vi "TC-4.59.22-backup.vi"() -> ()   [LabVIEW 2019]
uses:
  1. Sources/Lib/Lib.llb/CS mode.ctl
  1. Sources/Lib/Lib.llb/R.ctl
  1. Sources/Lib/Lib.llb/T.ctl
  1. Sources/Lib/Lib.llb/Calibrations.ctl
  1. Sources/Lib/Lib.llb/CS.lvclass
  1. Sources/Lib/Lib.llb/PID Settings.ctl
  1. Sources/Lib/Lib.llb/AVS_exc_n_ranges.ctl
  1. Sources/Lib/Lib.llb/AVS_excitation.ctl
  1. Sources/Lib/Lib.llb/AVS47_range.ctl
  1. Sources/Lib/Lib.llb/Ch descriptions.ctl
  1. Sources/Lib/Lib.llb/Cursor Controls.ctl
  1. Sources/Lib/Lib.llb/DataArray.ctl
  1. Sources/Lib/Lib.llb/Unit.ctl
  1. Sources/Lib/Lib.llb/Control 6.ctl
  1. Sources/Lib/Lib.llb/Control 4.ctl
  1. Sources/Lib/Lib.llb/Control 8.ctl
  1. Sources/Lib/Lib.llb/VI FPO Ref.ctl
  1. Sources/Lib/support/Class ID ENUM.ctl
  <userlib>/_OpenG.lib/lvdata/lvdata.llb/Type Descriptor Enumeration__ogtk.ctl
  <userlib>/_OpenG.lib/lvdata/lvdata.llb/Refnum Subtype Enum__ogtk.ctl
  <userlib>/_OpenG.lib/lvdata/lvdata.llb/Waveform Subtype Enum__ogtk.ctl
  1. Sources/Lib/Lib.llb/LV Data cluster.ctl
  1. Sources/Lib/Lib.llb/Action.ctl
  1. Sources/Lib/Lib.llb/TCS.lvclass
  C:/Users/patrick/Documents/GitHub/Leiden-FP-and-TC/src/TC/1. Sources/Lib/Lib.llb/CS.lvclass
  1. Sources/Lib/Lib.llb/QCS.lvclass
  1. Sources/Lib/Lib.llb/CS Emulation.lvclass
  1. Sources/Lib/Lib.llb/PCS.lvclass
  1. Sources/Lib/Lib.llb/Byte Params.ctl
  1. Sources/Lib/Lib.llb/MView.lvlib
  shared/FP-TC-Shared/FP-TC-Shared.lvclass
panel:
  out "R Array":dbl[](array[numeric])
  out "_SetControl":T1
  out "ControlNames":string[](array[string])
  out "VIRef":T2 {"Array DataType" format="%.0x"; "WaveForm Type" format="%.0x"; "RefNum Type" format="%.0x"; "DataType" format="%.0x"}
  out "VI called?":bool=TRUE
  out "Error code":u8
  out "_zBridgeSetNr":u8 caption="zBridge set nr."
  out "_zBridgeDll":path=path "C:/Users/Sasha/Dropbox/Labview/LC Software/ImpSoft-V5.2.2-multithreaded/ImpBridgeLabview/ImpBridgeDll.dll"
  in  "_String":string="^ Click the Run button to start the program "
  in  "Top Toolbar":enum32{"Page 1", "Page 2"}(tab)
  in  "Load config":bool
  in  "Start":bool
  in  "Load Data":bool
  in  "Pause":bool
  in  "Stop":bool
  in  "Copy to Clipboard":bool
  in  "Save config":bool
  in  "Clear all plots":bool
  in  "ColorBox":enum32{"Page 1", "Page 2"}(tab)
  in  "Colors":picture
  out "Color":u32(colorbox)
  in  "Graph-open popup":bool
  out "_CalibFilesPath":path=path "C:/avs-47/aaaa"
  out "_LogFilesPath":path
  out "_AVS_VISA":refnum<visa-resource-name>="COM3"
  out "VI Version":string="TC" caption="V"
  in  "Minimize UI 2":bool
  in  "Minimize UI 1":bool
  in  "Main Panel":enum32{"AVS"}(tab)
  in  "Graph Controls Bar":enum32{"Page 1"}(tab)
  in  "Mode Buttons":T7
  in  "Erase all":bool
  in  "Plot-Save All":bool
  in  "Plot-save-screen":bool
  in  "Channels Panel":T8(tab)=enum."All"
  out "T0":dbl=nan caption="T" format="%#.2p"
  out "R0":dbl caption="R" format="%.3p"
  out "R-Plot 0":cluster{dbl[], dbl[]}(graph) caption="R-Plot"
  out "T1":dbl=nan caption="T" format="%#.2p"
  out "R1":dbl caption="R" format="%.3p"
  out "R-Plot 1":cluster{dbl[], dbl[]}(graph) caption="R-Plot"
  out "T2":dbl=nan caption="T" format="%#.2p"
  out "R2":dbl caption="R" format="%.3p"
  out "R-Plot 2":cluster{dbl[], dbl[]}(graph) caption="R-Plot"
  out "T3":dbl=nan caption="T" format="%#.2p"
  out "R3":dbl caption="R" format="%.3p"
  out "R-Plot 3":cluster{dbl[], dbl[]}(graph) caption="R-Plot"
  out "T4":dbl=nan caption="T" format="%#.2p"
  out "R4":dbl caption="R" format="%.3p"
  out "R-Plot 4":cluster{dbl[], dbl[]}(graph) caption="R-Plot"
  out "T5":dbl=nan caption="T" format="%#.2p"
  out "R5":dbl caption="R" format="%.3p"
  out "R-Plot 5":cluster{dbl[], dbl[]}(graph) caption="R-Plot"
  out "T6":dbl=nan caption="T" format="%#.2p"
  out "R6":dbl caption="R" format="%.3p"
  out "R-Plot 6":cluster{dbl[], dbl[]}(graph) caption="R-Plot"
  out "T7":dbl=nan caption="T" format="%#.2p"
  out "R7":dbl caption="R" format="%.3p"
  out "R-Plot 7":cluster{dbl[], dbl[]}(graph) caption="R-Plot"
  out "T8":dbl=nan caption="T" format="%#.2p"
  out "R8":dbl caption="R" format="%.3p"
  out "R-Plot 8":cluster{dbl[], dbl[]}(graph) caption="R-Plot"
  out "T9":dbl=nan caption="T" format="%#.2p"
  out "R9":dbl caption="R" format="%.3p"
  out "R-Plot 9":cluster{dbl[], dbl[]}(graph) caption="R-Plot"
  out "T Cluster":T9 {"T9" format="%.2p"; "T8" format="%.2p"; "T7" format="%.2p"; "T6" format="%.2p"; "T5" format="%.2p"; "T4" format="%.2p"; "T3" format="%.2p"; "T2" format="%.2p"; "T1" format="%.2p"; "T0" format="%.2p"}
  in  "Sensor Names":T10={"AVS Name 0"="C_still", "AVS Name 1"="3K", "AVS Name 2"="Still", "AVS Name 3"="50mK", "AVS Name 4"="MC", "AVS Name 5"="MC", "AVS Name 6"="MC", "AVS Name 7"="", "AVS Name 8"="", "AVS Name 9"=""}
  in  "Edit Calibrations":T11
  in  "Sensor Calibrations":T12 {"Sensor 10" items=["magnet", "No Calibration", "PT100", "PT1000", "RuO2 10k", "RuO2 1k5", "RuO2 2k", "switch", "Emulation R", "PT 1000", "RuO2-10K-NEW", "RuO2-10K", "RuO2-1k5", "TT-1338", "TT-1340", "TT-1342", "TT-1346", "TT-1349", "TT-1392", "CMN-187", "testCMN", "No Calibration"]; "Sensor 9" items=["magnet", "No Calibration", "PT100", "PT1000", "RuO2 10k", "RuO2 1k5", "RuO2 2k", "switch", "Emulation R", "PT 1000", "RuO2-10K-NEW", "RuO2-10K", "RuO2-1k5", "TT-1338", "TT-1340", "TT-1342", "TT-1346", "TT-1349", "TT-1392", "CMN-187", "testCMN", "No Calibration"]; "Sensor 8" items=["magnet", "No Calibration", "PT100", "PT1000", "RuO2 10k", "RuO2 1k5", "RuO2 2k", "switch", "Emulation R", "PT 1000", "RuO2-10K-NEW", "RuO2-10K", "RuO2-1k5", "TT-1338", "TT-1340", "TT-1342", "TT-1346", "TT-1349", "TT-1392", "CMN-187", "testCMN", "No Calibration"]; "Sensor 7" items=["magnet", "No Calibration", "PT100", "PT1000", "RuO2 10k", "RuO2 1k5", "RuO2 2k", "switch", "Emulation R", "PT 1000", "RuO2-10K-NEW", "RuO2-10K", "RuO2-1k5", "TT-1338", "TT-1340", "TT-1342", "TT-1346", "TT-1349", "TT-1392", "CMN-187", "testCMN", "No Calibration"]; "Sensor 6" items=["magnet", "No Calibration", "PT100", "PT1000", "RuO2 10k", "RuO2 1k5", "RuO2 2k", "switch", "Emulation R", "PT 1000", "RuO2-10K-NEW", "RuO2-10K", "RuO2-1k5", "TT-1338", "TT-1340", "TT-1342", "TT-1346", "TT-1349", "TT-1392", "CMN-187", "testCMN", "No Calibration"]; "Sensor 5" items=["magnet", "No Calibration", "PT100", "PT1000", "RuO2 10k", "RuO2 1k5", "RuO2 2k", "switch", "Emulation R", "PT 1000", "RuO2-10K-NEW", "RuO2-10K", "RuO2-1k5", "TT-1338", "TT-1340", "TT-1342", "TT-1346", "TT-1349", "TT-1392", "CMN-187", "testCMN", "No Calibration"]; "Sensor 4" items=["magnet", "No Calibration", "PT100", "PT1000", "RuO2 10k", "RuO2 1k5", "RuO2 2k", "switch", "Emulation R", "PT 1000", "RuO2-10K-NEW", "RuO2-10K", "RuO2-1k5", "TT-1338", "TT-1340", "TT-1342", "TT-1346", "TT-1349", "TT-1392", "CMN-187", "testCMN", "No Calibration"]; "Sensor 3" items=["magnet", "No Calibration", "PT100", "PT1000", "RuO2 10k", "RuO2 1k5", "RuO2 2k", "switch", "Emulation R", "PT 1000", "RuO2-10K-NEW", "RuO2-10K", "RuO2-1k5", "TT-1338", "TT-1340", "TT-1342", "TT-1346", "TT-1349", "TT-1392", "CMN-187", "testCMN", "No Calibration"]; "Sensor 2" items=["magnet", "No Calibration", "PT100", "PT1000", "RuO2 10k", "RuO2 1k5", "RuO2 2k", "switch", "Emulation R", "PT 1000", "RuO2-10K-NEW", "RuO2-10K", "RuO2-1k5", "TT-1338", "TT-1340", "TT-1342", "TT-1346", "TT-1349", "TT-1392", "CMN-187", "testCMN", "No Calibration"]; "Sensor 1" items=["magnet", "No Calibration", "PT100", "PT1000", "RuO2 10k", "RuO2 1k5", "RuO2 2k", "switch", "Emulation R", "PT 1000", "RuO2-10K-NEW", "RuO2-10K", "RuO2-1k5", "TT-1338", "TT-1340", "TT-1342", "TT-1346", "TT-1349", "TT-1392", "CMN-187", "testCMN", "No Calibration"]}
  out "Units":T13
  out "R Cluster":T14={"R0"=0.0, "R1"=0.0, "R2"=-0.0, "R3"=0.0, "R4"=0.0, "R5"=0.0, "R6"=0.0, "R7"=0.0, "R8"=0.0, "R9"=0.0} {"R9" format="%.3p"; "R8" format="%.3p"; "R7" format="%.3p"; "R6" format="%.3p"; "R5" format="%.3p"; "R4" format="%.3p"; "R3" format="%.3p"; "R2" format="%.3p"; "R1" format="%.3p"; "R0" format="%.3p"}
  in  "AVS Scan Parameters":enum32{"Page 1", "Page 2"}(tab)
  in  "AVS Exc&Ranges":T15={"Excitation 0"=4, "Excitation 1"=4, "Excitation 2"=3, "Excitation 3"=3, "Excitation 4"=3, "Excitation 5"=3, "Excitation 6"=3, "Excitation 7"=3, "Range 0"=5, "Range 1"=5, "Range 2"=5, "Range 3"=5, "Range 4"=5, "Range 5"=5, "Range 6"=5, "Range 7"=5} {"Range 7" items=["n.a."=-1, "open"=0, "2 Ohm"=1, "20 Ohm"=2, "200 Ohm"=3, "2k Ohm"=4, "20k Ohm"=5, "200k Ohm"=6, "2M Ohm"=7]; "Range 6" items=["n.a."=-1, "open"=0, "2 Ohm"=1, "20 Ohm"=2, "200 Ohm"=3, "2k Ohm"=4, "20k Ohm"=5, "200k Ohm"=6, "2M Ohm"=7]; "Range 5" items=["n.a."=-1, "open"=0, "2 Ohm"=1, "20 Ohm"=2, "200 Ohm"=3, "2k Ohm"=4, "20k Ohm"=5, "200k Ohm"=6, "2M Ohm"=7]; "Range 4" items=["n.a."=-1, "open"=0, "2 Ohm"=1, "20 Ohm"=2, "200 Ohm"=3, "2k Ohm"=4, "20k Ohm"=5, "200k Ohm"=6, "2M Ohm"=7]; "Range 3" items=["n.a."=-1, "open"=0, "2 Ohm"=1, "20 Ohm"=2, "200 Ohm"=3, "2k Ohm"=4, "20k Ohm"=5, "200k Ohm"=6, "2M Ohm"=7]; "Range 2" items=["n.a."=-1, "open"=0, "2 Ohm"=1, "20 Ohm"=2, "200 Ohm"=3, "2k Ohm"=4, "20k Ohm"=5, "200k Ohm"=6, "2M Ohm"=7]; "Range 1" items=["n.a."=-1, "open"=0, "2 Ohm"=1, "20 Ohm"=2, "200 Ohm"=3, "2k Ohm"=4, "20k Ohm"=5, "200k Ohm"=6, "2M Ohm"=7]; "Range 0" items=["n.a."=-1, "open"=0, "2 Ohm"=1, "20 Ohm"=2, "200 Ohm"=3, "2k Ohm"=4, "20k Ohm"=5, "200k Ohm"=6, "2M Ohm"=7]; "Excitation 7" items=["none", "3 µV", "10 µV", "30 µV", "100 µV", "300 µV", "1 mV", "3 mV"]; "Excitation 6" items=["none", "3 µV", "10 µV", "30 µV", "100 µV", "300 µV", "1 mV", "3 mV"]; "Excitation 5" items=["none", "3 µV", "10 µV", "30 µV", "100 µV", "300 µV", "1 mV", "3 mV"]; "Excitation 4" items=["none", "3 µV", "10 µV", "30 µV", "100 µV", "300 µV", "1 mV", "3 mV"]; "Excitation 3" items=["none", "3 µV", "10 µV", "30 µV", "100 µV", "300 µV", "1 mV", "3 mV"]; "Excitation 2" items=["none", "3 µV", "10 µV", "30 µV", "100 µV", "300 µV", "1 mV", "3 mV"]; "Excitation 1" items=["none", "3 µV", "10 µV", "30 µV", "100 µV", "300 µV", "1 mV", "3 mV"]; "Excitation 0" items=["none", "3 µV", "10 µV", "30 µV", "100 µV", "300 µV", "1 mV", "3 mV"]}
  out "zBridge.Scan Phase":T18
  out "zBridge params":T19
  out "uPlots":T20
  out "zBridge.Active Channels":T21={"active Channel 0"=TRUE, "active Channel 1"=TRUE, "active Channel 2"=TRUE, "active Channel 3"=FALSE, "active Channel 4"=FALSE, "active Channel 5"=FALSE, "active Channel 6"=FALSE, "active Channel 7"=FALSE, "active Channel 8"=FALSE, "active Channel 9"=FALSE}
  out "Waveform Chart":T22(graph)
  in  "_CS_Address":u32
  in  "Edit calibration":bool
  in  "Convert R-T":bool
  out "T7":dbl caption="T=" format="%#.2p"
  in  "QuickR":dbl caption="R=" format="%_6g"
  in  "_QuickConvertCal":u16(ring) items=["magnet", "No Calibration", "PT100", "PT1000", "RuO2 10k", "RuO2 1k5", "RuO2 2k", "switch", "Emulation R", "PT 1000", "RuO2-10K-NEW", "RuO2-10K", "RuO2-1k5", "TT-1338", "TT-1340", "TT-1342", "TT-1346", "TT-1349", "TT-1392", "CMN-187", "testCMN", "No Calibration"]
  out "_CSMode1List[i]":T23[](array[typedef]) caption="I_list[i]" min=-1.0
  out "CS.Automode Current":T23[](array[typedef]) min=-1.0
  in  "Lower Panel":enum32{"Page 1", "Page 2"}(tab)
  in  "Data History/RT Settings":enum32{"History", "Settings"}(tab)=enum."Settings"
  out "AVS names small":T10={"AVS Name 0"="3K", "AVS Name 1"="Still", "AVS Name 2"="50 mK", "AVS Name 3"="MC", "AVS Name 4"="MC", "AVS Name 5"="", "AVS Name 6"="", "AVS Name 7"="", "AVS Name 8"="", "AVS Name 9"=""}
  out "zBridge.Active channel":T24
  out "Small T Cluster":T25 caption="T" {"T0" format="%#.2p"; "T1" format="%#.2p"; "T2" format="%#.2p"; "T3" format="%#.2p"; "T4" format="%#.2p"; "T5" format="%#.2p"; "T6" format="%#.2p"; "T7" format="%#.2p"; "T8" format="%#.2p"; "T9" format="%#.2p"}
  out "Small R Cluster":T26 caption="R" {"R0" format="%#_5p"; "R1" format="%#_5p"; "R2" format="%#_5p"; "R3" format="%#_5p"; "R4" format="%#_5p"; "R5" format="%#_5p"; "R6" format="%#_5p"; "R7" format="%#_5p"; "R8" format="%#_5p"; "R9" format="%#_5p"}
  out "Time":dbl format="%<%X\n%x>T"
  in  "Runtime Settings":T27={"Read AVS channels from"=0, "Last Channel"=7, "Delay Between Scans"=0, "Stabilisation Delay"=5.0, "Averages"=2, "Data Memory"=25000, "Filter Graphs"=FALSE, "Y_min"=0.0, "Y_max"=2000000.0, "Plot type"=enum."T vs Time", "Allow neg R"=TRUE, "Miniplot Time"=30.0} {"Miniplot Time" min=0.0; "Delay Between Scans" format="%.0f s"; "Averages" min=1 max=1000; "Stabilisation Delay" min=0.5; "Last Channel" min=0 max=7 step=1; "Read AVS channels from" min=0 max=7 step=1; "Y_max" format="%#_6f"; "Y_min" min=0.0 format="%#_6f"; "Data Memory" min=3 max=50000}
  out "CS.Current Value":dbl[](array[numeric])
  in  "Data Array":T28=[{"R"=[], "T"=[], "Time"=[]}, {"R"=[0.0, 2.0], "T"=[], "Time"=[]}]
  out "T Array":dbl[](array[numeric])
  in  "_ScanData":dbl[](array[numeric])
  out "_I3SetPnt":dbl
  out "_CurrentsChanged":bool
  in  "_AVSRanges":T29={"Excitationl 0"=5, "Excitation 1"=5, "Excitation 2"=5, "Excitation 3"=5, "Excitation 4"=5, "Excitation 5"=5, "Excitation 6"=5, "Excitation 7"=5} caption="Ranges" {"Excitation 7" items=["n.a."=-1, "open"=0, "2 Ohm"=1, "20 Ohm"=2, "200 Ohm"=3, "2k Ohm"=4, "20k Ohm"=5, "200k Ohm"=6, "2M Ohm"=7]; "Excitation 6" items=["n.a."=-1, "open"=0, "2 Ohm"=1, "20 Ohm"=2, "200 Ohm"=3, "2k Ohm"=4, "20k Ohm"=5, "200k Ohm"=6, "2M Ohm"=7]; "Excitation 5" items=["n.a."=-1, "open"=0, "2 Ohm"=1, "20 Ohm"=2, "200 Ohm"=3, "2k Ohm"=4, "20k Ohm"=5, "200k Ohm"=6, "2M Ohm"=7]; "Excitation 4" items=["n.a."=-1, "open"=0, "2 Ohm"=1, "20 Ohm"=2, "200 Ohm"=3, "2k Ohm"=4, "20k Ohm"=5, "200k Ohm"=6, "2M Ohm"=7]; "Excitation 3" items=["n.a."=-1, "open"=0, "2 Ohm"=1, "20 Ohm"=2, "200 Ohm"=3, "2k Ohm"=4, "20k Ohm"=5, "200k Ohm"=6, "2M Ohm"=7]; "Excitation 2" items=["n.a."=-1, "open"=0, "2 Ohm"=1, "20 Ohm"=2, "200 Ohm"=3, "2k Ohm"=4, "20k Ohm"=5, "200k Ohm"=6, "2M Ohm"=7]; "Excitation 1" items=["n.a."=-1, "open"=0, "2 Ohm"=1, "20 Ohm"=2, "200 Ohm"=3, "2k Ohm"=4, "20k Ohm"=5, "200k Ohm"=6, "2M Ohm"=7]; "Excitationl 0" items=["n.a."=-1, "open"=0, "2 Ohm"=1, "20 Ohm"=2, "200 Ohm"=3, "2k Ohm"=4, "20k Ohm"=5, "200k Ohm"=6, "2M Ohm"=7]}
  out "_CSClassRef":refnum<class "CS.lvclass">
  in  "CS Indicators Panel":enum32{"Page 1", "Page 2"}(tab)
  out "CS.Automode 0":bool
  out "CS.Automode 1":bool
  out "QCS. I0 Mapping":T30(ring) caption="Output to"
  in  "uA 0":u32
  in  "CS Cannel Names":T31={"CS Name 0"="N.C.", "CS Name 1"="3K", "CS Name 2"="Still", "CS Name 3"="MC"}
  out "I0":T32={"uA"="000", "ON"=FALSE, "Gated"=FALSE, "current flows"=FALSE, "Error"=FALSE} caption="Ch0 -"
  in  "uA 3":u32
  in  "uA 2":u32
  in  "uA 1":u32
  out "CS.Automode 3":bool
  out "CS.Automode 2":bool
  out "I3":T32={"uA"="000", "ON"=FALSE, "Gated"=FALSE, "current flows"=FALSE, "Error"=FALSE} caption="Chn 3"
  out "I2":T32={"uA"="000", "ON"=FALSE, "Gated"=FALSE, "current flows"=FALSE, "Error"=FALSE} caption="Chn 2"
  out "I1":T32={"uA"="000", "ON"=FALSE, "Gated"=FALSE, "current flows"=FALSE, "Error"=FALSE} caption="Chn 1"
  out "_ExtVIReference":refnum<vi>
  out "Small I":cluster{"I1":dbl, "I2":dbl, "I3":dbl, "I4":dbl} caption="I" {"I1" format="%#.2f"; "I2" format="%#.2p"; "I3" format="%#.2p"; "I4" format="%#.2p"}
  out "CS.Actual Current":dbl[](array[numeric])
  in  "Save Data 2":bool
  in  "Show PID graph?":bool
  in  "Set Color":bool
  out "_ZBridgeUnit":string caption="Unit"
  out "_zBridgeParText":string caption="zBridge params/Error"
  out "_CurCalibrations":T33
  out "_LMBDown":bool
  in  "Side Panel":T34(tab)
  in  "Reload Calibrations":bool
  in  "zBridge settings":bool
  out "CS.ID":string
  out "CS status":errorcluster
  out "General Error":errorcluster caption="General status"
  in  "Bridge settings":T35={"Bridge Type"=enum."AVS47A (GPIB interface)", "AVS RS232 Port"="COM5", "AVS GPIB Address"="GPIB0::20::INSTR", "Calibrations Folder"=path "C:/LC Data/Calibrations"}
  in  "CS Settings":T36={"TCS RS232 Port"="COM1", "TCS_Imax"=5, "CS type"=enum."TCS", "CS.QCS Device Nr"=0}
  in  "Data Logging Settings":T37={"Log Files Folder"=path "C:/LC Data/Data", "Log Files Name"="LogAVS", "Automode Files Name"="calibration", "Filenames Suffix"="_%Y-%m-%d-%H-%M-%S", "Delimeter"="\t", "New File Interval"=7, "New File Interval Units"=enum."Days", "Date Format"="%Y-%m-%d %H:%M:%S", "External VI Path"=path "", "Query Description"=FALSE, "Run Description"="\n"}
  out "Bridge status":errorcluster
  in  "CS.QCS I0 Output":T38(ring) caption="Set Channel 0 output to"
  in  "CS.Mode":T39 caption="CS mode"
  out "_TimeOld":dbl format="%#_16g"
  in  "CS Modes Panel":T40(tab)=enum."Automatic 1"
  in  "CS.I3":T41={"Toggle ON/OFF"=FALSE, "Toggle Gated"=FALSE, "I"=0, "Range"=enum."x1 uA"} caption="Chn 3" {"I" max=100000 step=1}
  in  "CS.I2":T41={"Toggle ON/OFF"=FALSE, "Toggle Gated"=FALSE, "I"=0, "Range"=enum."x1 uA"} caption="Chn 2" {"I" max=100000 step=1}
  in  "CS.I1":T41={"Toggle ON/OFF"=FALSE, "Toggle Gated"=FALSE, "I"=0, "Range"=enum."x1 uA"} caption="Chn 1" {"I" max=100000 step=1}
  in  "CS.I0":T41={"Toggle ON/OFF"=FALSE, "Toggle Gated"=FALSE, "I"=0, "Range"=enum."x1 uA"} caption="Chn 0" {"I" max=100000 step=1}
  in  "CS.Mode1.PID Settings":T42={"FB on 2"=enum."3", "Proportional Gain"=3.0, "Integral Gain"=3.0, "Derivative Gain"=1.0, "Deadband"=0.1, "Feed Fwd Gain [uA/mK]"=0.0, "Integral Gain Bandwidth"=10.0, "Integral Gain Background"=1.0, "Current limit, [uA]"=1.0} {"Integral Gain Background" format="%#.6g"; "Integral Gain Bandwidth" format="%#.6g"; "Feed Fwd Gain [uA/mK]" format="%#.5g"; "Deadband" format="%#.5g"; "Derivative Gain" format="%#.6g"; "Integral Gain" format="%#.6g"; "Proportional Gain" format="%#.6g"; "Current limit, [uA]" format="%#.5g"}
  in  "CS.Mode1.Start":bool
  in  "CS.Mode1.List":T23[][](array[typedef]) min=-1.0
  out "CS.Mode1.PID Column":T43[](array[typedef])
  out "CS.Mode1.Row":T44[](array[typedef])=[TRUE, FALSE, FALSE, FALSE, FALSE, FALSE, FALSE, FALSE, FALSE, FALSE]
  out "CS.Mode1.PID Stabilized?":bool caption="SP reached?"
  out "CS.Mode1.PID Error":dbl=10.0 caption="Error" format="%#_6f"
  out "CS.Mode1.Slope":dbl caption="Slope" format="%#_3g %"
  out "CS.Mode1.Timer":dbl caption="Timer" format="%<%H:%M:%S>t"
  out "CS.Mode1.List:Count":i32=10 caption="/"
  out "CS.Mode1.List:Index":i32=10 caption="Point #"
  in  "CS.Mode1.Next":bool
  in  "CS.Mode1.Reset PID":bool
  in  "CS.Mode1.Auto Advance":bool=TRUE caption="Enable automatic sweeping/list iteration"
  in  "CS.Mode1.Settings":T45={"Bridge Channel"=0, "N averages"=10, "Delay Time"=10.0, "T stability"=0.3, "FB on"=enum."Temperature"} {"Delay Time" min=0.0 format="%#_g min"; "Bridge Channel" min=-1 max=9 step=1}
  in  "CS.Mode1.Call VI?":bool caption="Call Ext. VI"
  out "CS.Mode1.VI State":T46(ring) caption="- state"
  in  "CS.Mode1.Trigger all TC":bool caption="Trigger other running TC instances"
  in  "CS.Mode1.List:Prev":bool
  in  "CS.Mode1.List:Next":bool
  in  "CS.Mode1.List:To First":bool
  in  "CS.Mode1.List:Save":bool
  in  "CS.Mode1.List:Load":bool
  in  "CS.Mode1.Write To Log":bool
  in  "CS.Mode1.PID":cluster{"Enabled":bool}
  in  "CS.Mode1.List:Clear":bool
  in  "CS.Mode2.Settings":T47={"FB on"=enum."Temperature", "Bridge Channel"=0, "Hysteresis"=10} {"Hysteresis" max=100 format="%.0f %%"; "Bridge Channel" min=-1 max=9 step=1}
  in  "CS.Mode2.Start":bool
  in  "CS.Mode2.Add Row":bool
  in  "CS.Mode2.New Row":dbl[](array[numeric])=[0.0, 0.0, 0.0, 0.0, 0.0, 0.0] caption="New range" min=-1.0
  in  "CS.Mode2.List":dbl[][](array[numeric])=[[0.0, 0.0, 0.0, 0.0, 0.0, inf]] min=-1.0
  out "CS.Mode2.Row":T44[](array[typedef])=[TRUE, FALSE, FALSE, FALSE, FALSE, FALSE, FALSE, FALSE, FALSE, FALSE]
  in  "T Sweep":T48={"Start value"=200.0, "End value"=250.0, "Step"=10.0, "Current"=0.0, "I_next"=FALSE, "I_prev"=FALSE, "Interrrupt Sweep"=FALSE, "Start"=FALSE, "Boolean"=TRUE} {"Step" min=0.0; "End value" min=0.0; "Start value" min=0.0}
  # "Quick convert R->T:"
  # "Ohm"
  # "mK"
  # "Ch#"
  # "Miniplot"
  # "Channel parameters"
  # "Impedance"
  # "Unit"
  # "Type of sensor"
  # "T [mK]"
  # "Description"
  # "0"
  # "1"
  # "2"
  # "3"
  # "4"
  # "5"
  # "6"
  # "7"
  # "8"
  # "9"
  # "0"
  # "1"
  # "2"
  # "3"
  # "4"
  # "5"
  # "7"
  # "8"
  # "9"
  # "6"
  # "auto"
  # "auto"
  # "auto"
  # "auto"
  # "gated"
  # "gated"
  # "gated"
  # "gated"
  # "Status"
  # "Current source mode"
  # "Current source manual control"
  # "Current source automatic mode #1"
  # "Currents List"
  # "Settings"
  # "I0"
  # "I1"
  # "I2"
  # "I3"
  # "Status"
  # "On temperature stabilized"
  # "Current source automatic mode #2"
  # "Currents List"
  # "Settings"
  # "T0"
  # "T1"
  # "I0"
  # "I1"
  # "I2"
  # "I3"
  # "T0"
  # "T1"
  # "I0"
  # "I1"
  # "I2"
  # "I3"
  # "Ch3"
types:
  T1 = typedef "MView.lvlib/LV Data cluster.ctl" = cluster{"Name":string, "Scalar":string, "Array":string[][]}
  T2 = typedef "MView.lvlib/VI FPO Ref.ctl" = cluster{"Control Ref ID":refnum<vi>[], "Full Name":string[], "ClassID":T3[], "Short Name":string[], "DataType":T4[], "RefNum Type":T5[], "WaveForm Type":T6[], "Parent":i32[], "Array DataType":T4[], "Owning VI":refnum<vi>[], "Active?":bool[]}
  T3 = typedef "Class ID ENUM.ctl" = enum16{"<Null>", "1", "2", "Generic", "Decoration", "Text", "Control", "ColorBox", "Boolean", "RefNum", "Variant", "Path", "ListBox", "Table", "Array", "Picture", "ActiveXContainer", "Numeric", "Digital", "NamedNumeric", "ColorRamp", "Slide", "GraphOrChart", "WaveformChart", "WaveformGraph", "IntensityChart", "IntensityGraph", "String", "IOName", "ComboBox", "Cluster", "Panel", "Knob", "NumWithScale", "Ring", "Enum", "GObject", "Plot", "Cursor", "NumericText", "Scale", "ColorScale", "GraphScale", "ColorGraphScale", "TypedRefNum", "OldKnobScale", "MCListbox", "MeasureData", "BVTag", "DAQName", "VISAName", "IVIName", "SlideScale", "TabControl", "Page", "TabArrayTabControl", "ConPane", "57", "58", "59", "60", "61", "62", "63", "64", "SubPanel", "TreeControl", "67", "68", "69", "70", "71", "72", "73", "74", "75", "SplitterBar"}
  T4 = typedef "Type Descriptor Enumeration__ogtk.ctl" = enum8{"<Null>", "I8", "I16", "I32", "I64", "U8", "U16", "U32", "U64", "SGL", "DBL", "EXT", "CSG", "CDB", "CXT", "0x0F", "0x10", "0x11", "0x12", "0x13", "0x14", "Enum U8", "Enum U16", "Enum U32", "Enum U64", "SGL PQ", "DBL PQ", "EXT PQ", "CSG PQ", "CDB PQ", "CXT PQ", "0x1F", "0x20", "Boolean", "0x22", "0x23", "0x24", "0x25", "0x26", "0x27", "0x28", "0x29", "0x2A", "0x2B", "0x2C", "0x2D", "0x2E", "0x2F", "String", "0x31", "Path", "Pict", "0x34", "0x35", "0x36", "DAQ", "0x38", "0x39", "0x3A", "0x3B", "0x3C", "0x3D", "0x3E", "0x3F", "Array", "0x41", "0x42", "0x43", "0x44", "0x45", "0x46", "0x47", "0x48", "0x49", "0x4A", "0x4B", "0x4C", "0x4D", "0x4E", "0x4F", "Cluster", "0x51", "0x52", "Variant", "Waveform", "0x55", "0x56", "0x57", "0x58", "0x59", "0x5A", "0x5B", "0x5C", "0x5D", "0x5E", "Fixed Point", "0x60", "0x61", "0x62", "0x63", "0x64", "0x65", "0x66", "0x67", "0x68", "0x69", "0x6A", "0x6B", "0x6C", "0x6D", "0x6E", "0x6F", "Refnum", "0x71", "0x72", "Set Collection", "Map Collection"}
  T5 = typedef "Refnum Subtype Enum__ogtk.ctl" = enum8{"Generic", "Datalog File Refnum", "Byte Stream File Refnum", "Device Refnum", "Occurence Refnum", "TCP Connection Refnum", "VISA Refnum (Obsolete)", "Automation Renum", "VI Server Refnum", "Menu Refnum", "IVI Refnum (Obsolete)", "IMAQ Session", "0x0C", "Datasocket Refnum", "VISA Resource", "IVI Logical Name", "UDP Connection Refnum", "Notifier Refnum", "Queue Refnum", "IrDA Refnum", "Hardware Plugin Refnum", "Hardware Plugin Tag Refnum", "DAQmx Refnum", "Event Registration Refnum", ".NET Refnum", "User Event Refnum", "0x1A", "Event Callback", "0x1C", "0x1D", "LabVIEW Class Instance", "Bluetooth", "Data Value References", "RT FIFO", "TDM Streaming"}
  T6 = typedef "Waveform Subtype Enum__ogtk.ctl" = enum8{"<Not a Waveform Type>", "0x01", "Analog 16-bit signed", "Analog Double-Precision", "0x04", "Analog Single Precision", "Timestamp", "Digital Data", "Digital Waveform", "Dynamic Data", "Analog Extended-Precision", "Analog 8-bit unsigned", "Analog 16-bit unsigned", "Analog 32-bit unsigned", "Analog 8-bit signed", "Analog 32-bit signed", "Analog Complex Single-Precision", "Analog Complex Double-Precision", "Analog Complex Extended Precision", "Analog 64-bit signed", "Analog 64-bit unsigned"}
  T7 = typedef "Cursor Controls.ctl" = enum32{"No Selection", "Cursor mode", "Erase point", "Erase range"}
  T8 = enum32{"0", "1", "2", "3", "4", "5", "6", "7", "8", "9", "All", "PID loop"}
  T9 = typedef "T.ctl" = cluster{"T0":dbl, "T1":dbl, "T2":dbl, "T3":dbl, "T4":dbl, "T5":dbl, "T6":dbl, "T7":dbl, "T8":dbl, "T9":dbl}
  T10 = typedef "Ch descriptions.ctl" = cluster{"AVS Name 0":string, "AVS Name 1":string, "AVS Name 2":string, "AVS Name 3":string, "AVS Name 4":string, "AVS Name 5":string, "AVS Name 6":string, "AVS Name 7":string, "AVS Name 8":string, "AVS Name 9":string}
  T11 = cluster{"Boolean":bool, "Boolean 2":bool, "Boolean 3":bool, "Boolean 4":bool, "Boolean 5":bool, "Boolean 6":bool, "Boolean 7":bool, "Boolean 8":bool, "Boolean 9":bool, "Boolean 10":bool}
  T12 = typedef "Calibrations.ctl" = cluster{"Sensor 1":u16, "Sensor 2":u16, "Sensor 3":u16, "Sensor 4":u16, "Sensor 5":u16, "Sensor 6":u16, "Sensor 7":u16, "Sensor 8":u16, "Sensor 9":u16, "Sensor 10":u16}
  T13 = typedef "Unit.ctl" = cluster{"Value 0":string, "Value 1":string, "Value 2":string, "Value 3":string, "Value 4":string, "Value 5":string, "Value 6":string, "Value 7":string, "Value 8":string, "Value 9":string}
  T14 = typedef "R.ctl" = cluster{"R0":dbl, "R1":dbl, "R2":dbl, "R3":dbl, "R4":dbl, "R5":dbl, "R6":dbl, "R7":dbl, "R8":dbl, "R9":dbl}
  T15 = typedef "AVS_exc_n_ranges.ctl" = cluster{"Excitation 0":T16, "Excitation 1":T16, "Excitation 2":T16, "Excitation 3":T16, "Excitation 4":T16, "Excitation 5":T16, "Excitation 6":T16, "Excitation 7":T16, "Range 0":T17, "Range 1":T17, "Range 2":T17, "Range 3":T17, "Range 4":T17, "Range 5":T17, "Range 6":T17, "Range 7":T17}
  T16 = typedef "AVS_excitation.ctl" = i16
  T17 = typedef "AVS47_range.ctl" = i16
  T18 = cluster{"Value 0":dbl, "Value 1":dbl, "Value 2":dbl, "Value 3":dbl, "Value 4":dbl, "Value 5":dbl, "Value 6":dbl, "Value 7":dbl, "Value 8":dbl, "Value 9":dbl}
  T19 = cluster{"AVS Name 0":string, "AVS Name 1":string, "AVS Name 2":string, "AVS Name 3":string, "AVS Name 4":string, "AVS Name 5":string, "AVS Name 6":string, "AVS Name 7":string, "AVS Name 8":string, "AVS Name 9":string}
  T20 = cluster{"uPlot 0":cluster{dbl[], dbl[]}, "uPlot 1":cluster{dbl[], dbl[]}, "uPlot 2":cluster{dbl[], dbl[]}, "uPlot 3":cluster{dbl[], dbl[]}, "uPlot 4":cluster{dbl[], dbl[]}, "uPlot 5":cluster{dbl[], dbl[]}, "uPlot 6":cluster{dbl[], dbl[]}, "uPlot 7":cluster{dbl[], dbl[]}, "uPlot 8":cluster{dbl[], dbl[]}, "uPlot 9":cluster{dbl[], dbl[]}}
  T21 = cluster{"active Channel 0":bool, "active Channel 1":bool, "active Channel 2":bool, "active Channel 3":bool, "active Channel 4":bool, "active Channel 5":bool, "active Channel 6":bool, "active Channel 7":bool, "active Channel 8":bool, "active Channel 9":bool}
  T22 = cluster{"Ip":dbl, "Ii":dbl, "Id":dbl, "Iff":dbl, "I_tot":dbl}
  T23 = typedef "Control 4.ctl" = dbl
  T24 = cluster{"Boolean 5":bool, "Boolean 5":bool, "Boolean 5":bool, "Boolean 5":bool, "Boolean 5":bool, "Boolean 5":bool, "Boolean 5":bool, "Boolean 5":bool, "Boolean 5":bool, "Boolean 5":bool}
  T25 = cluster{"T0":dbl, "T1":dbl, "T2":dbl, "T3":dbl, "T4":dbl, "T5":dbl, "T6":dbl, "T7":dbl, "T8":dbl, "T9":dbl}
  T26 = cluster{"R0":dbl, "R1":dbl, "R2":dbl, "R3":dbl, "R4":dbl, "R5":dbl, "R6":dbl, "R7":dbl, "R8":dbl, "R9":dbl}
  T27 = cluster{"Read AVS channels from":i8, "Last Channel":i8, "Delay Between Scans":u32, "Stabilisation Delay":dbl, "Averages":u16, "Data Memory":u16, "Filter Graphs":bool, "Y_min":dbl, "Y_max":dbl, "Plot type":enum16{"R vs Time", "T vs Time"}, "Allow neg R":bool, "Miniplot Time":dbl}
  T28 = typedef "DataArray.ctl" = cluster{"R":dbl[], "T":dbl[], "Time":dbl[]}[]
  T29 = cluster{"Excitationl 0":i16, "Excitation 1":i16, "Excitation 2":i16, "Excitation 3":i16, "Excitation 4":i16, "Excitation 5":i16, "Excitation 6":i16, "Excitation 7":i16}
  T30 = enum16{"Chn 0", "Aux 0", "Aux 1", "Aux 2", "Aux 3"}
  T31 = cluster{"CS Name 0":string, "CS Name 1":string, "CS Name 2":string, "CS Name 3":string}
  T32 = cluster{"uA":string, "ON":bool, "Gated":bool, "current flows":bool, "Error":bool}
  T33 = cluster{"[0]":string, "[1]":string, "[2]":string, "[3]":string, "[4]":string, "[5]":string, "[6]":string, "[7]":string, "[8]":string, "[9]":string}
  T34 = enum32{"Devices Settings", "Current source control"}
  T35 = cluster{"Bridge Type":enum16{"AVS47A (GPIB interface)", "AVS47B (RS232 interface)", "AVS48SI (RS232 interface)", "AVS Emulation", "Impedance Bridge", "Disabled"}, "AVS RS232 Port":refnum<visa-resource-name>, "AVS GPIB Address":refnum<visa-resource-name>, "Calibrations Folder":path}
  T36 = cluster{"TCS RS232 Port":refnum<visa-resource-name>, "TCS_Imax":i32, "CS type":enum16{"TCS", "QCS v1", "PCS (n.a.)", "CS Emulation", "Disabled"}, "CS.QCS Device Nr":u16}
  T37 = cluster{"Log Files Folder":path, "Log Files Name":string, "Automode Files Name":string, "Filenames Suffix":string, "Delimeter":string, "New File Interval":u32, "New File Interval Units":enum16{"Minutes", "Hours", "Days"}, "Date Format":string, "External VI Path":path, "Query Description":bool, "Run Description":string}
  T38 = enum16{"Channel 0", "Aux 0", "Aux 1", "Aux 2", "Aux 3"}
  T39 = typedef "CS mode.ctl" = enum16{"Manual", "Mode 1", "Mode2"}
  T40 = enum32{"Manual", "Automatic 1", "Automatic 2", "Automatic 3"}
  T41 = cluster{"Toggle ON/OFF":bool, "Toggle Gated":bool, "I":u32, "Range":enum8{"Auto", "x1 uA", "x10 uA", "x100 uA", "x1 mA"}}
  T42 = typedef "PID Settings.ctl" = cluster{"FB on 2":enum16{"0", "1", "2", "3"}, "Proportional Gain":dbl, "Integral Gain":dbl, "Derivative Gain":dbl, "Deadband":dbl, "Feed Fwd Gain [uA/mK]":dbl, "Integral Gain Bandwidth":dbl, "Integral Gain Background":dbl, "Current limit, [uA]":dbl}
  T43 = typedef "Control 8.ctl" = bool
  T44 = typedef "Control 6.ctl" = bool
  T45 = cluster{"Bridge Channel":i32, "N averages":i32, "Delay Time":dbl, "T stability":dbl, "FB on":enum16{"Resistance", "Temperature"}}
  T46 = enum32{"Bad", "Idle", "Run top level", "Running"}
  T47 = cluster{"FB on":enum16{"Resistance", "Temperature"}, "Bridge Channel":i32, "Hysteresis":u8}
  T48 = cluster{"Start value":dbl, "End value":dbl, "Step":dbl, "Current":dbl, "I_next":bool, "I_prev":bool, "Interrrupt Sweep":bool, "Start":bool, "Boolean":bool}
  T49 = cluster{"UpdateChannelInfo":refnum<user-event>, "UpdateValuesAVS":refnum<user-event>, "UpdateCalibrations":refnum<user-event>, "UpdateLogFilePath":refnum<user-event>, "TempStabilized":refnum<user-event>, "Reset PID loop":refnum<user-event>, "UpdateValuesZBridge":refnum<user-event>, "CS Automode":refnum<user-event>, "CallExtVI":refnum<user-event>, "Data Array":refnum<user-event>}
  T50 = cluster{"Config folder":path, "Config File":path, "Calibrations Folder":path, "zBridge dll":path, "Variables Library":path}
  T51 = enum32{"Page Enabled", "Page Disabled", "Page Disabled & Grayed"}
  T52 = cluster{"error":bool, "code":i32, "source":string}
  T53 = typedef "Action.ctl" = enum16{"Init", "Write", "Read"}
  T54 = enum32{"No Selection", "Cursor mode", "Erase point", "Erase range"}
  T55 = enum16{"AVS47A (GPIB interface)", "AVS47B (RS232 interface)", "AVS48", "AVS Emulation", "Impedance Bridge", "Disabled"}
  T56 = enum16{"TCS", "QCS v1", "PCS (n.a.)", "CS Emulation", "Disabled"}
  T57 = enum8{"Auto", "x1 uA", "x10 uA", "x100 uA", "x1 mA"}
  T58 = cluster{"Cluster":cluster{"Time":dbl[], "T":dbl[]}, "Cluster":cluster{"Time":dbl[], "T":dbl[]}, "Cluster":cluster{"Time":dbl[], "T":dbl[]}, "Cluster":cluster{"Time":dbl[], "T":dbl[]}, "Cluster":cluster{"Time":dbl[], "T":dbl[]}, "Cluster":cluster{"Time":dbl[], "T":dbl[]}, "Cluster":cluster{"Time":dbl[], "T":dbl[]}, "Cluster":cluster{"Time":dbl[], "T":dbl[]}, "Cluster":cluster{"Time":dbl[], "T":dbl[]}, "Cluster":cluster{"Time":dbl[], "T":dbl[]}}
  T59 = enum32{"invalid app kind", "Development System", "Run Time System", "Student Edition", "Embedded LabVIEW", "Evaluation", "Custom"}
  T60 = enum16{"AVS47A (GPIB interface)", "AVS47B (RS232 interface)", "AVS48SI (RS232 interface)", "AVS Emulation", "Impedance Bridge", "Disabled"}
  T61 = cluster{"[0]":dbl, "[1]":dbl, "[2]":dbl, "[3]":dbl, "[4]":dbl, "[5]":dbl, "[6]":dbl, "[7]":dbl, "[8]":dbl, "[9]":dbl}
  T62 = cluster{"Temperature[0]":dbl, "Temperature[1]":dbl, "Temperature[2]":dbl, "Temperature[3]":dbl, "Temperature[4]":dbl, "Temperature[5]":dbl, "Temperature[6]":dbl, "Temperature[7]":dbl, "Temperature[8]":dbl, "Temperature[9]":dbl}
  T63 = cluster{"Current Time (double)":dbl, "R":dbl[], "T":dbl[]}
  T64 = typedef "File Info Record__ogtk.ctl" = cluster{"type":string, "creator":string, "permissions":i32, "data size":i32, "res size":i32, "creation date":u32, "modification date":u32, "bFolder":bool, "bInvisible":bool, "location":cluster{"vertical":i16, "horizontal":i16}, "owner":string, "group":string}
  T65 = cluster{"Units[0]":string, "Units[1]":string, "Units[2]":string, "Units[3]":string, "Units[4]":string, "Units[5]":string, "Units[6]":string, "Units[7]":string, "Units[8]":string, "Units[9]":string}
  T66 = cluster{"zBridge params[0]":string, "zBridge params[1]":string, "zBridge params[2]":string, "zBridge params[3]":string, "zBridge params[4]":string, "zBridge params[5]":string, "zBridge params[6]":string, "zBridge params[7]":string, "zBridge params[8]":string, "zBridge params[9]":string}
  T67 = cluster{"date/time string":string, "Value":dbl[], "Value":dbl[], "Value":dbl[]}
  T68 = typedef "imagedata.ctl" = cluster{"image type":i32, "image depth":i32, "image":u8[], "mask":u8[], "colors":u32[], "Rectangle":cluster{"left":i16, "top":i16, "right":i16, "bottom":i16}}
  T69 = typedef "LVPoint32TypeDef.ctl" = cluster{"Horizontal":i32, "Vertical":i32}
  T70 = cluster{"Shift":bool, "Ctrl":bool, "Alt":bool, "Cmd":bool, "Opt":bool}
  T71 = cluster{"Output Array":dbl[], "array w/ subset deleted":dbl[], "array w/ subset deleted":dbl[]}
  T72 = typedef "LVRectTypeDef.ctl" = cluster{"Left":i16, "Top":i16, "Right":i16, "Bottom":i16}
  T73 = typedef "Exc_n_Ranges.ctl" = cluster{"Excitationl 0":i16, "Excitation 1":i16, "Excitation 2":i16, "Excitation 3":i16, "Excitation 4":i16, "Excitation 5":i16, "Excitation 6":i16, "Excitation 7":i16, "Range 0":i16, "Range 1":i16, "Range 2":i16, "Range 3":i16, "Range 4":i16, "Range 5":i16, "Range 6":i16, "Range 7":i16}
  T74 = enum32{"HKEY_CLASSES_ROOT", "HKEY_CURRENT_USER", "HKEY_LOCAL_MACHINE", "HKEY_USERS", "HKEY_PERFORMANCE_DATA", "HKEY_CURRENT_CONFIG", "HKEY_DYN_DATA"}
  T75 = typedef "Byte Params.ctl" = enum8{"Active", "Channel Type", "Channel No", "Reference No", "RLC select", "Save Data", "L Inverted", "Menu Active"}
  T76 = typedef "LVPositionTypeDef.ctl" = cluster{"Left":i32, "Top":i32}
  T77 = cluster{"Range 0":i16, "Range 1":i16, "Range 2":i16, "Range 3":i16, "Range 4":i16, "Range 7":i16, "Range 5":i16, "Range 6":i16}
  T78 = cluster{"Range 0":i16, "Range 1":i16, "Range 2":i16, "Range 3":i16, "Range 4":i16, "Range 5":i16, "Range 6":i16, "Range 7":i16}
  T79 = cluster{"RANGE 0":u16, "RANGE 1":u16, "RANGE 2":u16, "RANGE 3":u16, "RANGE 4":u16, "RANGE 5":u16, "RANGE 6":u16, "RANGE 7":u16}
  T80 = typedef "LCR Channel parameters.ctl" = cluster{"Set_number":u8, "Set_char":u16, "Ch_number":u8, "Ch_type":u8, "Freq":dbl, "T_int":dbl, "I_exc":dbl, "V_exc":dbl, "SNR":dbl, "Vnoise":dbl, "P_diss":dbl}
  T81 = typedef "CS Data.ctl" = cluster{"Range":u8, "Current":dbl, "Current (string)":string, "On?":bool, "G?":bool, "I?":bool, "Err?":bool}
  T82 = typedef "TCS indicator.ctl" = cluster{"uA":string, " ON":bool, "Gated":bool, "current flows":bool, "Error":bool}
  T83 = cluster{"Toggle ON/OFF":bool, "Toggle Gated":bool}
  T84 = cluster{"Current":u32, "Range":enum16{"Auto", "x1 uA", "x10 uA", "x100 uA", "x1 mA"}}
  T85 = typedef "TCS manual control.ctl" = cluster{"Toggle ON/OFF":bool, "Toggle Gated":bool, "Current":u32, "Range":enum8{"Auto", "x1 uA", "x10 uA", "x100 uA", "x1 mA"}}
  T86 = cluster{"Status[0]":i32, "Status[1]":i32, "Status[2]":i32, "Status[3]":i32, "Status[4]":i32, "Status[5]":i32, "Status[6]":i32, "Status[7]":i32, "Status[8]":i32, "Status[9]":i32}
  T87 = cluster{"Active":bool, "Active":bool, "Active":bool, "Active":bool, "Active":bool, "Active":bool, "Active":bool, "Active":bool, "Active":bool, "Active":bool}
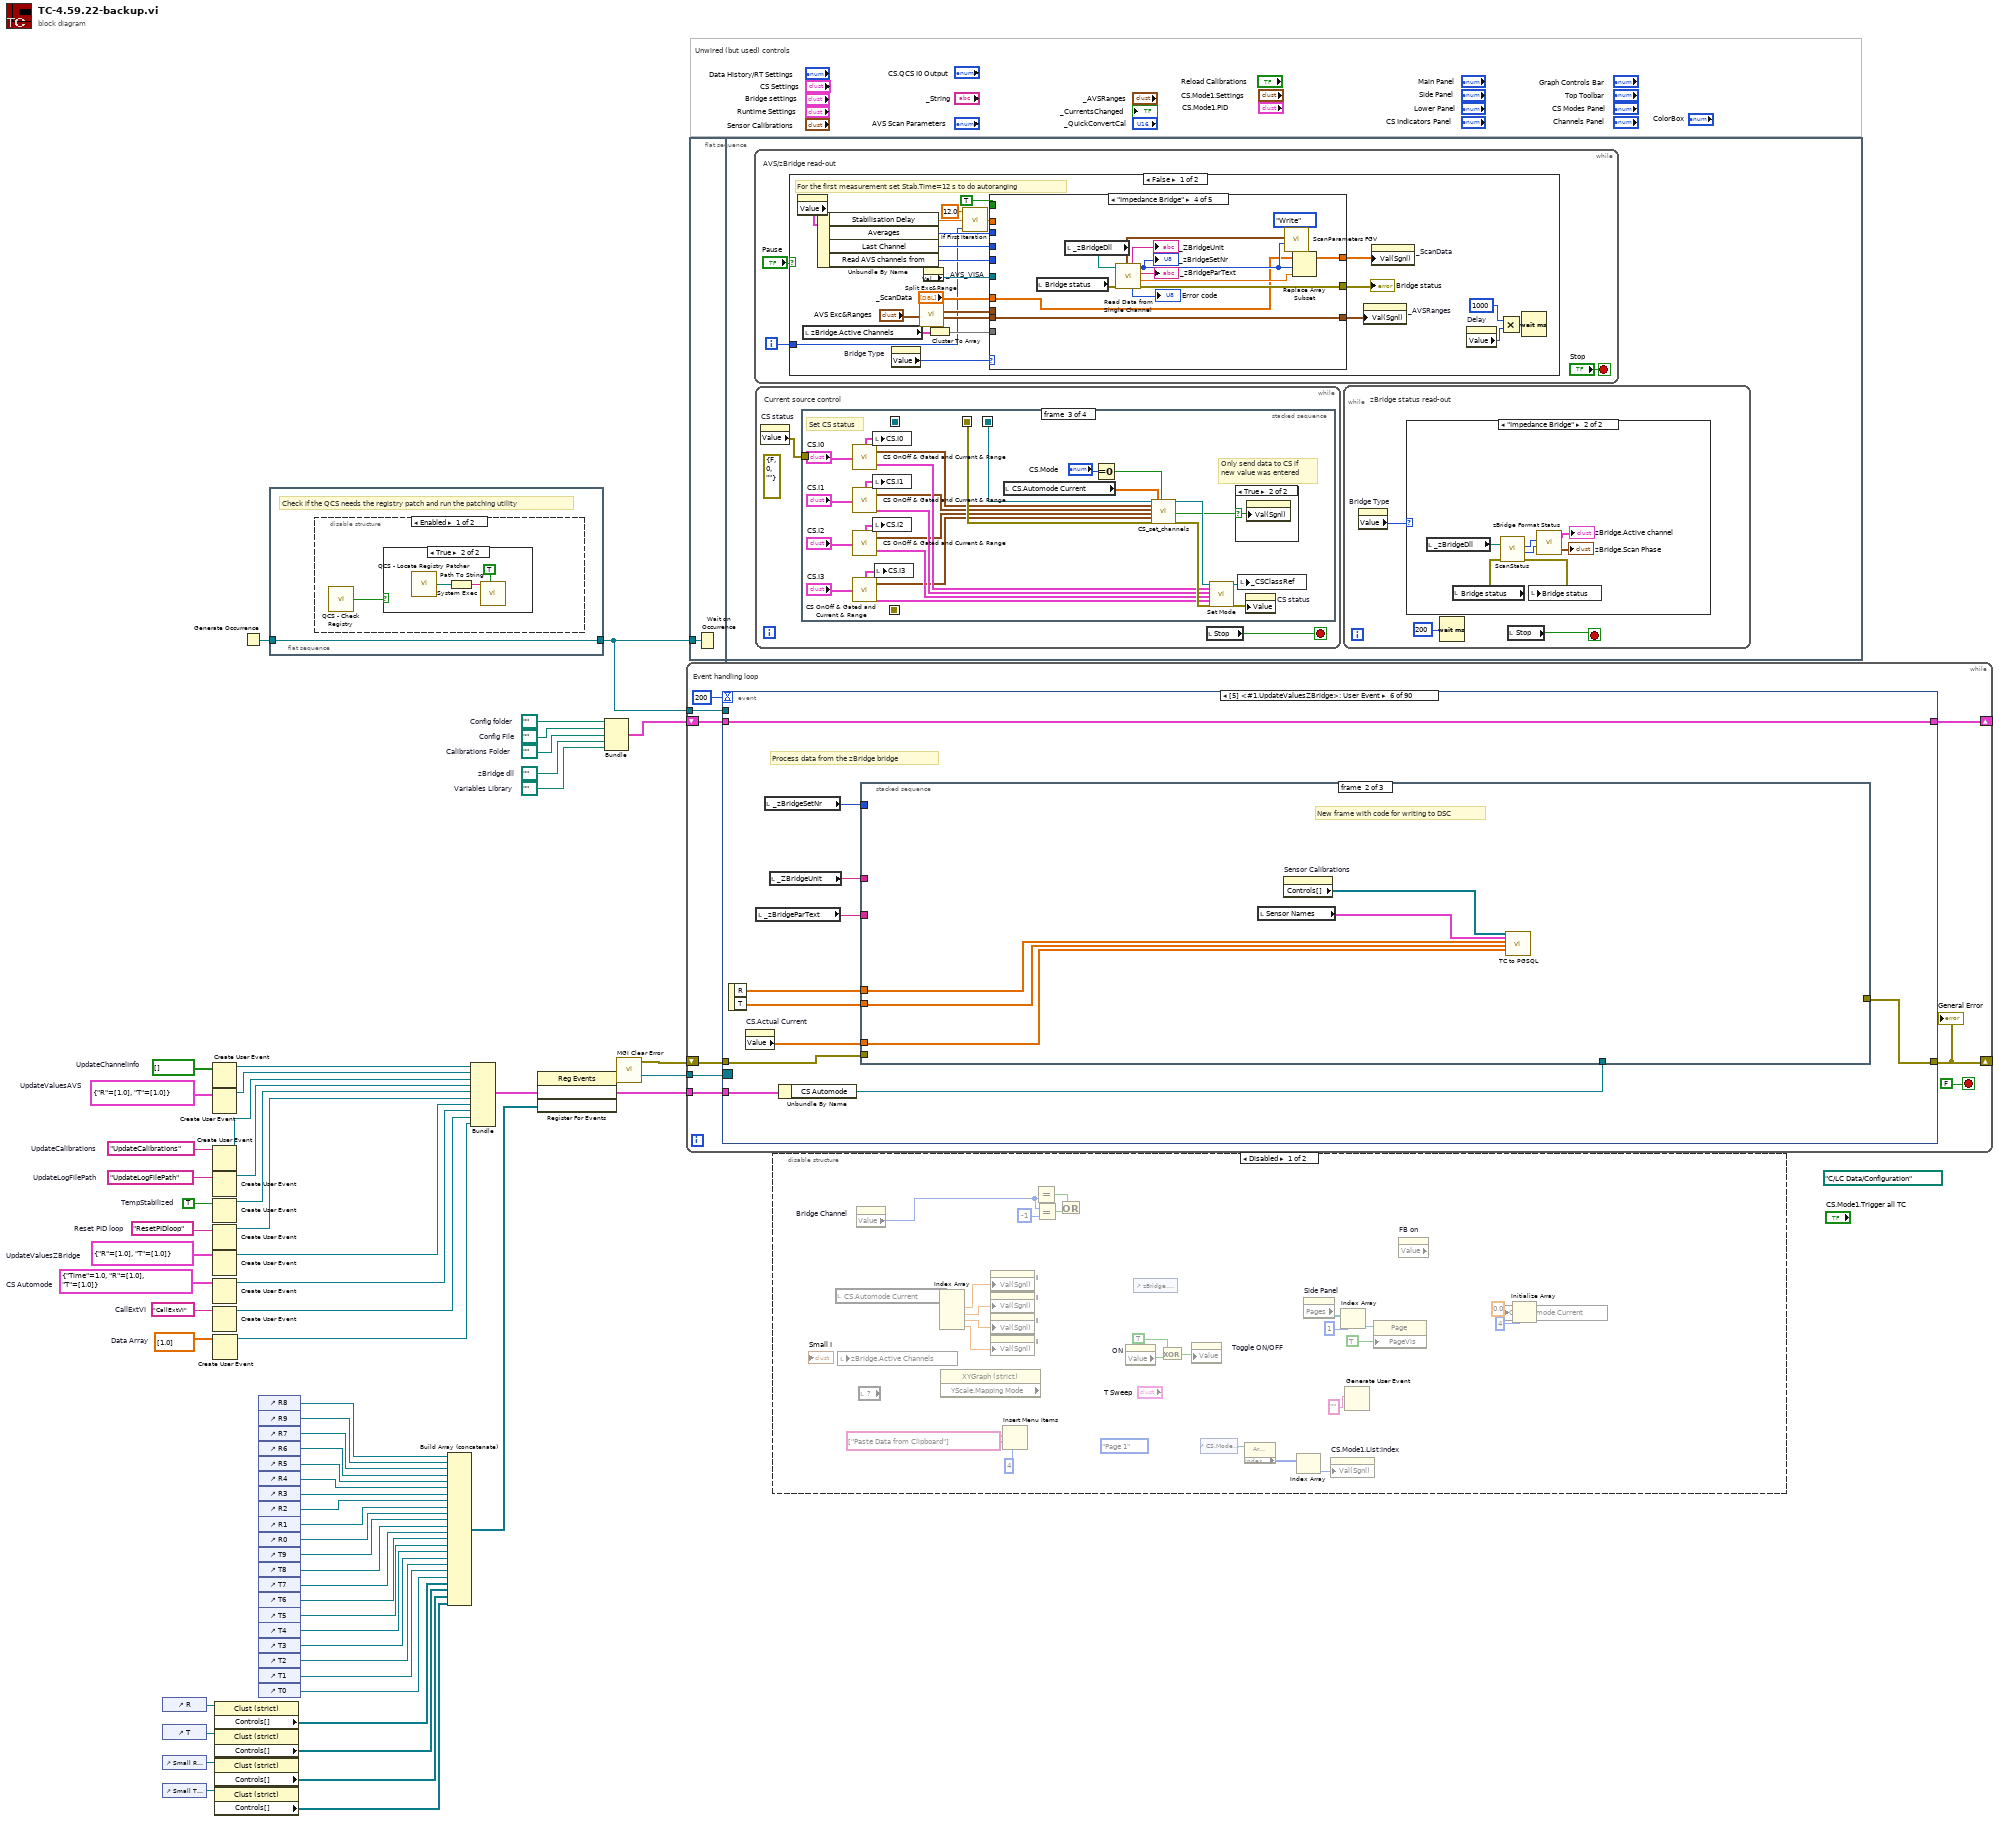
[diagram p0: block diagram]
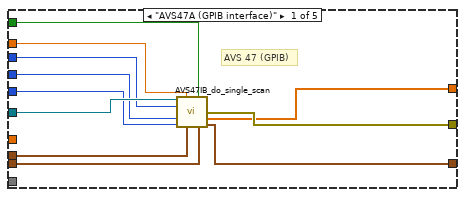
[diagram p5: hidden frame]
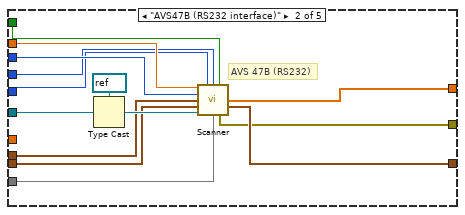
[diagram p6: hidden frame]
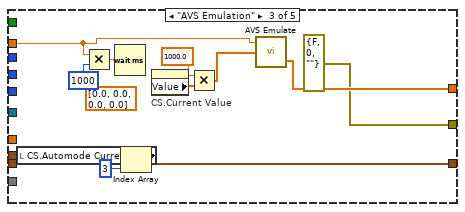
[diagram p7: hidden frame]
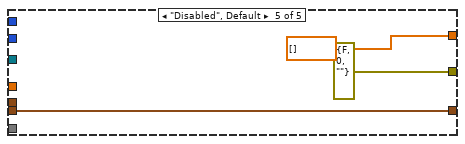
[diagram p8: hidden frame]
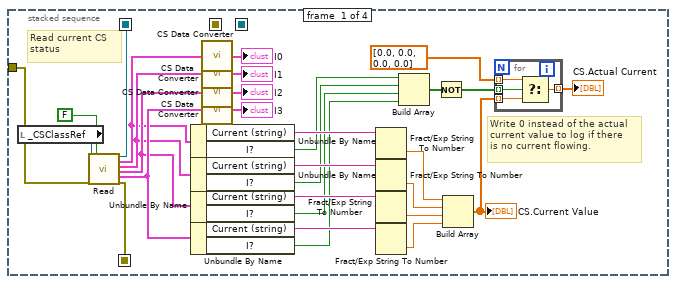
[diagram p10: hidden frame]
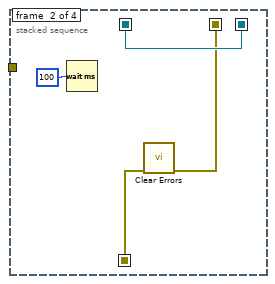
[diagram p11: hidden frame]
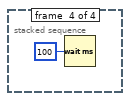
[diagram p13: hidden frame]
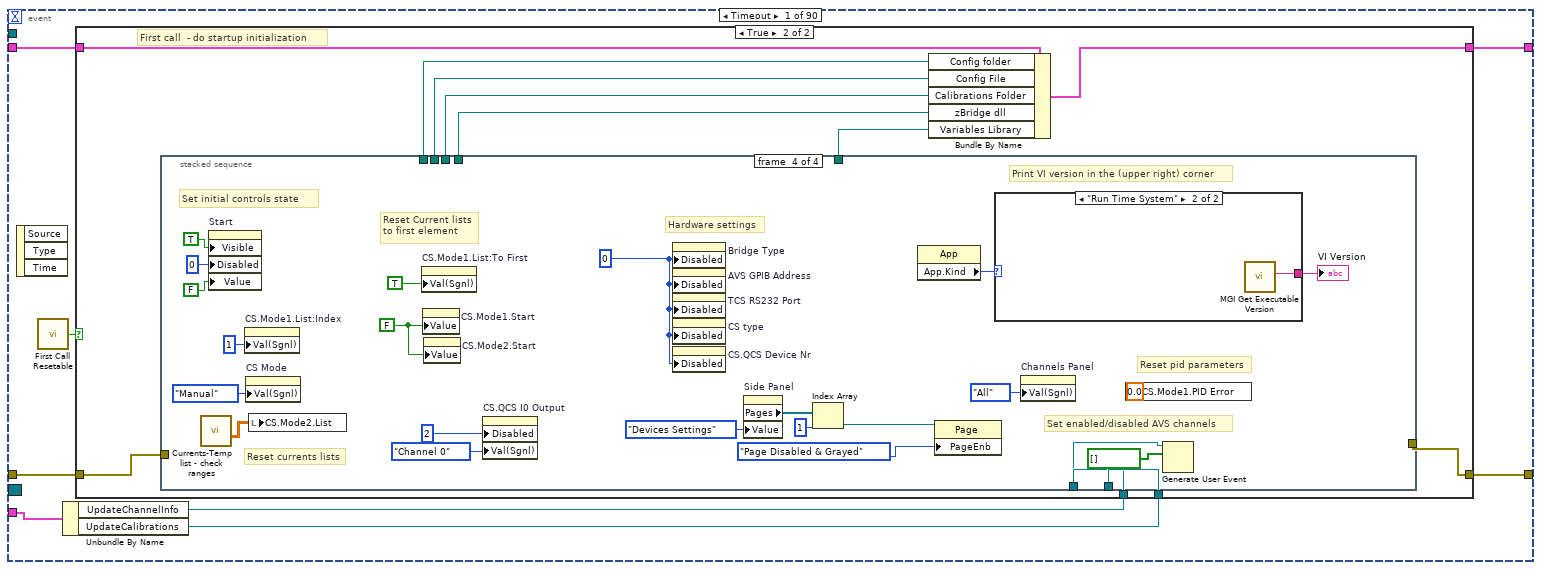
[diagram p15: hidden frame]
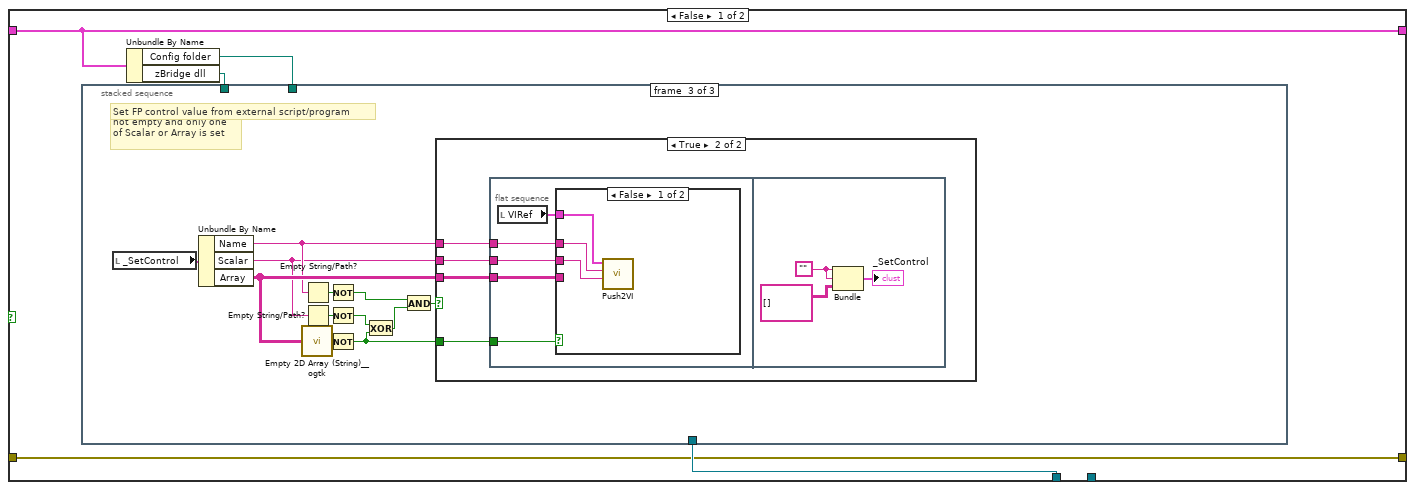
[diagram p16: hidden frame]
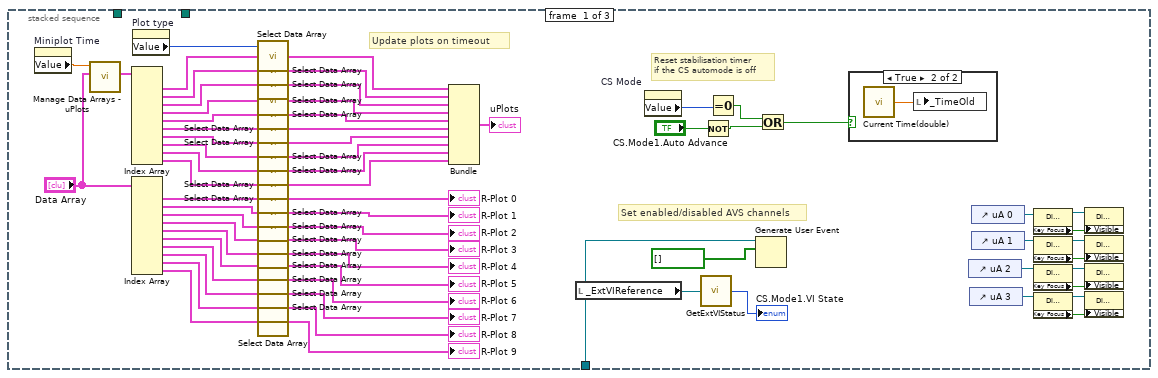
[diagram p17: hidden frame]
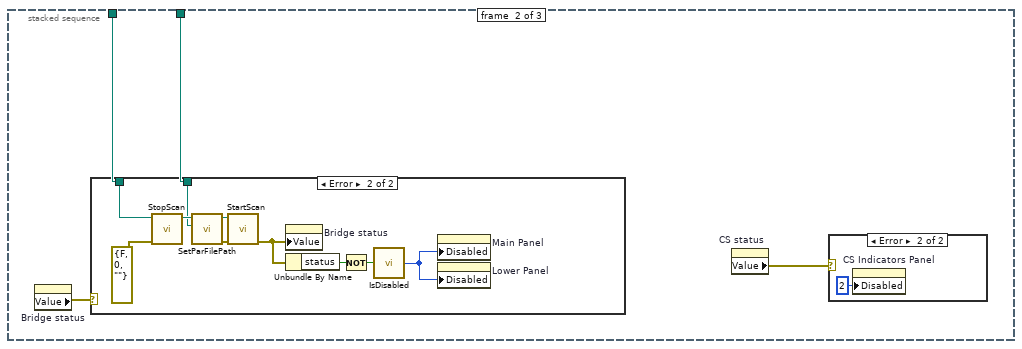
[diagram p19: hidden frame]
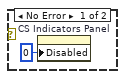
[diagram p20: hidden frame]
diagram:
  w30 = path ""  # Variables Library
  w31 = path ""  # zBridge dll
  w32 = path ""  # Calibrations Folder
  w33 = path ""  # Config File
  w35 = path ""  # Config folder
  (unwired) path "C:/LC Data/Configuration" ("Relative path (.)")
  w38 = dbl[] [1.0]  # Data Array
  w52 = "CallExtVI"  # CallExtVI
  w53 = bool[] []  # UpdateChannelInfo
  w54 = cluster{"Time":dbl, "R":dbl[], "T":dbl[]} {"Time"=1.0, "R"=[1.0], "T"=[1.0]}  # CS Automode
  w55 = cluster{"R":dbl[], "T":dbl[]} {"R"=[1.0], "T"=[1.0]}  # UpdateValuesAVS
  w56 = cluster{"R":dbl[], "T":dbl[]} {"R"=[1.0], "T"=[1.0]}  # UpdateValuesZBridge
  w57 = "ResetPIDloop"  # Reset PID loop
  w58 = TRUE  # TempStabilized
  w59 = "UpdateLogFilePath"  # UpdateLogFilePath
  w60 = "UpdateCalibrations"  # UpdateCalibrations
  # "Unwired (but used) controls"
  n1 = control-ref of="R"() -> (w29:refnum<vi>)
  n2 = control-ref of="T"() -> (w28:refnum<vi>)
  n3 = control-ref of="Small R Cluster"() -> (w4:refnum<vi>)
  n4 = control-ref of="Small T Cluster"() -> (w3:refnum<vi>)
  n5 = Create User Event(user event datatype=w53) -> (user event=w50:refnum<user-event>)  [unwired: 1 in, 1 out]
  n6 = Create User Event(user event datatype=w55) -> (user event=w49:refnum<user-event>)  [unwired: 1 in, 1 out]
  n7 = Create User Event(user event datatype=w60) -> (user event=w48:refnum<user-event>)  [unwired: 1 in, 1 out]
  n8 = Create User Event(user event datatype=w59) -> (user event=w47:refnum<user-event>)  [unwired: 1 in, 1 out]
  n9 = Create User Event ("TempStabilized")(user event datatype=w58) -> (user event=w46:refnum<user-event>)  [unwired: 1 in, 1 out]
  n10 = Create User Event(user event datatype=w57) -> (user event=w45:refnum<user-event>)  [unwired: 1 in, 1 out]
  n11 = Create User Event(user event datatype=w56) -> (user event=w44:refnum<user-event>)  [unwired: 1 in, 1 out]
  n12 = Create User Event(user event datatype=w54) -> (user event=w43:refnum<user-event>)  [unwired: 1 in, 1 out]
  n13 = Create User Event(user event datatype=w52) -> (user event=w42:refnum<user-event>)  [unwired: 1 in, 1 out]
  n14 = Create User Event(user event datatype=w38) -> (user event=w39:refnum<user-event>)  [unwired: 1 in, 1 out]
  n15 = property class="Clust (strict)"(reference=w29) -> ("Controls[]"=w7:refnum<vi>[])  [unwired: 1 in, 2 out]
  n16 = property class="Clust (strict)"(reference=w28) -> ("Controls[]"=w6:refnum<vi>[])  [unwired: 1 in, 2 out]
  n17 = property class="Clust (strict)"(reference=w4) -> ("Controls[]"=w2:refnum<vi>[])  [unwired: 1 in, 2 out]
  n18 = property class="Clust (strict)"(reference=w3) -> ("Controls[]"=w1:refnum<vi>[])  [unwired: 1 in, 2 out]
  n19 = Generate Occurrence() -> (w37:refnum<k4>)
  n20 = control-ref of="R8"() -> (w27:refnum<vi>)
  n21 = control-ref of="R9"() -> (w26:refnum<vi>)
  n22 = control-ref of="R7"() -> (w25:refnum<vi>)
  n23 = control-ref of="R6"() -> (w24:refnum<vi>)
  n24 = control-ref of="R5"() -> (w23:refnum<vi>)
  n25 = control-ref of="R4"() -> (w22:refnum<vi>)
  n26 = control-ref of="R3"() -> (w21:refnum<vi>)
  n27 = control-ref of="R2"() -> (w20:refnum<vi>)
  n28 = control-ref of="R1"() -> (w19:refnum<vi>)
  n29 = control-ref of="R0"() -> (w18:refnum<vi>)
  n30 = control-ref of="T9"() -> (w17:refnum<vi>)
  n31 = control-ref of="T8"() -> (w16:refnum<vi>)
  n32 = control-ref of="T7"() -> (w15:refnum<vi>)
  n33 = control-ref of="T6"() -> (w14:refnum<vi>)
  n34 = control-ref of="T5"() -> (w13:refnum<vi>)
  n35 = control-ref of="T4"() -> (w12:refnum<vi>)
  n36 = control-ref of="T3"() -> (w11:refnum<vi>)
  n37 = control-ref of="T2"() -> (w10:refnum<vi>)
  n38 = control-ref of="T1"() -> (w9:refnum<vi>)
  n39 = control-ref of="T0"() -> (w8:refnum<vi>)
  n40 = flat-sequence {
    tunnel: w37 -> [w61]
    tunnel: [w61] -> w36
    frame #0 {
      # "Check if the QCS needs the registry patch and run the patching utility"
      n41 = disable-structure shown="Enabled" {
        frame Enabled {
          n42 = call "QCS - Check Registry.vi"() -> ("QCS needs reset?"=w62:bool)  [unwired: 5 in]
          n43 = case shown="True" w62 {
            frame False {
            }
            frame True {
              n44 = call "QCS - Locate Registry Patcher.vi"() -> ("dup path"=w64:path)  [unwired: 5 in]
              n45 = Path To String(path=w64) -> (string=w65:string)
              n46 = call <vilib>:"System Exec.vi"("wait until completion? (T)"=TRUE, "command line"=w65) -> ()  [unwired: 6 in, 4 out]
            }
          }
        }
        frame Disabled {
        }
      }
    }
  }
  n47 = Build Array (concatenate)(w27, w26, w25, w24, w23, w22, w21, w20, w19, w18, w17, w16, w15, w14, w13, w12, w11, w10, w9, w8, w7, w6, w2, w1) -> (w5:refnum<vi>[])
  n48 = Bundle("UpdateChannelInfo"=w50, "UpdateValuesAVS"=w49, "UpdateCalibrations"=w48, "UpdateLogFilePath"=w47, "TempStabilized"=w46, "Reset PID loop"=w45, "UpdateValuesZBridge"=w44, "CS Automode"=w43, "CallExtVI"=w42, "Data Array"=w39) -> (w41:T49)  [unwired: 1 in]
  n49 = register-events(w41, w5) -> (reference out=w51:refnum<event-registration>)  [unwired: 2 in, 1 out]
  n50 = Bundle("Config folder"=w35, "Config File"=w33, "Calibrations Folder"=w32, "zBridge dll"=w31, "Variables Library"=w30) -> (w34:T50)  [unwired: 1 in]
  n51 = call <userlib>:"MGI Clear Error.vi"() -> ("Error Out"=w40:errorcluster)  [unwired: 7 in]
  n52 = while {
    tunnel: w51 -> [w73]
    shift-right: [w70] -> _
    shift-left: w40 -> [w71]
    tunnel: w41 -> [w69]
    tunnel: w36 -> [w68]
    shift-right: [w66] -> _
    shift-left: w34 -> [w67]
    stop <- FALSE stop-if-true
    # "Event handling loop"
    n53 = event shown="[5] <#1.UpdateValuesZBridge>: User Event" {
      selector: w73 -> [_ _ _ _ _ _ _ _ _ _ _ _ _ _ _ _ _ _ _ _ _ _ _ _ _ _ _ _ _ _ _ _ _ _ _ _ _ _ _ _ _ _ _ _ _ _ _ _ _ _ _ _ _ _ _ _ _ _ _ _ _ _ _ _ _ _ _ _ _ _ _ _ _ _ _ _ _ _ _ _ _ _ _ _ _ _ _ _ _ _]
      dyn-events: _ -> [_ _ _ _ _ _ _ _ _ _ _ _ _ _ _ _ _ _ _ _ _ _ _ _ _ _ _ _ _ _ _ _ _ _ _ _ _ _ _ _ _ _ _ _ _ _ _ _ _ _ _ _ _ _ _ _ _ _ _ _ _ _ _ _ _ _ _ _ _ _ _ _ _ _ _ _ _ _ _ _ _ _ _ _ _ _ _ _ _ _]
      timeout: 200 -> [_ _ _ _ _ _ _ _ _ _ _ _ _ _ _ _ _ _ _ _ _ _ _ _ _ _ _ _ _ _ _ _ _ _ _ _ _ _ _ _ _ _ _ _ _ _ _ _ _ _ _ _ _ _ _ _ _ _ _ _ _ _ _ _ _ _ _ _ _ _ _ _ _ _ _ _ _ _ _ _ _ _ _ _ _ _ _ _ _ _]
      tunnel: w71 -> [w82 _ _ w520 w568 w652 _ _ w863 _ _ _ w992 w1001 _ _ _ _ _ _ _ _ _ w1250 _ w1259 _ _ _ _ _ _ _ _ w1364 _ _ _ _ _ _ _ _ _ _ _ _ _ _ _ _ _ _ _ _ _ _ w1790 w1810 _ _ _ _ _ w1955 _ _ _ _ _ _ _ _ _ _ _ _ _ _ _ _ _ _ _ _ _ _ _ _ _]
      tunnel: [w81 _ _ w523 w567 w647 _ _ w861 _ _ _ w991 w1001 _ _ _ _ _ _ _ _ _ w1250 _ w1259 _ _ _ _ _ _ w1346 _ w1364 _ _ _ _ _ _ _ _ _ _ _ _ _ _ _ _ _ _ _ _ _ _ w1789 w1809 _ _ _ _ _ w1955 _ _ _ _ _ _ _ _ _ _ _ _ _ _ _ _ _ _ _ _ _ _ _ _ _] -> w70
      tunnel: w69 -> [w79 _ _ w505 w563 w649 w753 w842 _ _ _ _ _ _ _ _ _ _ _ _ _ _ _ _ _ _ w1290 w1312 _ _ _ _ _ w1354 w1362 _ _ _ _ _ _ _ _ _ _ _ _ _ _ _ _ _ _ _ _ _ _ _ w1804 _ w1885 w1899 _ _ _ _ _ w1961 _ _ w1983 w2000 w2004 _ _ _ _ _ _ _ _ _ _ w2084 _ _ _ _ _ _]
      tunnel: w68 -> [_ w338 _ _ _ _ _ _ _ _ _ _ _ _ _ _ _ _ _ _ _ _ _ _ _ _ _ _ _ _ _ _ _ _ _ _ _ _ _ _ _ _ _ _ _ _ _ _ _ _ _ _ _ _ _ _ _ _ _ _ _ _ _ _ _ _ _ _ _ _ _ _ _ _ _ _ _ _ _ _ _ _ _ _ _ _ _ _ _ _]
      tunnel: w67 -> [w75 w337 w469 w501 w561 w646 w749 w840 w860 w897 w954 w982 w989 w997 w1040 w1057 w1123 w1136 w1176 w1178 w1181 w1194 w1237 w1245 w1253 w1257 w1288 w1310 w1314 w1317 w1325 w1334 w1344 w1352 w1357 w1384 w1388 w1463 w1470 w1477 w1519 w1547 w1581 w1608 w1614 w1622 w1630 w1639 w1648 w1650 w1695 w1703 w1708 w1731 w1748 w1773 w1777 w1781 w1802 w1873 w1883 w1897 w1907 w1932 w1954 w1956 w1957 w1959 w1965 w1969 w1980 w1998 w2002 w2015 w2022 w2023 w2031 w2034 w2038 w2042 w2045 w2071 w2077 w2082 w2086 w2090 w2111 w2123 w2133 w2135]
      tunnel: [w76 w337 w469 w501 w561 w646 w749 w840 w860 w897 w954 w982 w988 w997 w1040 w1057 w1123 w1136 w1176 w1178 w1181 w1194 w1237 w1245 w1253 w1257 w1288 w1310 w1314 w1317 w1325 w1334 w1344 w1352 w1357 w1384 w1388 w1463 w1470 w1477 w1519 w1547 w1581 w1608 w1614 w1622 w1630 w1639 w1648 w1650 w1695 w1703 w1708 w1731 w1748 w1773 w1777 w1781 w1802 w1873 w1883 w1897 w1907 w1932 w1954 w1956 w1957 w1959 w1965 w1969 w1980 w1998 w2002 w2015 w2022 w2023 w2031 w2034 w2038 w2042 w2045 w2071 w2077 w2082 w2086 w2090 w2111 w2123 w2133 w2135] -> w66
      event Timeout {
        n54 = event-data() -> ()  [unwired: 1 in, 3 out]
        n55 = call "First Call Resetable.vi"() -> ("First Call?"=w80:bool)
        n56 = Unbundle By Name(w79) -> ("UpdateChannelInfo"=w77:refnum<user-event>, "UpdateCalibrations"=w78:refnum<user-event>)
        n57 = case shown="True" w80 {
          tunnel: w82 -> [w86 w211]
          tunnel: [w86 w209] -> w81
          tunnel: w78 -> [_ w210]
          tunnel: w77 -> [w87 w208]
          tunnel: w75 -> [w85 w207]
          tunnel: [w85 w206] -> w76
          frame False {
            n58 = Unbundle By Name(w85) -> ("Config folder"=w84:path, "zBridge dll"=w83:path)
            n59 = stacked-sequence {
              tunnel: w87 -> [w88 _ _]
              tunnel: w84 -> [_ w156 _]
              tunnel: w83 -> [_ w155 _]
              frame #0 {
                # "Update plots on timeout"
                # "Set enabled/disabled AVS channels"
                # "Reset stabilisation timer\nif the CS automode is off"
                n60 = property on="Miniplot Time" class="DigNum (strict)"() -> ("Value"=w149:dbl)  [unwired: 2 in, 2 out]
                n61 = call "Manage Data Arrays - uPlots.vi"("Data In"="Data Array", "Data Memory"=w149) -> ("Data Out"=w104:T28)  [unwired: 7 in]
                n62 = Index Array(array=w104) -> (element #1=w119:cluster{"R":dbl[], "T":dbl[], "Time":dbl[]}, element #2=w120:cluster{"R":dbl[], "T":dbl[], "Time":dbl[]}, element #3=w121:cluster{"R":dbl[], "T":dbl[], "Time":dbl[]}, element #4=w122:cluster{"R":dbl[], "T":dbl[], "Time":dbl[]}, element #5=w123:cluster{"R":dbl[], "T":dbl[], "Time":dbl[]}, element #6=w124:cluster{"R":dbl[], "T":dbl[], "Time":dbl[]}, element #7=w125:cluster{"R":dbl[], "T":dbl[], "Time":dbl[]}, element #8=w126:cluster{"R":dbl[], "T":dbl[], "Time":dbl[]}, element #9=w127:cluster{"R":dbl[], "T":dbl[], "Time":dbl[]}, element #10=w128:cluster{"R":dbl[], "T":dbl[], "Time":dbl[]})  [unwired: 10 in]
                n63 = Index Array(array="Data Array") -> (element #1=w148:cluster{"R":dbl[], "T":dbl[], "Time":dbl[]}, element #2=w147:cluster{"R":dbl[], "T":dbl[], "Time":dbl[]}, element #3=w146:cluster{"R":dbl[], "T":dbl[], "Time":dbl[]}, element #4=w145:cluster{"R":dbl[], "T":dbl[], "Time":dbl[]}, element #5=w144:cluster{"R":dbl[], "T":dbl[], "Time":dbl[]}, element #6=w143:cluster{"R":dbl[], "T":dbl[], "Time":dbl[]}, element #7=w142:cluster{"R":dbl[], "T":dbl[], "Time":dbl[]}, element #8=w141:cluster{"R":dbl[], "T":dbl[], "Time":dbl[]}, element #9=w140:cluster{"R":dbl[], "T":dbl[], "Time":dbl[]}, element #10=w139:cluster{"R":dbl[], "T":dbl[], "Time":dbl[]})  [unwired: 10 in]
                n64 = property on="Plot type" class="Enum (strict)"() -> ("Value"=w107:enum16{"R vs Time", "T vs Time"})  [unwired: 2 in, 2 out]
                n65 = call "Select Data Array.vi"("Cluster 2"=w119, "Value"=w107) -> ("Cluster"=w129:cluster{"Time":dbl[], "T":dbl[]})
                n66 = call "Select Data Array.vi"("Cluster 2"=w120, "Value"=w107) -> ("Cluster"=w130:cluster{"Time":dbl[], "T":dbl[]})
                n67 = call "Select Data Array.vi"("Cluster 2"=w121, "Value"=w107) -> ("Cluster"=w131:cluster{"Time":dbl[], "T":dbl[]})
                n68 = call "Select Data Array.vi"("Cluster 2"=w122, "Value"=w107) -> ("Cluster"=w132:cluster{"Time":dbl[], "T":dbl[]})
                n69 = call "Select Data Array.vi"("Cluster 2"=w123, "Value"=w107) -> ("Cluster"=w138:cluster{"Time":dbl[], "T":dbl[]})
                n70 = call "Select Data Array.vi"("Cluster 2"=w124, "Value"=w107) -> ("Cluster"=w133:cluster{"Time":dbl[], "T":dbl[]})
                n71 = call "Select Data Array.vi"("Cluster 2"=w125, "Value"=w107) -> ("Cluster"=w134:cluster{"Time":dbl[], "T":dbl[]})
                n72 = call "Select Data Array.vi"("Cluster 2"=w126, "Value"=w107) -> ("Cluster"=w135:cluster{"Time":dbl[], "T":dbl[]})
                n73 = call "Select Data Array.vi"("Cluster 2"=w127, "Value"=w107) -> ("Cluster"=w136:cluster{"Time":dbl[], "T":dbl[]})
                n74 = call "Select Data Array.vi"("Cluster 2"=w128, "Value"=w107) -> ("Cluster"=w137:cluster{"Time":dbl[], "T":dbl[]})
                n75 = call "Select Data Array.vi"("Cluster 2"=w148, "Value"=w107) -> ("Cluster"=→"R-Plot 0":cluster{"Time":dbl[], "T":dbl[]})
                n76 = call "Select Data Array.vi"("Cluster 2"=w147, "Value"=w107) -> ("Cluster"=→"R-Plot 1":cluster{"Time":dbl[], "T":dbl[]})
                n77 = call "Select Data Array.vi"("Cluster 2"=w146, "Value"=w107) -> ("Cluster"=→"R-Plot 2":cluster{"Time":dbl[], "T":dbl[]})
                n78 = call "Select Data Array.vi"("Cluster 2"=w145, "Value"=w107) -> ("Cluster"=→"R-Plot 3":cluster{"Time":dbl[], "T":dbl[]})
                n79 = call "Select Data Array.vi"("Cluster 2"=w144, "Value"=w107) -> ("Cluster"=→"R-Plot 4":cluster{"Time":dbl[], "T":dbl[]})
                n80 = call "Select Data Array.vi"("Cluster 2"=w143, "Value"=w107) -> ("Cluster"=→"R-Plot 5":cluster{"Time":dbl[], "T":dbl[]})
                n81 = call "Select Data Array.vi"("Cluster 2"=w142, "Value"=w107) -> ("Cluster"=→"R-Plot 6":cluster{"Time":dbl[], "T":dbl[]})
                n82 = call "Select Data Array.vi"("Cluster 2"=w141, "Value"=w107) -> ("Cluster"=→"R-Plot 7":cluster{"Time":dbl[], "T":dbl[]})
                n83 = call "Select Data Array.vi"("Cluster 2"=w140, "Value"=w107) -> ("Cluster"=→"R-Plot 8":cluster{"Time":dbl[], "T":dbl[]})
                n84 = call "Select Data Array.vi"("Cluster 2"=w139, "Value"=w107) -> ("Cluster"=→"R-Plot 9":cluster{"Time":dbl[], "T":dbl[]})
                n85 = Bundle("Cluster"=w129, "Cluster"=w130, "Cluster"=w131, "Cluster"=w132, "Cluster"=w138, "Cluster"=w133, "Cluster"=w134, "Cluster"=w135, "Cluster"=w136, "Cluster"=w137) -> (→"uPlots":T58)  [unwired: 1 in]
                n86 = local read "_ExtVIReference"() -> (w103:refnum<vi>)
                n87 = property on="CS Mode" class="Enum (strict)"() -> ("Value"=w152:T39)  [unwired: 2 in, 2 out]
                n88 = call "GetExtVIStatus.vi"("vi reference in"=w103) -> ("Exec.State"=→"CS.Mode1.VI State":T46)  [unwired: 2 out]
                n89 = Not(x="CS.Mode1.Auto Advance") -> (.not. x?=w151:bool)
                n90 = Equal To 0?(x=w152) -> (x = 0?=w101:bool)
                n91 = Generate User Event(user event=w88, event data cluster=bool[] [] ("event data")) -> ()  [unwired: 2 in, 2 out]
                n92 = Or(x=w101, y=w151) -> (x .or. y?=w150:bool)
                n93 = case shown="True" w150 {
                  frame False {
                  }
                  frame True {
                    n94 = call "Current Time(double).vi"() -> ("Current Time (double)"=w154:dbl)  [unwired: 6 in, 1 out]
                    n95 = local write "_TimeOld"(w154) -> ()
                  }
                }
                n96 = control-ref of="uA 2"() -> (w89:refnum<vi>)
                n97 = control-ref of="uA 3"() -> (w90:refnum<vi>)
                n98 = control-ref of="uA 0"() -> (w100:refnum<vi>)
                n99 = control-ref of="uA 1"() -> (w96:refnum<vi>)
                n100 = property class="DigNum (strict)"(reference=w100) -> (reference out=w99:refnum<vi>, "Key Focus"=w98:bool)  [unwired: 1 in, 1 out]
                n101 = property class="DigNum (strict)"(reference=w96) -> (reference out=w97:refnum<vi>, "Key Focus"=w95:bool)  [unwired: 1 in, 1 out]
                n102 = property class="DigNum (strict)"(reference=w89) -> (reference out=w91:refnum<vi>, "Key Focus"=w92:bool)  [unwired: 1 in, 1 out]
                n103 = property class="DigNum (strict)"(reference=w90) -> (reference out=w93:refnum<vi>, "Key Focus"=w94:bool)  [unwired: 1 in, 1 out]
                n104 = property class="DigNum (strict)"(reference=w99, "Visible"=w98) -> ()  [unwired: 1 in, 2 out]
                n105 = property class="DigNum (strict)"(reference=w97, "Visible"=w95) -> ()  [unwired: 1 in, 2 out]
                n106 = property class="DigNum (strict)"(reference=w91, "Visible"=w92) -> ()  [unwired: 1 in, 2 out]
                n107 = property class="DigNum (strict)"(reference=w93, "Visible"=w94) -> ()  [unwired: 1 in, 2 out]
              }
              frame #1 {
                n108 = property on="Bridge status" class="Clust (strict)"() -> ("Value"=w158:errorcluster)  [unwired: 2 in, 2 out]
                n109 = case shown="Error" w158 {
                  tunnel: w156 -> [_ w162]
                  tunnel: w155 -> [_ w161]
                  frame No Error {
                  }
                  frame Error {
                    n110 = call "StopScan.vi"("error in (no error)"=errorcluster {"status"=FALSE, "code"=0, "source"=""}, "path in"=w161) -> ("path out"=w168:path)  [unwired: 8 in, 1 out]
                    n111 = call "SetParFilePath.vi"("path"=w162, "zDll"=w168) -> ("error out"=w170:errorcluster, "zDll out"=w169:path)  [unwired: 8 in]
                    n112 = call "StartScan.vi"("error in (no error)"=w170, "path in"=w169) -> ("error out"=w166:errorcluster)  [unwired: 8 in, 1 out]
                    n113 = property on="Bridge status" class="Clust (strict)"("Value"=w166) -> ()  [unwired: 2 in, 2 out]
                    n114 = Unbundle By Name(w166) -> ("status"=w164:bool)
                    n115 = Not(x=w164) -> (.not. x?=w165:bool)
                    n116 = call "IsDisabled.vi"("Enabled?"=w165) -> ("Numeric"=w163:i16)
                    n117 = property on="Main Panel" class="TabCtl (strict)"("Disabled"=w163) -> ()  [unwired: 2 in, 2 out]
                    n118 = property on="Lower Panel" class="TabCtl (strict)"("Disabled"=w163) -> ()  [unwired: 2 in, 2 out]
                  }
                }
                n119 = property on="CS status" class="Clust (strict)"() -> ("Value"=w157:errorcluster)  [unwired: 2 in, 2 out]
                n120 = case shown="Error" w157 {
                  frame No Error {
                    n121 = property on="CS Indicators Panel" class="TabCtl (strict)"("Disabled"=u8 0) -> ()  [unwired: 2 in, 2 out]
                  }
                  frame Error {
                    n122 = property on="CS Indicators Panel" class="TabCtl (strict)"("Disabled"=u8 2) -> ()  [unwired: 2 in, 2 out]
                  }
                }
              }
              frame #2 {
                # "Check if the structure is \nnot empty and only one\nof Scalar or Array is set"
                # "Set FP control value from external script/program"
                n123 = local read "_SetControl"() -> (w171:T1)
                n124 = Unbundle By Name(w171) -> ("Name"=w173:string, "Scalar"=w172:string, "Array"=w181:string[][])
                n125 = call <userlib>:"Empty 2D Array (String)__ogtk.vi"("Array"=w181) -> ("Empty Array?"=w178:bool)  [unwired: 8 in]
                n126 = Empty String/Path?(string/path=w173) -> (empty?=w177:bool)
                n127 = Empty String/Path?(string/path=w172) -> (empty?=w176:bool)
                n128 = Not(x=w177) -> (.not. x?=w175:bool)
                n129 = Not(x=w176) -> (.not. x?=w179:bool)
                n130 = Not(x=w178) -> (.not. x?=w182:bool)
                n131 = Exclusive Or(1:w182, 2:w179) -> (0:w180:bool)
                n132 = And(x=w175, y=w180) -> (x .and. y?=w174:bool)
                n133 = case shown="True" w174 {
                  tunnel: w173 -> [_ w186]
                  tunnel: w172 -> [_ w185]
                  tunnel: w181 -> [_ w184]
                  tunnel: w182 -> [_ w183]
                  frame False {
                  }
                  frame True {
                    n134 = flat-sequence {
                      tunnel: w186 -> [w190]
                      tunnel: w185 -> [w189]
                      tunnel: w184 -> [w187]
                      tunnel: w183 -> [w188]
                      frame #0 {
                        n135 = local read "VIRef"() -> (w191:T2)
                        n136 = case shown="False" w188 {
                          tunnel: w191 -> [w194 w197]
                          tunnel: w190 -> [w193 w196]
                          tunnel: w189 -> [w192 _]
                          tunnel: w187 -> [_ w195]
                          frame False {
                            n137 = call "Push2VI.vi"("New Value"=w192, "element"=w193, "VIRef"=w194) -> ()  [unwired: 8 in, 1 out]
                          }
                          frame True {
                            n138 = call "PushArray2VI.vi"("Str"=w195, "element"=w196, "VIRef"=w197) -> ()  [unwired: 8 in, 1 out]
                          }
                        }
                      }
                      frame #1 {
                        w199 = ""
                        n139 = Bundle(w199, w199, "Array"=string[][] []) -> (→"_SetControl":cluster{string, string, "Array":string[][]})  [unwired: 1 in]
                      }
                    }
                  }
                }
              }
            }
          }
          frame True {
            # "First call  - do startup initialization"
            n140 = stacked-sequence {
              tunnel: w211 -> [_ _ w256 _]
              tunnel: [_ _ w250 _] -> w209
              tunnel: w210 -> [_ _ w252 _]
              tunnel: w208 -> [_ _ _ w311]
              tunnel: [_ _ w248 _] -> w205
              tunnel: [_ _ w249 _] -> w204
              tunnel: [_ _ w247 _] -> w203
              tunnel: [_ _ w245 _] -> w202
              tunnel: [w212 _ _ _] -> w201
              frame #0 {
                # "Set control bindings"
                # "\\\\localhost\\DR TempControl\\Currents(In)"
                # "\\\\localhost\\DR TempControl\\Temperatures"
                # "\\\\localhost\\DR TempControl\\Resistances"
                # "\\\\localhost\\DR TempControl\\Currents(Out)"
                n141 = disable-structure shown="RUN_TIME_ENGINE==True" {
                  disable-tunnel: [w225 "\\\\localhost\\DR TempControl\\"] -> w213
                  disable-tunnel: [w222 w235] -> w212
                  frame condition #0 {
                    w232 = u16 0 items=["overwrite", "ask first", "don't overwrite"] ("overwrite")
                    # "Deploy the shared variable library. If there are few copies of the program\nrunning - generate unique name for every copy."
                    n142 = call "Enum Variables.vi"("regular expression"="DR TempControl.*") -> ("Containers"=w230:string[])  [unwired: 15 in, 3 out]
                    n143 = call "Generate New Name.vi"("Existing names"=w230, "Base Name"="DR TempControl") -> ("New Name (path)"=w227:path, "New Name"=w226:string)  [unwired: 16 in]
                    n144 = call <userlib>:"Temporary Directory__ogtk.vi"("Relative path (.)"=w227) -> ("Temporary Directory (+ Relative)"=w231:path)
                    n145 = call <userlib>:"Current VIs Parent Directory__ogtk.vi"("Relative path (.)"=path "DR TempControl.lvlib" ("Library Path")) -> ("Parent Directory (+ Relative)"=w233:path)  [unwired: 4 in]
                    n146 = call <vilib>:"Librarian Copy.vi"("source"=w233, "overwrite"=w232, "destination"=w231) -> ("dup destination"=w222:path)  [unwired: 7 in, 1 out]
                    n147 = invoke class="App" method="Library.Deploy Library"("libPath"=w222) -> ()  [unwired: 4 in, 5 out]
                    n148 = Concatenate Strings("\\\\localhost\\" ("string"), w226, "\\" ("string")) -> (w225:string)
                  }
                  frame condition #1 (active) {
                    # "Default library is deployed automatically in development environment"
                    n149 = call <userlib>:"Current VIs Parent Directory__ogtk.vi"("Relative path (.)"=path "DR TempControl.lvlib" ("Library Path")) -> ("Parent Directory (+ Relative)"=w235:path)  [unwired: 4 in]
                  }
                }
                n150 = Concatenate Strings(w213, "Resistances" ("string")) -> (w219:string)
                n151 = Concatenate Strings(w213, "Temperatures" ("string")) -> (w216:string)
                n152 = Concatenate Strings(w213, "Currents(Out)" ("string")) -> (w215:string)
                n153 = Concatenate Strings(w213, "Currents(In)" ("string")) -> (w214:string)
                n154 = property on="R Array" class="Arr (strict)"("FPB.URL"=w219) -> ()  [unwired: 2 in, 2 out]
                n155 = property on="T Array" class="Arr (strict)"("FPB.URL"=w216) -> ()  [unwired: 2 in, 2 out]
                n156 = property on="CS.Actual Current" class="Arr (strict)"("FPB.URL"=w215) -> ()  [unwired: 2 in, 2 out]
                n157 = property on="CS.Automode Current" class="Arr (strict)"("FPB.URL"=w214) -> ()  [unwired: 2 in, 2 out]
              }
              frame #1 {
                w243 = u8 0 ("Disabled")
                n158 = call <userlib>:"Current VIs Reference__ogtk.vi"() -> ("Current VI's reference"=w241:refnum<vi>)  [unwired: 5 in]
                n159 = property on="Minimize UI 1" class="Bool (strict)"("Val(Sgnl)"=FALSE ("Value (Signaling)")) -> ()  [unwired: 2 in, 2 out]
                n160 = call "GetFrontPanelControls.vi"("Ref to VI"=w241) -> ("VIRef"=w240:T2)  [unwired: 9 in, 1 out]
                "VIRef" <- w240
                n161 = Unbundle By Name(w240) -> ("Full Name"=→"ControlNames":string[])
                n162 = property on="_String" class="Str"("Visible"=FALSE) -> ()  [unwired: 2 in, 2 out]
                n163 = property on="Lower Panel" class="TabCtl (strict)"("Disabled"=w243) -> ()  [unwired: 2 in, 2 out]
                n164 = property on="Main Panel" class="TabCtl (strict)"("Disabled"=w243) -> ()  [unwired: 2 in, 2 out]
                n165 = property on="CS Indicators Panel" class="TabCtl (strict)"("Disabled"=w243) -> ()  [unwired: 2 in, 2 out]
                n166 = property on="Side Panel" class="TabCtl (strict)"("Disabled"=w243) -> ()  [unwired: 2 in, 2 out]
                n167 = property on="Top Toolbar" class="TabCtl (strict)"("Disabled"=w243) -> ()  [unwired: 2 in, 2 out]
              }
              frame #2 {
                # "Read settings from the config file"
                n168 = flat-sequence {
                  tunnel: w256 -> [w257]
                  tunnel: [w257] -> w251
                  tunnel: [w260] -> w249
                  tunnel: [w261] -> w248
                  tunnel: [w262] -> w247
                  tunnel: [w261] -> w246
                  tunnel: [w258] -> w245
                  tunnel: [w277] -> w255
                  tunnel: w251 -> [w276]
                  tunnel: w246 -> [w278]
                  tunnel: w255 -> [w288]
                  tunnel: [w288] -> w254
                  tunnel: [w292] -> w253
                  tunnel: w254 -> [w289]
                  tunnel: w253 -> [w297]
                  tunnel: [w297] -> w244
                  tunnel: [w301] -> w250
                  tunnel: w252 -> [w298]
                  tunnel: w244 -> [w299]
                  frame #0 {
                    w263 = path "C:/LC Data" ("LC Data")
                    n169 = call "Generate config file path.vi"("LC data path"=w263) -> ("Config folder"=w262:path)  [unwired: 18 in]
                    n170 = call <userlib>:"Build Path - Traditional__ogtk.vi"("name or relative path"="config.ini", "base path"=w262) -> ("appended path"=w261:path)
                    n171 = call <userlib>:"Build Path - Traditional__ogtk.vi"("name or relative path"="Calibrations", "base path"=w263) -> ("appended path"=w260:path)
                    n172 = property on="Calibrations Folder" class="Path"("Value"=w260) -> ()  [unwired: 2 in, 2 out]
                    n173 = call <userlib>:"Current VIs Parent Directory__ogtk.vi"("Relative path (.)"=path "data/ImpBridgeDll.dll" ("Library Path")) -> ("Parent Directory (+ Relative)"=w258:path)  [unwired: 4 in]
                    "_zBridgeDll" <- w258
                  }
                  frame #1 {
                    n174 = control-ref of="zBridge.Active Channels"() -> (w275:refnum<vi>)
                    n175 = control-ref of="CS Settings"() -> (w274:refnum<vi>)
                    n176 = control-ref of="Bridge settings"() -> (w273:refnum<vi>)
                    n177 = control-ref of="Runtime Settings"() -> (w272:refnum<vi>)
                    n178 = control-ref of="Data Logging Settings"() -> (w271:refnum<vi>)
                    n179 = control-ref of="PID setup"() -> (w270:refnum<vi>)
                    n180 = control-ref of="CS Cannel Names"() -> (w284:refnum<vi>)
                    n181 = control-ref of="AVS names"() -> (w266:refnum<vi>)
                    n182 = control-ref of="_CurCalibrations"() -> (w267:refnum<vi>)
                    n183 = control-ref of="CS.Mode1.PID"() -> (w268:refnum<vi>)
                    n184 = control-ref of="CS.Mode1.Settings"() -> (w269:refnum<vi>)
                    n185 = call <userlib>:"Current VIs Parent Directory__ogtk.vi"("Relative path (.)"=path "data/config.ini") -> ("Parent Directory (+ Relative)"=w281:path)  [unwired: 4 in]
                    n186 = Build Array(w275, w274, w273, w272, w271, w270, w284, w266, w267, w268, w269) -> (w280:refnum<vi>[])
                    n187 = call "Save Load Settings to File by Ref with path.vi"("Array of Cluster References"=w280, "Action"=enum8{"Load", "Save"}."Load", "error in (no error)"=w276, "Configuration file"=w281) -> ("error out"=w283:errorcluster)  [unwired: 5 in]
                    n188 = call <userlib>:"MGI Clear Error.vi"("Error In"=w283) -> ("Error Out"=w282:errorcluster)  [unwired: 6 in]
                    n189 = call "Save Load Settings to File by Ref with path.vi"("Array of Cluster References"=w280, "Action"=enum8{"Load", "Save"}."Load", "error in (no error)"=w282, "Configuration file"=w278) -> ("error out"=w277:errorcluster)  [unwired: 5 in]
                  }
                  frame #2 {
                    n190 = Wait (ms)(milliseconds to wait=250) -> ()  [unwired: 1 out]
                  }
                  frame #3 {
                    n191 = control-ref of="Sensor Calibrations"() -> (w291:refnum<vi>)
                    n192 = control-ref of="_CurCalibrations"() -> (w290:refnum<vi>)
                    n193 = control-ref of="Calibrations Folder"() -> (w294:refnum<vi>)
                    n194 = control-ref of="_QuickConvertCal"() -> (w293:refnum<vi>)
                    n195 = control-ref of="Sensor 1"() -> (w295:refnum<vi>)
                    n196 = call "ReloadCalibrations.vi"("error in (no error)"=w289, "Quick convert sensors"=w293, "CurCalibrations"=w290, "Calibration files path"=w294, "Channel1 sensors"=w295, "Channels list"=w291) -> ("error out"=w292:errorcluster)  [unwired: 1 in]
                  }
                  frame #4 {
                    n197 = Wait (ms)(milliseconds to wait=250) -> ()  [unwired: 1 out]
                  }
                  frame #5 {
                    n198 = Generate User Event(user event=w298, event data cluster="" ("event data"), error in=w299) -> (error out=w301:errorcluster)  [unwired: 1 in, 1 out]
                  }
                }
              }
              frame #3 {
                w303 = FALSE ("Mode1 ON")
                w320 = u8 0 ("Disabled")
                # "Set enabled/disabled AVS channels"
                # "Reset pid parameters"
                # "Print VI version in the (upper right) corner"
                # "Reset Current lists\nto first element"
                # "Hardware settings"
                # "Reset currents lists"
                # "Set initial controls state"
                n199 = call "Currents-Temp list - check ranges.vi"() -> ("I_list out"=w314:dbl[][])  [unwired: 5 in]
                n200 = property on="Start" class="Bool (strict)"("Visible"=TRUE, "Disabled"=u8 0, "Value"=FALSE ("start")) -> ()  [unwired: 2 in, 2 out]
                n201 = property on="CS.Mode1.List:Index" class="DigNum (strict)"("Val(Sgnl)"=1 ("Value (Signaling)")) -> ()  [unwired: 2 in, 2 out]
                n202 = property on="CS Mode" class="Enum (strict)"("Val(Sgnl)"=CS_mode."Manual" ("CS Mode")) -> ()  [unwired: 2 in, 2 out]
                n203 = local write "CS.Mode2.List"(w314) -> ()
                n204 = property on="CS.Mode1.List:To First" class="Bool (strict)"("Val(Sgnl)"=TRUE ("Value (Signaling)")) -> ()  [unwired: 2 in, 2 out]
                n205 = property on="CS.Mode1.Start" class="Bool (strict)"("Value"=w303) -> ()  [unwired: 2 in, 2 out]
                n206 = property on="CS.Mode2.Start" class="Bool (strict)"("Value"=w303) -> ()  [unwired: 2 in, 2 out]
                n207 = property on="CS.QCS I0 Output" class="Enum (strict)"("Disabled"=u8 2, "Val(Sgnl)"=T38."Channel 0" ("Map Channel 0 to")) -> ()  [unwired: 2 in, 2 out]
                n208 = property on="Bridge Type" class="Enum (strict)"("Disabled"=w320) -> ()  [unwired: 2 in, 2 out]
                n209 = property on="AVS GPIB Address" class="VISAName"("Disabled"=w320) -> ()  [unwired: 2 in, 2 out]
                n210 = property on="TCS RS232 Port" class="VISAName"("Disabled"=w320) -> ()  [unwired: 2 in, 2 out]
                n211 = property on="CS type" class="Enum (strict)"("Disabled"=w320) -> ()  [unwired: 2 in, 2 out]
                n212 = property on="CS.QCS Device Nr" class="DigNum (strict)"("Disabled"=w320) -> ()  [unwired: 2 in, 2 out]
                n213 = property on="Side Panel" class="TabCtl (strict)"("Value"=T34."Devices Settings" ("Tab Control 2")) -> ("Pages"=w308:refnum<vi>[])  [unwired: 2 in, 2 out]
                n214 = Index Array(array=w308, index=1) -> (element=w305:refnum<vi>)
                n215 = property class="App"() -> ("App.Kind"=w317:T59)  [unwired: 2 in, 2 out]
                n216 = property class="Page"(reference=w305, "PageEnb"=T51."Page Disabled & Grayed" ("Page Enabled State")) -> ()  [unwired: 1 in, 2 out]
                n217 = case shown="\"Run Time System\"" w317 {
                  tunnel: [w325 w333] -> w302
                  frame "invalid app kind", Default {
                    n218 = control-ref of="This VI"() -> (w332:refnum<vi>)
                    n219 = property class="VI"(reference=w332) -> ("Hist.Revision"=w331:u32)  [unwired: 1 in, 2 out]
                    n220 = Divide(x=w331, y=1000.0 ("x")) -> (x/y=w327:dbl)
                    n221 = Number To Fractional String(use system decimal point (T)=FALSE, number=w327, precision (6)=i16 2) -> (F-format string=w326:string)  [unwired: 1 in]
                    n222 = Concatenate Strings("" ("string"), w326) -> (w325:string)
                  }
                  frame "Run Time System" {
                    n223 = call <userlib>:"MGI Get Executable Version.vi"() -> ("Version"=w333:string)  [unwired: 7 in]
                  }
                }
                "VI Version" <- w302
                n224 = property on="Channels Panel" class="TabCtl (strict)"("Val(Sgnl)"=T8."All" ("Value (Signaling)")) -> ()  [unwired: 2 in, 2 out]
                n225 = local write "CS.Mode1.PID Error"(0.0 ("T_error")) -> ()
                n226 = Generate User Event(user event=w311, event data cluster=bool[] [] ("event data")) -> ()  [unwired: 2 in, 2 out]
              }
            }
            n227 = Bundle By Name(cluster=w207, "Config folder"=w203, "Config File"=w205, "Calibrations Folder"=w204, "zBridge dll"=w202, "Variables Library"=w201) -> (w206:T50)
          }
        }
      }
      event "Start": Value Change {
        # "\"Start\" button clicked -> start measuring"
        n228 = event-data() -> ()  [unwired: 1 in, 6 out]
        n229 = Unbundle By Name(w337) -> ("Config File"=w334:path, "zBridge dll"=w335:path, "Config folder"=w336:path)
        n230 = stacked-sequence {
          tunnel: w338 -> [_ _ _ _ _ _ w465]
          tunnel: w336 -> [_ _ _ _ w407 _ _]
          tunnel: w335 -> [_ _ _ _ w406 _ _]
          tunnel: w334 -> [_ w348 _ _ _ _ _]
          frame #0 {
            n231 = property on="Run Description" class="Str"() -> ("Value"=w341:string)  [unwired: 2 in, 2 out]
            n232 = property on="Query Description" class="Bool (strict)"() -> ("Value"=w340:bool)  [unwired: 2 in, 2 out]
            n233 = Not(x=w340) -> (.not. x?=w339:bool)
            n234 = call "Run Reference DLG.vi"("Enable"=w340, "Run Reference"=w341, "Dont' ask again"=w339) -> ("Dont' ask again"=w343:bool, "Run Reference"=w344:string, "OK"=w345:bool)  [unwired: 13 in, 1 out]
            n235 = Not(x=w343) -> (.not. x?=w342:bool)
            n236 = case shown="True" w345 {
              tunnel: w344 -> [_ w347]
              tunnel: w342 -> [_ w346]
              frame False {
              }
              frame True {
                n237 = property on="Run Description" class="Str"("Val(Sgnl)"=w347) -> ()  [unwired: 2 in, 2 out]
                n238 = property on="Query Description" class="Bool (strict)"("Val(Sgnl)"=w346) -> ()  [unwired: 2 in, 2 out]
              }
            }
          }
          frame #1 {
            # "Save new settings to config file"
            n239 = control-ref of="zBridge.Active Channels"() -> (w352:refnum<vi>)
            n240 = control-ref of="CS.Mode1.PID"() -> (w351:refnum<vi>)
            n241 = control-ref of="CS.Mode1.Settings"() -> (w350:refnum<vi>)
            n242 = control-ref of="CS.Mode1.Settings"() -> (w349:refnum<vi>)
            n243 = control-ref of="CS Cannel Names"() -> (w355:refnum<vi>)
            n244 = control-ref of="AVS names"() -> (w354:refnum<vi>)
            n245 = control-ref of="_CurCalibrations"() -> (w353:refnum<vi>)
            n246 = control-ref of="Bridge settings"() -> (w360:refnum<vi>)
            n247 = control-ref of="Runtime Settings"() -> (w361:refnum<vi>)
            n248 = control-ref of="CS Settings"() -> (w359:refnum<vi>)
            n249 = control-ref of="Sensor Calibrations"() -> (w362:refnum<vi>)
            n250 = control-ref of="PID setup"() -> (w363:refnum<vi>)
            n251 = control-ref of="Data Logging Settings"() -> (w358:refnum<vi>)
            n252 = Build Array(w352, w360, w361, w359, w358, w362, w363, w355, w354, w353, w351, w350, w349) -> (w356:refnum<vi>[])
            n253 = call "Save Load Settings to File by Ref with path.vi"("Array of Cluster References"=w356, "Action"=enum8{"Load", "Save"}."Save", "Configuration file"=w348) -> ()  [unwired: 6 in, 1 out]
          }
          frame #2 {
            w379 = u8 2 ("Disabled")
            # "Reset stop button"
            # "Hide Disable Start button"
            # "Load external calibration VI"
            # "Set controls\nInitialize data for run"
            # "Lock hardware settings"
            n254 = property on="Bridge Type" class="Enum (strict)"("Disabled"=w379) -> ()  [unwired: 2 in, 2 out]
            n255 = property on="AVS GPIB Address" class="VISAName"("Disabled"=w379) -> ()  [unwired: 2 in, 2 out]
            n256 = property on="AVS RS232 Port" class="VISAName"("Disabled"=w379) -> ()  [unwired: 2 in, 2 out]
            n257 = property on="TCS RS232 Port" class="VISAName"("Disabled"=w379) -> ()  [unwired: 2 in, 2 out]
            n258 = property on="CS type" class="Enum (strict)"("Disabled"=w379) -> ()  [unwired: 2 in, 2 out]
            n259 = property on="CS.QCS Device Nr" class="DigNum (strict)"("Disabled"=w379) -> ()  [unwired: 2 in, 2 out]
            n260 = property on="CS.QCS I0 Output" class="Enum (strict)"("Disabled"=u8 0) -> ()  [unwired: 2 in, 2 out]
            n261 = call "Current Time(double).vi"() -> ("Current Time (double)"=w368:dbl)  [unwired: 6 in, 1 out]
            n262 = local write "_TimeOld"(w368) -> ()
            n263 = property on="External VI Path" class="Path"() -> ("Value"=w378:path)  [unwired: 2 in, 2 out]
            n264 = vi-ref "OnTempStabilizedRef.vi"() -> (w377:refnum<vi>)
            n265 = local write "VI called?"(FALSE ("VI called?")) -> ()
            n266 = Open VI Reference(type specifier VI Refnum (for type only)=w377, vi path=w378) -> (vi reference=→"_ExtVIReference":refnum<vi>)  [unwired: 4 in, 1 out]
            n267 = property on="Start" class="Bool (strict)"("Visible"=TRUE, "Disabled"=u8 2) -> ()  [unwired: 2 in, 2 out]
            n268 = Initialize Array(cluster{"R":dbl[], "T":dbl[], "Time":dbl[]} {"R"=[], "T"=[], "Time"=[]}, 10 ("dimension size")) -> (w372:cluster{"R":dbl[], "T":dbl[], "Time":dbl[]}[])
            n269 = local write "Data Array"(w372) -> ()
            n270 = disable-structure shown="Enabled" {
              frame Enabled {
                n271 = property on="Stop" class="Bool (strict)"("Value"=FALSE ("MainStopButton")) -> ()  [unwired: 2 in, 2 out]
              }
              frame Disabled {
              }
            }
            n272 = property on="Side Panel" class="TabCtl (strict)"() -> ("Pages"=w367:refnum<vi>[])  [unwired: 2 in, 2 out]
            n273 = Index Array(array=w367, index=1) -> (element=w365:refnum<vi>)
            n274 = property class="Page"(reference=w365, "PageEnb"=T51."Page Enabled" ("Page Enabled State")) -> ()  [unwired: 1 in, 2 out]
          }
          frame #3 {
            # "Initialize CS"
            n275 = local read "_CSClassRef"() -> (w391:refnum<class "CS.lvclass">)
            n276 = call-dynamic "Initialize.vi"("CS in"=w391, "HW Address"="_CS_Address", "error in (no error)"=T52 {"error"=FALSE, "code"=0, "source"=""} ("error in")) -> ("CS out"=w384:refnum<class "CS.lvclass">, "Instrument ID"=→"CS.ID":string, "error out"=w383:errorcluster)  [unwired: 10 in]
            n277 = call-dynamic "Get Currents & Ranges.vi"("CS.lvclass in"=w384, "error in (no error)"=w383) -> ("CS.lvclass out"=w392:refnum<class "CS.lvclass">, "I0"=w393:cluster{"Value":dbl, "Range":dbl}, "I1"=w385:cluster{"Value":dbl, "Range":dbl}, "I2"=w386:cluster{"Value":dbl, "Range":dbl}, "I3"=w387:cluster{"Value":dbl, "Range":dbl}, "error out"=w389:errorcluster)  [unwired: 12 in]
            "CS status" <- w389
            n278 = local write "_CSClassRef"(w392) -> ()
            n279 = Unbundle By Name(w389) -> ("status"=w381:bool)
            n280 = case shown="False" w381 {
              tunnel: w385 -> [w405 _]
              tunnel: w386 -> [w404 _]
              tunnel: w387 -> [w403 _]
              tunnel: w393 -> [w397 _]
              frame False {
                n281 = Unbundle By Name(w397) -> ("Value"=w396:dbl, "Range"=w395:dbl)
                n282 = Unbundle By Name(w405) -> ("Value"=w402:dbl, "Range"=w401:dbl)
                n283 = Unbundle By Name(w404) -> ("Value"=w400:dbl, "Range"=w399:dbl)
                n284 = Unbundle By Name(w403) -> ("Value"=w394:dbl, "Range"=w398:dbl)
                n285 = property on="I" class="DigNum (strict)"("Value"=w396) -> ()  [unwired: 2 in, 2 out]
                n286 = property on="I" class="DigNum (strict)"("Value"=w402) -> ()  [unwired: 2 in, 2 out]
                n287 = property on="I" class="DigNum (strict)"("Value"=w400) -> ()  [unwired: 2 in, 2 out]
                n288 = property on="I" class="DigNum (strict)"("Value"=w394) -> ()  [unwired: 2 in, 2 out]
                n289 = property on="Range" class="Enum (strict)"("Value"=w395) -> ()  [unwired: 2 in, 2 out]
                n290 = property on="Range" class="Enum (strict)"("Value"=w401) -> ()  [unwired: 2 in, 2 out]
                n291 = property on="Range" class="Enum (strict)"("Value"=w399) -> ()  [unwired: 2 in, 2 out]
                n292 = property on="Range" class="Enum (strict)"("Value"=w398) -> ()  [unwired: 2 in, 2 out]
              }
              frame True {
              }
            }
          }
          frame #4 {
            # "Initialize AVS/zBridge"
            n293 = property on="Bridge Type" class="Enum (strict)"() -> ("Value"=w412:T60)  [unwired: 2 in, 2 out]
            n294 = case shown="\"AVS47A (GPIB interface)\"" w412 {
              tunnel: [w418 w427 w443 refnum<visa-resource-name> refnum ("dup VISA session") refnum<visa-resource-name> refnum ("dup VISA session")] -> w411
              tunnel: [w417 w430 _ w451 errorcluster {"status"=FALSE, "code"=0, "source"=""} ("error out")] -> w410
              tunnel: [_ _ w442 _ _] -> _
              tunnel: w407 -> [_ _ _ w448 _]
              tunnel: w406 -> [_ _ _ w447 _]
              frame "AVS47A (GPIB interface)" {
                # "Set default Parameters,\n enable Autoranging"
                n295 = property on="AVS GPIB Address" class="VISAName"() -> ("Value"=w413:refnum<visa-resource-name>)  [unwired: 2 in, 2 out]
                n296 = call "AVS47IB Initialize.vi"("Instr. Descriptor (GPIB::)"=w413) -> ("VISA session"=w426:refnum<visa-resource-name>, "error out"=w414:errorcluster)  [unwired: 13 in]
                n297 = call "AVS47IB Stop.vi"("VISA session"=w426, "error in (no error)"=w414) -> ("dup VISA session"=w424:refnum<visa-resource-name>, "error out"=w416:errorcluster)  [unwired: 12 in]
                n298 = call "AVS47IB Go Remote.vi"("VISA session"=w424, "error in (no error)"=w416) -> ("dup VISA session"=w425:refnum<visa-resource-name>, "error out"=w415:errorcluster)  [unwired: 12 in]
                n299 = call "AVS47IB Configure 47IB.vi"("VISA session"=w425, "Printer Enabled (-1:no change)"=i8 0, "Buffer Enabled (-1:no change)"=i8 0, "Message Headers Included  (-1:no change)"=i8 0, "Autoranging Enabled (-1:no change)"=i8 1, "Stabilisation Delay (-1:no change)"=i8 15, "error in (no error)"=w415) -> ("dup VISA session"=w418:refnum<visa-resource-name>, "error out"=w417:errorcluster)  [unwired: 7 in]
              }
              frame "AVS47B (RS232 interface)" {
                n300 = property on="Bridge settings" class="Clust (strict)"() -> ("Value"=w434:T35)  [unwired: 2 in, 2 out]
                n301 = Unbundle By Name(w434) -> ("AVS RS232 Port"=w433:refnum<visa-resource-name>)
                n302 = call "InitPort_b.vi"("VISA resource"=w433) -> ("error out"=w429:errorcluster, "dup VISA resource"=w432:refnum<visa-resource-name>)  [unwired: 5 in]
                n303 = Type Cast(type=refnum<visa-resource-name> refnum ("dup VISA session"), x=w432) -> (*(type *) &x=w428:refnum<visa-resource-name>)
                n304 = case shown="Error" w429 {
                  selector: w429 -> [w435 w438]
                  tunnel: w428 -> [w436 w440]
                  tunnel: [w435 w439] -> w430
                  tunnel: [w436 refnum<visa-resource-name> refnum ("dup VISA session")] -> w427
                  frame No Error {
                  }
                  frame Error {
                    n305 = VISA Close(VISA resource name=w440, error in (no error)=w438) -> (error out=w439:errorcluster)
                  }
                }
              }
              frame "AVS48SI (RS232 interface)" {
                n306 = property on="Bridge settings" class="Clust (strict)"() -> ("Value"=w446:T35)  [unwired: 2 in, 2 out]
                n307 = Unbundle By Name(w446) -> ("AVS RS232 Port"=w444:refnum<visa-resource-name>)
                n308 = call "Configure Hardware.vi"("VISA RESOURCE NAME"=w444) -> ("THREAD OUT"=w441:string)  [unwired: 14 in]
                n309 = call "Configure Sensor Wiring of CHs.vi"("THREAD IN"=w441) -> ("THREAD OUT"=w442:string)  [unwired: 10 in]
                n310 = Type Cast(type=refnum<visa-resource-name> refnum ("dup VISA session"), x=w444) -> (*(type *) &x=w443:refnum<visa-resource-name>)
              }
              frame "Impedance Bridge" {
                n311 = call "SetParFilePath.vi"("path"=w448, "zDll"=w447) -> ("error out"=w450:errorcluster, "zDll out"=w449:path)  [unwired: 8 in]
                n312 = call "StartScan.vi"("error in (no error)"=w450, "path in"=w449) -> ("error out"=w451:errorcluster)  [unwired: 8 in, 1 out]
              }
              frame "Disabled", Default {
              }
            }
            "_AVS_VISA" <- w411
            n313 = property on="Bridge status" class="Clust (strict)"("Value"=w410) -> ()  [unwired: 2 in, 2 out]
            n314 = property on="_ScanData" class="Arr (strict)"("Value"=dbl[] [0.0, 0.0, 0.0, 0.0, 0.0, 0.0, 0.0, 0.0, 0.0, 0.0] ("R_array")) -> ()  [unwired: 2 in, 2 out]
            n315 = call "ScanParameters FGV.vi"("Action"=Action."Init") -> ()  [unwired: 10 in, 1 out]
          }
          frame #5 {
            # "Generate paths for log files"
            n316 = Unbundle By Name("Data Logging Settings") -> ("Run Description"=w458:string, "Filenames Suffix"=w459:string, "Log Files Folder"=w456:path, "Log Files Name"=w462:string, "Automode Files Name"=w461:string)
            n317 = call <userlib>:"Create Dir if Non-Existant__ogtk.vi"("Directory Path"=w456) -> ("dup Directory Path"=w455:path)  [unwired: 8 in, 2 out]
            n318 = call <userlib>:"MGI Make String Filesafe.vi"("String In"=w458) -> ("Filesafe String Out"=w457:string)
            n319 = call "GeneratePaths.vi"("Filename Suffix"=w459, "Run description"=w457, "AVS_Path"=w455, "AVS_FName"=w462, "CAL_Path"=w455, "CAL_FName"=w461) -> ("Generated Log path"=w460:path, "Generated Calib path"=→"_CalibFilesPath":path)  [unwired: 8 in]
            n320 = property on="_LogFilesPath" class="Path"("Val(Sgnl)"=w460) -> ()  [unwired: 2 in, 2 out]
          }
          frame #6 {
            # "Start measurements"
            n321 = Set Occurrence(w465) -> ()
          }
        }
      }
      event "Stop": Value Change; Application Instance Close {
        # "\"Stop\" button pressed -> Stop measuring."
        n322 = event-data() -> ()  [unwired: 1 in, 1 out]
        n323 = flat-sequence {
          tunnel: w467 -> [w470]
          tunnel: w468 -> [w485]
          tunnel: w466 -> [w499]
          frame #0 {
            # "Save settings to config file"
            n324 = control-ref of="zBridge.Active Channels"() -> (w473:refnum<vi>)
            n325 = control-ref of="Bridge settings"() -> (w480:refnum<vi>)
            n326 = control-ref of="Runtime Settings"() -> (w479:refnum<vi>)
            n327 = control-ref of="CS Settings"() -> (w481:refnum<vi>)
            n328 = control-ref of="Data Logging Settings"() -> (w482:refnum<vi>)
            n329 = control-ref of="Sensor Calibrations"() -> (w478:refnum<vi>)
            n330 = control-ref of="PID Settings"() -> (w477:refnum<vi>)
            n331 = control-ref of="CS Cannel Names"() -> (w476:refnum<vi>)
            n332 = control-ref of="Channel names"() -> (w475:refnum<vi>)
            n333 = control-ref of="Curent Calibrations"() -> (w474:refnum<vi>)
            n334 = control-ref of="CS.Mode1.PID"() -> (w472:refnum<vi>)
            n335 = control-ref of="CS.Mode1.Settings"() -> (w471:refnum<vi>)
            n336 = Build Array(w473, w480, w479, w481, w482, w478, w477, w476, w475, w474, w472, w471) -> (w484:refnum<vi>[])
            n337 = call "Save Load Settings to File by Ref with path.vi"("Array of Cluster References"=w484, "Action"=enum8{"Load", "Save"}."Save", "Configuration file"=w470) -> ()  [unwired: 6 in, 1 out]
          }
          frame #1 {
            # "Free serial ports"
            n338 = control-ref of="_AVS_VISA"() -> (w486:refnum<vi>)
            n339 = control-ref of="TCS RS232 Port"() -> (w491:refnum<vi>)
            n340 = call "StopScan.vi"("path in"=w485) -> ()  [unwired: 9 in, 2 out]
            n341 = property class="VISAName"(reference=w486) -> (error out=w488:errorcluster, "Value"=w487:refnum<visa-resource-name>)  [unwired: 1 in, 1 out]
            n342 = property class="VISAName"(reference=w491) -> (error out=w489:errorcluster, "Value"=w490:refnum<visa-resource-name>)  [unwired: 1 in, 1 out]
            n343 = VISA Close(VISA resource name=w487, error in (no error)=w488) -> ()  [unwired: 1 out]
            n344 = VISA Close(VISA resource name=w490, error in (no error)=w489) -> ()  [unwired: 1 out]
          }
          frame #2 {
            w493 = u8 0 ("Disabled")
            # "Reset controls state"
            n345 = property on="Bridge Type" class="Enum (strict)"("Disabled"=w493) -> ()  [unwired: 2 in, 2 out]
            n346 = property on="AVS GPIB Address" class="VISAName"("Disabled"=w493) -> ()  [unwired: 2 in, 2 out]
            n347 = property on="AVS RS232 Port" class="VISAName"("Disabled"=w493) -> ()  [unwired: 2 in, 2 out]
            n348 = property on="TCS RS232 Port" class="VISAName"("Disabled"=w493) -> ()  [unwired: 2 in, 2 out]
            n349 = property on="CS type" class="Enum (strict)"("Disabled"=w493) -> ()  [unwired: 2 in, 2 out]
            n350 = property on="CS.QCS Device Nr" class="DigNum (strict)"("Disabled"=w493) -> ()  [unwired: 2 in, 2 out]
            n351 = property on="Start" class="Bool (strict)"("Visible"=TRUE, "Disabled"=u8 0, "Value"=FALSE ("start")) -> ()  [unwired: 2 in, 2 out]
            n352 = property on="Stop" class="Bool (strict)"("Value"=FALSE ("MainStopButton")) -> ()  [unwired: 2 in, 2 out]
          }
          frame #3 {
            w497 = u8 2 ("Disabled")
            # "Disable UI"
            n353 = property on="Top Toolbar" class="TabCtl (strict)"("Disabled"=w497) -> ()  [unwired: 2 in, 2 out]
            n354 = property on="Main Panel" class="TabCtl (strict)"("Disabled"=w497) -> ()  [unwired: 2 in, 2 out]
            n355 = property on="CS Indicators Panel" class="TabCtl (strict)"("Disabled"=w497) -> ()  [unwired: 2 in, 2 out]
            n356 = property on="Side Panel" class="TabCtl (strict)"("Disabled"=w497) -> ()  [unwired: 2 in, 2 out]
            n357 = property on="Lower Panel" class="TabCtl (strict)"("Disabled"=w497) -> ()  [unwired: 2 in, 2 out]
            n358 = property on="_String" class="Str"("Visible"=TRUE) -> ()  [unwired: 2 in, 2 out]
          }
          frame #4 {
            n359 = invoke class="App" method="Library.UndeployLibrary"("libPath"=w499) -> ()  [unwired: 4 in, 5 out]
          }
          frame #5 {
            # "Stop \nexecution"
            n360 = Stop(stop? (T)=TRUE) -> ()
          }
        }
        n361 = Unbundle By Name(w469) -> ("Variables Library"=w466:path, "zBridge dll"=w468:path, "Config File"=w467:path)
      }
      event "_ScanData": Value Change {
        # "Convert 8 elements AVS\narray to 10 elements"
        # "Received new data from AVS/zBridge. Do general tasks - update indicators, calculate temperature and pass the data further to AVS/zBridge specific processing"
        n362 = event-data() -> ("NewVal"=w517:dbl[])  [unwired: 1 in]
        n363 = Unbundle By Name(w505) -> ("UpdateValuesAVS"=w503:refnum<user-event>, "UpdateValuesZBridge"=w504:refnum<user-event>)
        n364 = Unbundle By Name(w501) -> ("Calibrations Folder"=w502:path)
        n365 = for {
          tunnel: w517 -> [w546] mode=indexing
          tunnel: [w544] -> w513 mode=indexing
          n366 = Less?(x=w546, y=1e+25) -> (x < y?=w547:bool)
          n367 = Select(t=w546, s=w547, f=inf) -> (s? t:f=w544:dbl)
        }
        n368 = Index Array(array=w513) -> (element #1=→"R0":dbl, element #2=→"R1":dbl, element #3=→"R2":dbl, element #4=→"R3":dbl, element #5=→"R4":dbl, element #6=→"R5":dbl, element #7=→"R6":dbl, element #8=→"R7":dbl, element #9=→"R8":dbl, element #10=→"R9":dbl)  [unwired: 10 in]
        n369 = Array To Cluster(array=w513) -> (cluster=w507:T61)
        "R Cluster" <- w507
        n370 = Cluster To Array(cluster=w507) -> (array=w506:dbl[])
        n371 = Absolute Value(x=w506) -> (abs(x)=w514:dbl[])
        n372 = property on="Allow neg R" class="Bool (strict)"() -> ("Value"=w512:bool)  [unwired: 2 in, 2 out]
        n373 = Select(t=w506, s=w512, f=w514) -> (s? t:f=w511:dbl[])
        "R Array" <- w511
        n374 = local read "_CurCalibrations"() -> (w519:T33)
        n375 = Cluster To Array(cluster=w519) -> (array=w518:string[])
        n376 = call "Resistance to Temp no Ext.vi"("error in"=w520, "Path"=w502, "CurCalibrations"=w518, "Resistance"=w511) -> ("Temperature"=w509:dbl[])  [unwired: 1 in, 3 out]
        "T Array" <- w509
        n377 = Array To Cluster(array=w509) -> (cluster=w525:T62)
        "T Cluster" <- w525
        n378 = Unbundle(w525) -> ("Temperature[0]"=→"T0":dbl, "Temperature[1]"=→"T1":dbl, "Temperature[2]"=→"T2":dbl, "Temperature[3]"=→"T3":dbl, "Temperature[4]"=→"T4":dbl, "Temperature[5]"=→"T5":dbl, "Temperature[6]"=→"T6":dbl, "Temperature[7]"=→"T7":dbl, "Temperature[8]"=→"T8":dbl, "Temperature[9]"=→"T9":dbl)
        n379 = property on="Mode Buttons" class="RadioBtnsControl (strict)"() -> ("Value"=w524:T7)  [unwired: 2 in, 2 out]
        n380 = Array To Cluster(array=w511) -> (cluster=w510:T61)
        n381 = Array To Cluster(array=w509) -> (cluster=w508:T62)
        n382 = case shown="\"No Selection\", Default" w524 {
          tunnel: w508 -> [w559 _]
          tunnel: w510 -> [w560 _]
          frame "No Selection", Default {
            n383 = call "Current Time(double).vi"() -> ("Current Time (double)"=→"Time":dbl)  [unwired: 6 in, 1 out]
            "Small R Cluster" <- w560
            "Small T Cluster" <- w559
          }
          frame "Cursor mode" {
          }
        }
        n384 = Bundle(w511, "Temperature"=w509) -> (w522:cluster{dbl[], "Temperature":dbl[]})  [unwired: 1 in]
        n385 = property on="Bridge Type" class="Enum (strict)"() -> ("Value"=w521:T60)  [unwired: 2 in, 2 out]
        n386 = case shown="\"AVS47B (RS232 interface)\", Default" w521 {
          tunnel: [w552 w553 w556] -> w523
          tunnel: w520 -> [w551 w553 w557]
          tunnel: w522 -> [w550 _ w555]
          tunnel: w504 -> [_ _ w554]
          tunnel: w503 -> [w549 _ _]
          frame "AVS47B (RS232 interface)", Default {
            n387 = Generate User Event(user event=w549, event data cluster=w550, error in=w551) -> (error out=w552:errorcluster)  [unwired: 1 in, 1 out]
          }
          frame "Disabled" {
          }
          frame "Impedance Bridge" {
            n388 = Generate User Event(user event=w554, event data cluster=w555, error in=w557) -> (error out=w556:errorcluster)  [unwired: 1 in, 1 out]
          }
        }
      }
      event User Event {
        # "Process data from the AVS bridge"
        n389 = event-data() -> ("R"=w565:dbl[], "T"=w564:dbl[])  [unwired: 1 in]
        n390 = property on="CS.Actual Current" class="Arr (strict)"() -> ("Value"=w566:dbl[])  [unwired: 2 in, 2 out]
        n391 = Unbundle By Name(w563) -> ("CS Automode"=w562:refnum<user-event>)
        n392 = stacked-sequence {
          tunnel: w568 -> [_ w586 _]
          tunnel: [_ w610 _] -> w567
          tunnel: w566 -> [_ w587 w641]
          tunnel: w565 -> [w576 w589 w643]
          tunnel: w564 -> [w575 w588 w642]
          tunnel: w562 -> [w573 _ _]
          frame #0 {
            # "Filter data and add it to the data array. \nDo PID"
            n393 = property on="Runtime Settings" class="Clust (strict)"() -> ("Value"=w579:T27)  [unwired: 2 in, 2 out]
            n394 = Unbundle By Name(w579) -> ("Y_max"=w582:dbl, "Y_min"=w581:dbl, "Filter Graphs"=w580:bool)
            n395 = local read "Data Array"() -> (w577:T28)
            n396 = property on="Data Memory" class="DigNum (strict)"() -> ("Value"=w584:u16)  [unwired: 2 in, 2 out]
            n397 = call "Current Time(double).vi"() -> ("Current Time (double)"=w574:dbl)  [unwired: 6 in, 1 out]
            n398 = call "Manage Data Arrays - AVS.vi"("Y_max"=w582, "Y_min"=w581, "Filter Graph Results"=w580, "Append New Data"=TRUE, "Data In"=w577, "Curr R"=w576, "Curr T"=w575, "Curr Time"=w574, "Data Memory"=w584) -> ("Data Out"=w578:T28)  [unwired: 10 in]
            n399 = Bundle("Current Time (double)"=w574, "R"=w576, "T"=w575) -> (w585:T63)  [unwired: 1 in]
            n400 = local write "Data Array"(w578) -> ()
            n401 = Generate User Event(user event=w573, event data cluster=w585) -> ()  [unwired: 2 in, 2 out]
            n402 = Initialize Array("Ohm" ("AVS Name 0"), 10 ("dimension size")) -> (w572:string[])
            n403 = Array To Cluster(array=w572) -> (cluster=w569:T33)
            n404 = local write "Units"(w569) -> ()
          }
          frame #1 {
            # "Save data to log file"
            n405 = local read "_LogFilesPath"() -> (w608:path)
            n406 = local read "_CalibFilesPath"() -> (w609:path)
            n407 = call <vilib>:"Check if File or Folder Exists.vi"("path"=w608) -> ("file or folder exists?"=w600:bool, "dup path"=w601:path)  [unwired: 8 in, 1 out]
            n408 = case shown="True" w600 {
              tunnel: w601 -> [w633 w640]
              tunnel: [w633 w640] -> w602
              tunnel: [w631 _] -> w594
              frame False {
                n409 = control-ref of="Sensor Calibrations"() -> (w636:refnum<vi>)
                n410 = property on="Run Description" class="Str"() -> ("Value"=w632:string)  [unwired: 2 in, 2 out]
                n411 = Cluster To Array(cluster="Sensor Names") -> (array=w638:string[])
                n412 = Cluster To Array(cluster="CS Cannel Names") -> (array=w639:string[])
                n413 = call "Format log file header Z.vi"("Thermometer"=w636, "AVS names"=w638, "CS Names"=w639, "Run description"=w632) -> ("String"=w634:string)  [unwired: 1 in]
                n414 = Write to Text File(file (use dialog)=w633, text=w634) -> (error out=w631:errorcluster)  [unwired: 2 in, 2 out]
              }
              frame True {
              }
            }
            n415 = property on="Data Logging Settings" class="Clust (strict)"() -> ("Value"=w619:T37)  [unwired: 2 in, 2 out]
            n416 = Unbundle By Name(w619) -> ("Delimeter"=w592:string, "Date Format"=w618:string)
            n417 = call "Current Time(double).vi"() -> ("Current Time"=w595:timestamp, "Current Time (double)"=w596:dbl)  [unwired: 6 in]
            n418 = call <userlib>:"File Info__ogtk.vi"("error in (no error)"=w594, "file"=w602) -> ("error out"=w593:errorcluster, "file info"=w598:T64, "file out"=w607:path)  [unwired: 4 in]
            n419 = Unbundle By Name(w598) -> ("creation date"=w599:u32)
            n420 = Number To Exponential String(number=w596, precision (6)=i16 10) -> (E-format string=w590:string)  [unwired: 2 in]
            n421 = Format Date/Time String(time format string (%c)=w618, seconds (now)=w595) -> (date/time string=w615:string)  [unwired: 1 in]
            n422 = Number To Fractional String(number=w589) -> (F-format string=w617:string[])  [unwired: 3 in]
            n423 = Number To Fractional String(number=w588) -> (F-format string=w616:string[])  [unwired: 3 in]
            n424 = Number To Fractional String(number=w587) -> (F-format string=w614:string[])  [unwired: 3 in]
            n425 = property on="New File Interval" class="DigNum (strict)"() -> ("Value"=w603:u32)  [unwired: 2 in, 2 out]
            n426 = property on="New File Interval Units" class="Enum (strict)"() -> ("Value"=w604:enum16{"Minutes", "Hours", "Days"})  [unwired: 2 in, 2 out]
            n427 = To Time Stamp(1:w599) -> (0:w605:timestamp)
            n428 = Build Array (concatenate)(w615, w590, w617, w616, w614) -> (w591:string[])
            n429 = call "Time Elapsed time.vi"("Time Units"=w604, "Delay Time"=w603, "Time Old In"=w605) -> ("T>dT?"=w606:bool)  [unwired: 2 out]
            n430 = case shown="True" w606 {
              tunnel: [w621 w624] -> w597
              tunnel: [w620 w625] -> _
              tunnel: w607 -> [w621 _]
              tunnel: w609 -> [w620 _]
              frame False {
              }
              frame True {
                n431 = local read "Data Logging Settings"() -> (w626:T37)
                n432 = Unbundle By Name(w626) -> ("Run Description"=w622:string, "Log Files Folder"=w630:path, "Log Files Name"=w628:string, "Automode Files Name"=w629:string, "Filenames Suffix"=w627:string)
                n433 = call <userlib>:"MGI Make String Filesafe.vi"("String In"=w622) -> ("Filesafe String Out"=w623:string)
                n434 = call "GeneratePaths.vi"("Filename Suffix"=w627, "Run description"=w623, "AVS_Path"=w630, "AVS_FName"=w628, "CAL_Path"=w630, "CAL_FName"=w629) -> ("Generated Log path"=w624:path, "Generated Calib path"=w625:path)  [unwired: 8 in]
                n435 = local write "_CalibFilesPath"(w625) -> ()
                n436 = property on="_LogFilesPath" class="Path"("Val(Sgnl)"=w624) -> ()  [unwired: 2 in, 2 out]
              }
            }
            n437 = call "Write To Spreadsheet File (string) w Error.vi"("delimiter (\\t)"=w592, "append to file? (new file:F)"=TRUE, "error in"=w593, "1D data"=w591, "file path (dialog if empty)"=w597) -> ("error out"=w611:errorcluster)  [unwired: 5 in, 1 out]
            n438 = Merge Errors(w611, w586) -> (w610:errorcluster)
          }
          frame #2 {
            # "Add frame with code for writing to PGSQL"
            n439 = local read "Sensor Names"() -> (w644:T10)
            n440 = property on="Sensor Calibrations" class="Clust (strict)"() -> ("Controls[]"=w645:refnum<vi>[])  [unwired: 2 in, 2 out]
            n441 = call "TC to PGSQL.vi"("Calibration"=w645, "AVS names"=w644, "R"=w643, "T"=w642, "I"=w641) -> ()  [unwired: 15 in]
          }
        }
      }
      event User Event {
        # "Process data from the zBridge bridge"
        n442 = event-data() -> ("R"=w655:dbl[], "T"=w654:dbl[])  [unwired: 1 in]
        n443 = property on="CS.Actual Current" class="Arr (strict)"() -> ("Value"=w653:dbl[])  [unwired: 2 in, 2 out]
        n444 = local read "_zBridgeParText"() -> (w650:string)
        n445 = local read "_zBridgeSetNr"() -> (w656:u8)
        n446 = local read "_ZBridgeUnit"() -> (w651:string)
        n447 = Unbundle By Name(w649) -> ("CS Automode"=w648:refnum<user-event>)
        n448 = stacked-sequence {
          tunnel: w650 -> [w677 _ _]
          tunnel: w656 -> [w662 _ w690]
          tunnel: w655 -> [w660 w684 w716]
          tunnel: w654 -> [w659 w683 w715]
          tunnel: w653 -> [_ w682 w714]
          tunnel: w652 -> [_ _ w713]
          tunnel: [_ _ w712] -> w647
          tunnel: w651 -> [w664 _ _]
          tunnel: w648 -> [w661 _ _]
          frame #0 {
            # "Only do PID after measuring\non selected channel( or any \nchannel if -1 is selected)"
            n449 = local read "zBridge params"() -> (w663:T19)
            n450 = local read "Units"() -> (w665:T13)
            n451 = Cluster To Array(cluster=w665) -> (array=w668:string[])
            n452 = Cluster To Array(cluster=w663) -> (array=w678:string[])
            n453 = Replace Array Subset(array=w668, new element=w664, index=w662) -> (w667:string[])
            n454 = Replace Array Subset(array=w678, new element=w677, index=w662) -> (w679:string[])
            n455 = Array To Cluster(array=w667) -> (cluster=→"Units":T65)
            n456 = Array To Cluster(array=w679) -> (cluster=→"zBridge params":T66)
            n457 = property on="Runtime Settings" class="Clust (strict)"() -> ("Value"=w671:T27)  [unwired: 2 in, 2 out]
            n458 = Unbundle By Name(w671) -> ("Y_max"=w674:dbl, "Y_min"=w673:dbl, "Filter Graphs"=w672:bool)
            n459 = local read "Data Array"() -> (w669:T28)
            n460 = property on="Data Memory" class="DigNum (strict)"() -> ("Value"=w676:u16)  [unwired: 2 in, 2 out]
            n461 = call "Current Time(double).vi"() -> ("Current Time (double)"=w657:dbl)  [unwired: 6 in, 1 out]
            n462 = call "Manage Data Arrays - zBridge.vi"("Y_max"=w674, "Y_min"=w673, "Filter Graph Results"=w672, "Append New Data"=TRUE, "Data In"=w669, "Curr R"=w660, "Curr T"=w659, "Curr Time"=w657, "Channel"=w662, "Data Memory"=w676) -> ("Data Out"=w670:T28)  [unwired: 9 in]
            n463 = local write "Data Array"(w670) -> ()
            n464 = Bundle("Current Time (double)"=w657, "R"=w660, "T"=w659) -> (w658:T63)  [unwired: 1 in]
            n465 = Generate User Event(user event=w661, event data cluster=w658) -> ()  [unwired: 2 in, 2 out]
          }
          frame #1 {
            # "New frame with code for writing to DSC"
            n466 = local read "Sensor Names"() -> (w681:T10)
            n467 = property on="Sensor Calibrations" class="Clust (strict)"() -> ("Controls[]"=w685:refnum<vi>[])  [unwired: 2 in, 2 out]
            n468 = call "TC to PGSQL.vi"("Calibration"=w685, "AVS names"=w681, "R"=w684, "T"=w683, "I"=w682) -> ()  [unwired: 15 in]
          }
          frame #2 {
            n469 = local read "_LogFilesPath"() -> (w693:path)
            n470 = local read "Data Logging Settings"() -> (w711:T37)
            n471 = call <userlib>:"Strip Path Extension - Path__ogtk.vi"("path"=w693) -> ("root"=w694:string, "extension"=w697:string)
            n472 = Format Into String(format string="_%d", initial string=w694, w690) -> (resulting string=w695:string)  [unwired: 1 in, 1 out]
            n473 = Concatenate Strings(w695, "." ("string"), w697) -> (w692:string)
            n474 = Unbundle By Name(w711) -> ("Delimeter"=w727:string, "Date Format"=w726:string)
            n475 = String To Path(string=w692) -> (path=w691:path)
            n476 = call <vilib>:"Check if File or Folder Exists.vi"("path"=w691) -> ("file or folder exists?"=w702:bool, "dup path"=w703:path)  [unwired: 8 in, 1 out]
            n477 = case shown="False" w702 {
              tunnel: w703 -> [w745 w748]
              tunnel: [w745 w748] -> w704
              tunnel: [w739 _] -> w687
              frame False {
                n478 = local read "CS Cannel Names"() -> (w743:T31)
                n479 = local read "Sensor Names"() -> (w744:T10)
                n480 = control-ref of="Sensor Calibrations"() -> (w747:refnum<vi>)
                n481 = property on="Run Description" class="Str"() -> ("Value"=w740:string)  [unwired: 2 in, 2 out]
                n482 = Cluster To Array(cluster=w744) -> (array=w741:string[])
                n483 = Cluster To Array(cluster=w743) -> (array=w742:string[])
                n484 = call "Format log file header Z.vi"("Thermometer"=w747, "AVS names"=w741, "CS Names"=w742, "Run description"=w740) -> ("String"=w746:string)  [unwired: 1 in]
                n485 = Write to Text File(file (use dialog)=w745, text=w746) -> (error out=w739:errorcluster)  [unwired: 2 in, 2 out]
              }
              frame True {
              }
            }
            n486 = call "Current Time(double).vi"() -> ("Current Time"=w688:timestamp, "Current Time (double)"=w689:dbl)  [unwired: 6 in]
            n487 = Number To Exponential String(number=w689, precision (6)=i16 10) -> (E-format string=w719:string)  [unwired: 2 in]
            n488 = Format Date/Time String(time format string (%c)=w726, seconds (now)=w688) -> (date/time string=w723:string)  [unwired: 1 in]
            n489 = Number To Exponential String(number=w716) -> (E-format string=w725:string[])  [unwired: 3 in]
            n490 = Number To Engineering String(4:w715) -> (0:w724:string[])  [unwired: 3 in]
            n491 = Number To Fractional String(number=w714) -> (F-format string=w722:string[])  [unwired: 3 in]
            n492 = call <userlib>:"File Info__ogtk.vi"("error in (no error)"=w687, "file"=w704) -> ("error out"=w686:errorcluster, "file info"=w700:T64, "file out"=w709:path)  [unwired: 4 in]
            n493 = Unbundle By Name(w700) -> ("creation date"=w701:u32)
            n494 = Build Array (concatenate)(w723, w719, w725, w724, w722) -> (w721:string[])
            n495 = local read "_CalibFilesPath"() -> (w710:path)
            n496 = property on="New File Interval" class="DigNum (strict)"() -> ("Value"=w705:u32)  [unwired: 2 in, 2 out]
            n497 = property on="New File Interval Units" class="Enum (strict)"() -> ("Value"=w706:enum16{"Minutes", "Hours", "Days"})  [unwired: 2 in, 2 out]
            n498 = To Time Stamp(1:w701) -> (0:w707:timestamp)
            n499 = call "Time Elapsed time.vi"("Time Units"=w706, "Delay Time"=w705, "Time Old In"=w707) -> ("T>dT?"=w708:bool)  [unwired: 2 out]
            n500 = case shown="True" w708 {
              tunnel: [w729 w732] -> w699
              tunnel: [w728 w734] -> _
              tunnel: w709 -> [w729 _]
              tunnel: w710 -> [w728 _]
              frame False {
              }
              frame True {
                n501 = local read "Data Logging Settings"() -> (w735:T37)
                n502 = Unbundle By Name(w735) -> ("Run Description"=w731:string, "Filenames Suffix"=w733:string, "Log Files Folder"=w738:path, "Log Files Name"=w736:string, "Automode Files Name"=w737:string)
                n503 = call <userlib>:"MGI Make String Filesafe.vi"("String In"=w731) -> ("Filesafe String Out"=w730:string)
                n504 = call "GeneratePaths.vi"("Filename Suffix"=w733, "Run description"=w730, "AVS_Path"=w738, "AVS_FName"=w736, "CAL_Path"=w738, "CAL_FName"=w737) -> ("Generated Log path"=w732:path, "Generated Calib path"=w734:path)  [unwired: 8 in]
                n505 = local write "_CalibFilesPath"(w734) -> ()
                n506 = property on="_LogFilesPath" class="Path"("Val(Sgnl)"=w732) -> ()  [unwired: 2 in, 2 out]
              }
            }
            n507 = call "Write To Spreadsheet File (string) w Error.vi"("delimiter (\\t)"=w727, "append to file? (new file:F)"=TRUE, "error in"=w686, "1D data"=w721, "file path (dialog if empty)"=w699) -> ("error out"=w717:errorcluster)  [unwired: 5 in, 1 out]
            n508 = Merge Errors(w717, w713) -> (w712:errorcluster)
          }
        }
      }
      event User Event {
        # "Current source automatic mode"
        n509 = event-data() -> ("R"=w755:dbl[], "T"=w756:dbl[], "Time"=w750:dbl)  [unwired: 1 in, 4 out]
        n510 = local read "CS.Mode"() -> (w754:T39)
        n511 = Unbundle By Name(w753) -> ("CallExtVI"=w752:refnum<user-event>, "TempStabilized"=w751:refnum<user-event>)
        n512 = case shown="\"Mode2\"" w754 {
          tunnel: w756 -> [_ w760 w835]
          tunnel: w755 -> [_ w761 w836]
          tunnel: w752 -> [_ w763 _]
          tunnel: w751 -> [_ w762 _]
          tunnel: w750 -> [_ w759 _]
          frame "Manual", Default {
          }
          frame "Mode 1" {
            n513 = call <userlib>:"MGI Change Detector (T).vi"("Value"="CS.Mode1.Start") -> ("Changed?"=w757:bool)
            n514 = case shown="True" "CS.Mode1.Start" {
              tunnel: w763 -> [_ w776]
              tunnel: w762 -> [_ w775]
              tunnel: w761 -> [_ w774]
              tunnel: w760 -> [_ w773]
              tunnel: w759 -> [_ w770]
              tunnel: w757 -> [_ w764]
              frame False {
              }
              frame True {
                # "Check if PID error (SP-PV)==0"
                # "Check if temperature\nis stabilized"
                # "T sabilized?"
                # "If TCS auto mode enabled and temperature is not changing => fire TempStabilized event to save log and set new CS point. Otherwise do PID (if enabled)."
                # "Check if stabilization delay time \nis elapsed"
                n515 = property on="R/T?" class="Enum (strict)"() -> ("Value"=w772:enum16{"Resistance", "Temperature"})  [unwired: 2 in, 2 out]
                n516 = case shown="\"Temperature\"" w772 {
                  tunnel: [w791 w792] -> w769
                  tunnel: w774 -> [w791 _]
                  tunnel: w773 -> [_ w792]
                  frame "Resistance", Default {
                  }
                  frame "Temperature" {
                  }
                }
                n517 = property on="Bridge Channel" class="DigNum (strict)"() -> ("Value"=w768:i32)  [unwired: 2 in, 2 out]
                n518 = Index Array(array=w769, index=w768) -> (element=w767:dbl)
                n519 = local read "CS.Mode1.PID Error"() -> (w783:dbl)
                n520 = property on="FB on 2" class="Enum (strict)"() -> ("Value"=w765:enum16{"0", "1", "2", "3"})  [unwired: 2 in, 2 out]
                n521 = local read "_CSMode1List[i]"() -> (w777:T23[])
                n522 = local read "_TimeOld"() -> (w789:dbl)
                n523 = property on="Delay Time" class="DigNum (strict)"() -> ("Value"=w779:dbl)  [unwired: 2 in, 2 out]
                n524 = property on="N averages" class="DigNum (strict)"() -> ("Value"=w766:i32)  [unwired: 2 in, 2 out]
                n525 = property on="T stability" class="DigNum (strict)"() -> ("Value"=w778:dbl)  [unwired: 2 in, 2 out]
                n526 = Equal To 0?(x=w783) -> (x = 0?=w781:bool)
                n527 = call "Derivatives Pt by Pt.vi"("initialize"=w764, "accuracy (%)"=w778, "Time"=w770, "Data"=w767, "Points to avg"=w766) -> ("Stable?"=w782:bool, "Stability (%)"=→"CS.Mode1.Slope":dbl, "dt (s)"=w786:dbl)  [unwired: 2 in]
                n528 = Index Array(array=w777, index=w765) -> (element=w790:T23)
                n529 = call "Time Elapsed dbl.vi"("Delay Time"=w779, "Time Old In"=w789) -> ("T>dT?"=w771:bool, "Delta T"=→"CS.Mode1.Timer":dbl, "Time New Out"=w788:dbl)  [unwired: 1 in]
                n530 = Compound Arithmetic op=AND(w771, w781, w782) -> (w784:bool)
                "CS.Mode1.PID Stabilized?" <- w784
                n531 = property on="Enable PID" class="Bool (strict)"() -> ("Value"=w780:bool)  [unwired: 2 in, 2 out]
                n532 = case shown="False" w784 {
                  tunnel: w788 -> [_ w812]
                  tunnel: w786 -> [w808 _]
                  tunnel: w780 -> [w798 _]
                  tunnel: w790 -> [w806 _]
                  tunnel: w777 -> [w803 _]
                  tunnel: w765 -> [w796 _]
                  tunnel: w776 -> [_ w810]
                  tunnel: w775 -> [_ w809]
                  tunnel: w767 -> [w795 _]
                  tunnel: w764 -> [w793 _]
                  frame False {
                    # "Temperature is not stable. If enabled, do PID regulation"
                    n533 = local read "CS.Current Value"() -> (w800:dbl[])
                    n534 = Index Array(array=w800, index=w796) -> (element=w801:dbl)
                    n535 = Multiply(x=1000.0, y=w801) -> (x*y=w799:dbl)
                    n536 = call "PID control incremental.vi"("Process Variable"=w795, "dt"=w808, "Setpoint"=w806, "PID Settings"="CS.Mode1.PID Settings", "I in"=w799, "PID Enabled"=w798, "Reset"=w793) -> ("PID output I"=→"Waveform Chart":T22, "err out"=→"CS.Mode1.PID Error":dbl, "I out"=w805:dbl)  [unwired: 9 in, 1 out]
                    n537 = Replace Array Subset(array=w803, new element=w805, index=w796) -> (→"CS.Automode Current":T23[])
                  }
                  frame True {
                    # "Temperature is stable & automode is on"
                    n538 = case shown="False" "CS.Mode1.Call VI?" {
                      tunnel: w812 -> [w815 _]
                      tunnel: w810 -> [_ w816]
                      tunnel: w809 -> [w813 _]
                      frame False {
                        # "External VI call disabled -> proceed\nwith automode"
                        n539 = local write "_TimeOld"(w815) -> ()
                        n540 = Generate User Event(user event=w813, event data cluster=TRUE ("event data")) -> ()  [unwired: 2 in, 2 out]
                      }
                      frame True {
                        # "Call external VI"
                        n541 = Generate User Event(user event=w816, event data cluster="" ("event data")) -> ()  [unwired: 2 in, 2 out]
                      }
                    }
                  }
                }
              }
            }
          }
          frame "Mode2" {
            n542 = Unbundle By Name("CS.Mode2.Settings") -> ("Hysteresis"=w818:u8, "Bridge Channel"=w819:i32, "FB on"=w820:enum16{"Resistance", "Temperature"})
            n543 = case shown="\"Resistance\", Default" w820 {
              tunnel: [w838 w839] -> w834
              tunnel: w836 -> [w838 _]
              tunnel: w835 -> [_ w839]
              frame "Resistance", Default {
              }
              frame "Temperature" {
              }
            }
            n544 = Index Array(array=w834, index=w819) -> (element=w833:dbl)
            n545 = local read "CS.Mode2.List"() -> (w832:dbl[][])
            n546 = call "Currents-Temp list  - T in range-.vi"("List in"=w832, "T"=w833, "T1 index"=1, "T0 index"=0, "Hysteresis"=w818) -> ("List index"=w826:i32, "I_out"=w825:dbl[])  [unwired: 1 out]
            n547 = case shown="True" "CS.Mode2.Start" {
              tunnel: w825 -> [_ w837]
              frame False {
              }
              frame True {
                n548 = local write "CS.Automode Current"(w837) -> ()
              }
            }
            n549 = Initialize Array(FALSE, 16 ("dimension size")) -> (w829:bool[])
            n550 = Replace Array Subset(array=w829, new element=TRUE ("new element/subarray"), index=w826) -> (→"CS.Mode2.Row":bool[])
          }
        }
      }
      event User Event {
        n551 = event-data() -> ()  [unwired: 1 in, 5 out]
        n552 = Unbundle By Name(w842) -> ("TempStabilized"=w841:refnum<user-event>)
        n553 = local read "_ExtVIReference"() -> (w846:refnum<vi>)
        n554 = call "GetExtVIStatus.vi"("vi reference in"=w846) -> ("vi reference out"=w843:refnum<vi>, "Exec.State"=w845:T46, "Finished?"=w844:bool)
        n555 = case shown="\"Idle\"" w845 {
          tunnel: w844 -> [_ _]
          tunnel: w843 -> [_ w848]
          tunnel: w841 -> [_ w847]
          frame "Bad", Default {
          }
          frame "Idle" {
            n556 = local read "VI called?"() -> (w849:bool)
            n557 = case shown="False" w849 {
              tunnel: w848 -> [w851 _]
              tunnel: w847 -> [_ w858]
              frame False {
                n558 = property on="_ScanData" class="Arr (strict)"() -> ("Value"=w854:dbl[])  [unwired: 2 in, 2 out]
                n559 = property on="T Array" class="Arr (strict)"() -> ("Value"=w855:dbl[])  [unwired: 2 in, 2 out]
                n560 = property on="CS.Current Value" class="Arr (strict)"() -> ("Value"=w856:dbl[])  [unwired: 2 in, 2 out]
                n561 = Format Date/Time String() -> (date/time string=w853:string)  [unwired: 3 in]
                n562 = Bundle("date/time string"=w853, "Value"=w854, "Value"=w855, "Value"=w856) -> (w852:T67)  [unwired: 1 in]
                n563 = call "CallExtVI.vi"("vi reference in"=w851, "Cluster"=w852) -> ()  [unwired: 1 out]
                "VI called?" <- TRUE ("VI called?")
              }
              frame True {
                n564 = call "Current Time(double).vi"() -> ("Current Time (double)"=w857:dbl)  [unwired: 6 in, 1 out]
                n565 = Generate User Event(user event=w858, event data cluster=TRUE ("event data")) -> ()  [unwired: 2 in, 2 out]
                n566 = local write "_TimeOld"(w857) -> ()
              }
            }
          }
        }
      }
      event User Event {
        # "CS automode\nT is stabilized"
        n567 = event-data() -> ("TempStabilized"=w862:bool)  [unwired: 1 in, 4 out]
        n568 = stacked-sequence {
          tunnel: w863 -> [w869 _]
          tunnel: [w870 _] -> w861
          tunnel: w862 -> [_ w890]
          frame #0 {
            # "Step1: Save R,T,I values to calibration file. Make screenshot when creating the calibration file."
            n569 = property on="_CalibFilesPath" class="Path"() -> ("Value"=w865:path)  [unwired: 2 in, 2 out]
            n570 = call <userlib>:"File Exists - Scalar__ogtk.vi"("file path"=w865) -> ("exists"=w866:bool)  [unwired: 6 in, 1 out]
            n571 = case shown="False" w866 {
              tunnel: w865 -> [w879 w889]
              tunnel: [w879 w889] -> w864
              frame False {
                n572 = local read "CS Cannel Names"() -> (w885:T31)
                n573 = local read "Sensor Names"() -> (w886:T10)
                n574 = property on="Run Description" class="Str"() -> ("Value"=w882:string)  [unwired: 2 in, 2 out]
                n575 = control-ref of="Sensor Calibrations"() -> (w888:refnum<vi>)
                n576 = Cluster To Array(cluster=w886) -> (array=w883:string[])
                n577 = Cluster To Array(cluster=w885) -> (array=w884:string[])
                n578 = call "Format log file header Z.vi"("Thermometer"=w888, "AVS names"=w883, "CS Names"=w884, "Run description"=w882) -> ("String"=w887:string)  [unwired: 1 in]
                n579 = control-ref of="This VI"() -> (w881:refnum<vi>)
                n580 = Write to Text File(file (use dialog)=w879, text=w887) -> ()  [unwired: 2 in, 3 out]
                n581 = invoke class="VI" method="FP.Get Image"(reference=w881) -> ("image data"=w880:T68)  [unwired: 5 in, 5 out]
                n582 = call <userlib>:"Convert File Extension (Path)__ogtk.vi"("new ending (none)"="png" ("name or relative path"), "file name"=w879) -> ("new filename"=w878:path)  [unwired: 1 out]
                n583 = call <vilib>:"Write PNG File.vi"("image data"=w880, "path to PNG file"=w878) -> ()  [unwired: 8 in, 2 out]
              }
              frame True {
              }
            }
            n584 = local write "VI called?"(FALSE ("VI called?")) -> ()
            n585 = property on="Data Logging Settings" class="Clust (strict)"() -> ("Value"=w873:T37)  [unwired: 2 in, 2 out]
            n586 = Unbundle By Name(w873) -> ("Date Format"=w874:string, "Delimeter"=w871:string)
            n587 = property on="R" class="Clust (strict)"() -> ("Value"=w872:T14)  [unwired: 2 in, 2 out]
            n588 = property on="T" class="Clust (strict)"() -> ("Value"=w876:T9)  [unwired: 2 in, 2 out]
            n589 = property on="CS.Current Value" class="Arr (strict)"() -> ("Value"=w875:dbl[])  [unwired: 2 in, 2 out]
            n590 = call "Write to cal log file.vi"("Value 2"=w875, "Date/Time Format"=w874, "Value 3"=w876, "Value"=w872, "Delimeter"=w871, "Value 4"=w864) -> ("error out"=w868:errorcluster)  [unwired: 1 out]
            n591 = Merge Errors(w868, w869) -> (w870:errorcluster)
          }
          frame #1 {
            # "Step 2: Sweep through the currents list"
            n592 = case shown="True" w890 {
              frame False {
              }
              frame True {
                n593 = local read "CS.Mode1.List:Count"() -> (w892:i32)
                n594 = local read "CS.Mode1.List:Index"() -> (w893:i32)
                n595 = Less?(x=w893, y=w892) -> (x < y?=w891:bool)
                n596 = case shown="False" w891 {
                  frame False {
                    n597 = property on="CS Mode" class="Enum (strict)"("Val(Sgnl)"=CS_mode."Manual" ("CS Mode")) -> ()  [unwired: 2 in, 2 out]
                  }
                  frame True {
                    n598 = property on="CS.Mode1.List:Next" class="Bool (strict)"("Val(Sgnl)"=TRUE) -> ()  [unwired: 2 in, 2 out]
                  }
                }
              }
            }
          }
        }
      }
      event User Event {
        # "Disable controls for disabled channels"
        n599 = event-data() -> ()  [unwired: 1 in, 5 out]
        n600 = Unbundle By Name(w897) -> ("zBridge dll"=w896:path)
        n601 = property on="Bridge Type" class="Enum (strict)"() -> ("Value"=w905:T60)  [unwired: 2 in, 2 out]
        n602 = case shown="Default" w905 {
          tunnel: [w915 w927 w935] -> w904
          tunnel: w896 -> [_ w926 _]
          frame Default {
            n603 = property on="Runtime Settings" class="Clust (strict)"() -> ("Value"=w919:T27)  [unwired: 2 in, 2 out]
            n604 = Unbundle By Name(w919) -> ("Read AVS channels from"=w917:i8, "Last Channel"=w918:i8)
            n605 = for {
              N: 10 -> [_]
              tunnel: w918 -> [w921]
              tunnel: w917 -> [w922]
              tunnel: [w920] -> w915 mode=indexing
              i -> [w923]
              n606 = Less Or Equal?(x=w922, y=w923) -> (x <= y?=w925:bool)
              n607 = Less Or Equal?(x=w923, y=w921) -> (x <= y?=w924:bool)
              n608 = And(x=w925, y=w924) -> (x .and. y?=w920:bool)
            }
          }
          frame "Impedance Bridge" {
            n609 = for {
              N: 10 -> [_]
              tunnel: [w930] -> w928 mode=indexing
              tunnel: w926 -> [w931]
              i -> [w933]
              n610 = call "GetByteParam.vi"("ParNo"=u8 0, "SetNo"=w933, "zDll"=w931) -> ("return type"=w930:u8)  [unwired: 6 in, 2 out]
            }
            n611 = Greater Than 0?(x=w928) -> (x > 0?=w927:bool[])
          }
          frame "AVS47B (RS232 interface)" {
            n612 = local read "zBridge.Active Channels"() -> (w934:T21)
            n613 = Cluster To Array(cluster=w934) -> (array=w935:bool[])
          }
        }
        n614 = control-ref of="zBridge.Active Channels"() -> (w911:refnum<vi>)
        n615 = control-ref of="AVS Exc&Ranges"() -> (w907:refnum<vi>)
        n616 = control-ref of="R"() -> (w912:refnum<vi>)
        n617 = control-ref of="Sensor Calibrations"() -> (w913:refnum<vi>)
        n618 = control-ref of="T"() -> (w914:refnum<vi>)
        n619 = control-ref of="uPlots"() -> (w908:refnum<vi>)
        n620 = control-ref of="AVS names"() -> (w906:refnum<vi>)
        n621 = control-ref of="zBridge params"() -> (w903:refnum<vi>)
        n622 = control-ref of="zBridge.Scan Phase"() -> (w902:refnum<vi>)
        n623 = control-ref of="Units"() -> (w901:refnum<vi>)
        n624 = control-ref of="AVS names small"() -> (w900:refnum<vi>)
        n625 = control-ref of="Small R Cluster"() -> (w899:refnum<vi>)
        n626 = control-ref of="Small T Cluster"() -> (w898:refnum<vi>)
        n627 = Build Array(w911, w907, w912, w913, w914, w908, w906, w903, w902, w901, w900, w899, w898) -> (w909:refnum<vi>[])
        n628 = Array Size(array=w909) -> (size(s)=w910:i32)
        n629 = for {
          N: w910 -> [_]
          tunnel: w909 -> [w939] mode=indexing
          tunnel: w904 -> [w936]
          n630 = property class="Clust"(reference=w939) -> ("Controls[]"=w937:refnum<vi>[])  [unwired: 1 in, 2 out]
          n631 = Array Size(array=w937) -> (size(s)=w938:i32)
          n632 = for {
            N: w938 -> [_]
            tunnel: w937 -> [w941] mode=indexing
            tunnel: w936 -> [w940] mode=indexing
            n633 = case shown="True" w940 {
              tunnel: w941 -> [w942 w947]
              frame False {
                n634 = property class="Ctl"(reference=w942, "Disabled"=u8 2) -> ("ClassName"=w943:string)  [unwired: 1 in, 2 out]
                n635 = case shown="\"Boolean\"" w943 {
                  tunnel: w942 -> [_ w946 _]
                  frame "False", Default {
                  }
                  frame "Boolean" {
                    n636 = property class="Ctl"(reference=w946, "Value"=FALSE) -> ()  [unwired: 1 in, 2 out]
                  }
                  frame "Ring" {
                  }
                }
              }
              frame True {
                n637 = property class="Ctl"(reference=w947, "Disabled"=u8 0) -> ("ClassName"=w948:string)  [unwired: 1 in, 2 out]
                n638 = case shown="\"False\", Default" w948 {
                  tunnel: w947 -> [_ w951]
                  frame "False", Default {
                  }
                  frame "Boolean" {
                    n639 = property class="Ctl"(reference=w951, "Value"=TRUE) -> ()  [unwired: 1 in, 2 out]
                  }
                }
              }
            }
          }
        }
      }
      event Mouse Down? {
        n640 = event-data() -> ("CtlRef"=w953:refnum<vi>, "Mods.Double Click"=w952:bool)  [unwired: 1 in]
        n641 = disable-structure shown="Enabled" {
          disable-tunnel: w952 -> [w956 _]
          disable-tunnel: w953 -> [w955 _]
          frame Enabled {
            n642 = case shown="True" w956 {
              tunnel: w955 -> [_ w975]
              frame False {
              }
              frame True {
                w971 = 128  # call and forget
                n643 = property class="Ctl"(reference=w975) -> ("Label.Text"=w974:string)  [unwired: 1 in, 2 out]
                n644 = local read "Sensor Names"() -> (w962:T10)
                n645 = call <userlib>:"Slice String 1__ogtk.vi"("Subset (i:j)"="-1", "String"=w974) -> ("Substring (String[i:j])"=w972:string)  [unwired: 7 in]
                n646 = Decimal String To Number(string=w972) -> (number=w957:i32)  [unwired: 2 in, 1 out]
                n647 = Cluster To Array(cluster=w962) -> (array=w961:string[])
                n648 = Index Array(array=w961, index=w957) -> (element=w960:string)
                n649 = vi-ref "Text Popup.vi"() -> (w968:refnum<vi>)
                n650 = property class="VI"(reference=w968) -> (error out=w969:errorcluster, "Name"=w970:string)  [unwired: 1 in, 1 out]
                n651 = Open VI Reference(type specifier VI Refnum (for type only)=refnum<vi> refnum, vi path=w970, options=w971, error in (no error)=w969) -> (vi reference=w967:refnum<vi>, error out=w964:errorcluster)  [unwired: 2 in]
                n652 = control-ref of="T Array"() -> (w958:refnum<vi>)
                n653 = control-ref of="R Array"() -> (w959:refnum<vi>)
                n654 = call-by-ref "Start Asynchronous Call"(reference=w967, error in=w964, "Title"=w960, "R_array"=w959, "T_array"=w958, "Index"=w957) -> (reference out=w965:refnum<vi>, error out=w963:errorcluster)  [unwired: 16 in]
                n655 = Close Reference(reference=w965, error in (no error)=w963) -> ()  [unwired: 1 out]
              }
            }
          }
          frame Disabled {
          }
        }
        n656 = event-data() -> ()  [unwired: 2 in, 1 out]
      }
      event "_LogFilesPath": Value Change {
        # "Modify window title to show measurement information"
        n657 = event-data() -> ("NewVal"=w985:path)  [unwired: 1 in, 5 out]
        n658 = property class="App"() -> ("App.Dir"=w977:path)  [unwired: 2 in, 2 out]
        n659 = property on="Run Description" class="Str"() -> ("Value"=w978:string)  [unwired: 2 in, 2 out]
        n660 = property on="Bridge Type" class="Enum (strict)"() -> ("RingText.Text"=w979:string)  [unwired: 2 in, 2 out]
        n661 = property on="CS type" class="Enum (strict)"() -> ("RingText.Text"=w980:string)  [unwired: 2 in, 2 out]
        n662 = Path To String(path=w985) -> (string=w981:string)
        n663 = Strip Path(path=w977) -> (name=w976:string)  [unwired: 1 out]
        n664 = Format Into String(format string="%s - %s - %s - %s   (%s)", w976, w978, w979, w980, w981) -> (resulting string=w983:string)  [unwired: 2 in, 1 out]
        n665 = control-ref of="This VI"() -> (w986:refnum<vi>)
        n666 = property class="VI"(reference=w986, "Front Panel.Title"=w983) -> ()  [unwired: 1 in, 2 out]
      }
      event "Reload Calibrations", "Bridge settings.Calibrations Folder": Value Change {
        # "Refresh the list of calibration files"
        n667 = event-data() -> ()  [unwired: 1 in, 1 out]
        n668 = property on="Calibrations Folder" class="Path"() -> ("Value"=w987:path)  [unwired: 2 in, 2 out]
        n669 = control-ref of="Sensor Calibrations"() -> (w996:refnum<vi>)
        n670 = control-ref of="_CurCalibrations"() -> (w990:refnum<vi>)
        n671 = control-ref of="Calibrations Folder"() -> (w994:refnum<vi>)
        n672 = control-ref of="_QuickConvertCal"() -> (w993:refnum<vi>)
        n673 = control-ref of="Sensor 1"() -> (w995:refnum<vi>)
        n674 = Bundle By Name(cluster=w989, "Calibrations Folder"=w987) -> (w988:T50)
        n675 = call "ReloadCalibrations.vi"("error in (no error)"=w992, "Quick convert sensors"=w993, "CurCalibrations"=w990, "Calibration files path"=w994, "Channel1 sensors"=w995, "Channels list"=w996) -> ("error out"=w991:errorcluster)  [unwired: 1 in]
      }
      event Value Change {
        w1003 = refnum<vi> refnum  # XYGraph
        # "Show cursor on plot is \"Cursor\" or \"Delete points\" mode is enabled"
        # "!!NOTE:This routine assumes that XY graph is control #0 on tab page!!"
        n676 = event-data() -> ("NewVal"=w999:T7)  [unwired: 1 in, 5 out]
        n677 = property on="Channels Panel" class="TabCtl (strict)"() -> ("Pages"=w1007:refnum<vi>[], "Value"=w1006:T8)  [unwired: 2 in, 2 out]
        n678 = Index Array(array=w1007, index=w1006) -> (element=w1005:refnum<vi>)
        n679 = property class="Page"(reference=w1005) -> ("ControlsOnPage"=w1000:refnum<vi>[])  [unwired: 1 in, 2 out]
        n680 = Index Array(array=w1000, index=0) -> (element=w1004:refnum<vi>)
        n681 = Type Cast(type=w1003, x=w1004) -> (*(type *) &x=w998:refnum<vi>)
        n682 = case shown="\"Erase range\"" w999 {
          tunnel: w998 -> [w1008 w1017 w1025 w1033]
          frame "No Selection", Default {
            n683 = property class="XYGraph"(reference=w1008, "Active Cursor"=u32 0, "Cursor.Visible"=FALSE) -> (reference out=w1011:refnum<vi>)  [unwired: 1 in, 1 out]
            n684 = property class="XYGraph"(reference=w1011, "Active Cursor"=u32 1, "Cursor.Visible"=FALSE) -> ()  [unwired: 1 in, 2 out]
          }
          frame "Erase range" {
            n685 = property class="XYGraph"(reference=w1017, "Active Cursor"=u32 0, "Cursor.Visible"=TRUE, "Cursor.Cursor Color"=u32 16777062, "Cursor.Cursor Index"=0, "ActPaletteTool"=0 ("Palette:Active Tool")) -> (reference out=w1020:refnum<vi>)  [unwired: 1 in, 1 out]
            n686 = property class="XYGraph"(reference=w1020, "Active Cursor"=u32 1, "Cursor.Visible"=TRUE, "Cursor.Cursor Color"=u32 6618880) -> ()  [unwired: 1 in, 2 out]
          }
          frame "Cursor mode" {
            n687 = property class="XYGraph"(reference=w1025, "Active Cursor"=u32 0, "Cursor.Visible"=TRUE, "Cursor.Cursor Color"=u32 6618880, "ActPaletteTool"=0 ("Palette:Active Tool")) -> (reference out=w1028:refnum<vi>)  [unwired: 1 in, 1 out]
            n688 = property class="XYGraph"(reference=w1028, "Active Cursor"=u32 1, "Cursor.Visible"=FALSE) -> ()  [unwired: 1 in, 2 out]
          }
          frame "Erase point" {
            n689 = property class="XYGraph"(reference=w1033, "Active Cursor"=u32 0, "Cursor.Visible"=TRUE, "Cursor.Cursor Color"=u32 16777062, "ActPaletteTool"=0 ("Palette:Active Tool")) -> (reference out=w1036:refnum<vi>)  [unwired: 1 in, 1 out]
            n690 = property class="XYGraph"(reference=w1036, "Active Cursor"=u32 1, "Cursor.Visible"=FALSE) -> ()  [unwired: 1 in, 2 out]
          }
        }
      }
      event "R-Plot 0", "R-Plot 1", "R-Plot 2", "R-Plot 3", "R-Plot 4", "R-Plot 5", "R-Plot 6", "R-Plot 7", "R-Plot 8", "R-Plot 9": Mouse Down? {
        # "Disabled"
        n691 = event-data() -> ("CtlRef"=w1042:refnum<vi>, "Button"=w1047:u16, "Mods.Double Click"=w1044:bool)  [unwired: 1 in, 5 out]
        n692 = Equal?(x=u16 1, y=w1047) -> (x = y?=w1045:bool)
        n693 = And(x=w1045, y=w1044) -> (x .and. y?=w1043:bool)
        n694 = disable-structure shown="Disabled" {
          disable-tunnel: w1043 -> [w1050 _]
          disable-tunnel: w1042 -> [w1049 _]
          disable-tunnel: "Mode Buttons" -> [w1048 _]
          frame Disabled {
            n695 = case shown="True" w1050 {
              tunnel: w1048 -> [_ w1052]
              tunnel: w1049 -> [_ w1051]
              frame False {
              }
              frame True {
                n696 = case shown="\"Erase range\"" w1052 {
                  tunnel: w1051 -> [_ w1053]
                  frame "No Selection", Default {
                  }
                  frame "Erase range" {
                    n697 = property class="XYGraph (strict)"(reference=w1053, "ActPaletteTool"=0 ("Palette:Active Tool"), "Active Cursor"=u32 0, "Cursor.Visible"=TRUE) -> ()  [unwired: 1 in, 2 out]
                  }
                }
              }
            }
          }
          frame Enabled {
          }
        }
        n698 = event-data() -> ()  [unwired: 5 in, 1 out]
      }
      event "R-Plot 0", "R-Plot 1", "R-Plot 2", "R-Plot 3", "R-Plot 4", "R-Plot 5", "R-Plot 6", "R-Plot 7", "R-Plot 8", "R-Plot 9": Mouse Down {
        # "Process (double) click on plots in special modes (\"Cursor\", \"Erase\")"
        n699 = event-data() -> ("CtlRef"=w1060:refnum<vi>, "Coords"=w1063:T69, "Button"=w1059:u16, "Mods.Double Click"=w1062:bool, "PlatMods"=w1058:T70)  [unwired: 1 in, 3 out]
        n700 = property on="Mode Buttons" class="RadioBtnsControl (strict)"() -> ("Value"=w1061:T7)  [unwired: 2 in, 2 out]
        n701 = case shown="1" w1059 {
          tunnel: w1063 -> [_ _ w1068]
          tunnel: w1062 -> [_ _ w1067]
          tunnel: w1061 -> [_ _ w1066]
          tunnel: w1060 -> [_ _ w1065]
          tunnel: w1058 -> [_ _ _]
          frame 2 {
          }
          frame Default {
          }
          frame 1 {
            n702 = case shown="\"Cursor mode\"" w1066 {
              tunnel: w1065 -> [_ w1071 w1092 w1100]
              tunnel: w1068 -> [_ w1070 w1091 w1102]
              tunnel: w1067 -> [_ w1069 w1093 w1101]
              frame "No Selection", Default {
              }
              frame "Cursor mode" {
                n703 = case shown="True" w1069 {
                  tunnel: w1071 -> [_ w1081]
                  tunnel: w1070 -> [_ w1079]
                  frame False {
                  }
                  frame True {
                    n704 = invoke class="XYGraph (strict)" method="Map Coords To XY"(reference=w1081, "Coords"=w1079) -> (reference out=w1080:refnum<vi>, "XY"=w1078:cluster{"X":dbl, "Y":dbl})  [unwired: 5 in, 5 out]
                    n705 = Unbundle By Name(w1078) -> ("X"=w1076:dbl)
                    n706 = local read "Data Array"() -> (w1077:T28)
                    n707 = property class="XYGraph (strict)"(reference=w1080, "Active Cursor"=u32 0, "Cursor.Cursor Position"=w1078) -> ()  [unwired: 1 in, 2 out]
                    n708 = for {
                      tunnel: w1077 -> [w1090] mode=indexing
                      tunnel: w1076 -> [w1088]
                      tunnel: [w1084] -> w1075 mode=indexing
                      tunnel: [w1083] -> w1074 mode=indexing
                      n709 = Unbundle By Name(w1090) -> ("R"=w1087:dbl[], "T"=w1086:dbl[], "Time"=w1089:dbl[])
                      n710 = Threshold 1D Array(2:w1088, 3:w1089) -> (0:w1085:dbl)  [unwired: 1 in]
                      n711 = Index Array(array=w1087, index=w1085) -> (element=w1084:dbl)
                      n712 = Index Array(array=w1086, index=w1085) -> (element=w1083:dbl)
                    }
                    n713 = Array To Cluster(array=w1074) -> (cluster=w1072:T61)
                    n714 = Array To Cluster(array=w1075) -> (cluster=w1073:T61)
                    n715 = property on="Time" class="DigNum (strict)"("Value"=w1076) -> ()  [unwired: 2 in, 2 out]
                    n716 = property on="Small R Cluster" class="Clust (strict)"("Value"=w1073) -> ()  [unwired: 2 in, 2 out]
                    n717 = property on="Small T Cluster" class="Clust (strict)"("Value"=w1072) -> ()  [unwired: 2 in, 2 out]
                  }
                }
              }
              frame "Erase range" {
                n718 = case shown="False" w1093 {
                  tunnel: w1092 -> [w1097 _]
                  tunnel: w1091 -> [w1096 _]
                  frame False {
                    n719 = invoke class="XYGraph (strict)" method="Map Coords To XY"(reference=w1097, "Coords"=w1096) -> (reference out=w1099:refnum<vi>, "XY"=w1094:cluster{"X":dbl, "Y":dbl})  [unwired: 5 in, 5 out]
                    n720 = property class="XYGraph (strict)"(reference=w1099, "Active Cursor"=u32 0, "Cursor.Cursor Position"=w1094, "Active Cursor"=u32 1, "Cursor.Cursor Position"=w1094) -> ()  [unwired: 1 in, 2 out]
                  }
                  frame True {
                  }
                }
              }
              frame "Erase point" {
                n721 = case shown="True" w1101 {
                  tunnel: w1100 -> [w1107 w1122]
                  tunnel: w1102 -> [w1106 _]
                  frame False {
                    n722 = invoke class="XYGraph (strict)" method="Map Coords To XY"(reference=w1107, "Coords"=w1106) -> (reference out=w1105:refnum<vi>, "XY"=w1104:cluster{"X":dbl, "Y":dbl})  [unwired: 5 in, 5 out]
                    n723 = property class="XYGraph (strict)"(reference=w1105, "Active Cursor"=u32 0, "Cursor.Cursor Position"=w1104) -> ()  [unwired: 1 in, 2 out]
                  }
                  frame True {
                    n724 = property class="XYGraph (strict)"(reference=w1122, "Active Cursor"=u32 0) -> ("Cursor.Cursor X"=w1110:dbl)  [unwired: 1 in, 2 out]
                    n725 = local read "Channels Panel"() -> (w1109:T8)
                    n726 = local read "Data Array"() -> (w1108:T28)
                    n727 = Index Array(array=w1108, index=w1109) -> (element=w1115:cluster{"R":dbl[], "T":dbl[], "Time":dbl[]})
                    n728 = Unbundle By Name(w1115) -> ("R"=w1111:dbl[], "T"=w1112:dbl[], "Time"=w1113:dbl[])
                    n729 = Threshold 1D Array(2:w1110, 3:w1113) -> (0:w1114:dbl)  [unwired: 1 in]
                    n730 = Delete From Array(array=w1111, index=w1114) -> (array with subset deleted=w1118:dbl[])  [unwired: 1 in, 1 out]
                    n731 = Delete From Array(array=w1112, index=w1114) -> (array with subset deleted=w1117:dbl[])  [unwired: 1 in, 1 out]
                    n732 = Delete From Array(array=w1113, index=w1114) -> (array with subset deleted=w1116:dbl[])  [unwired: 1 in, 1 out]
                    n733 = Bundle By Name(cluster=w1115, "R"=w1118, "T"=w1117, "Time"=w1116) -> (w1119:cluster{"R":dbl[], "T":dbl[], "Time":dbl[]})
                    n734 = Replace Array Subset(array=w1108, new element=w1119, index=w1109) -> (w1120:T28)
                    n735 = local write "Data Array"(w1120) -> ()
                  }
                }
              }
            }
            "_LMBDown" <- TRUE ("Mouse down")
          }
        }
      }
      event "R-Plot 0", "R-Plot 1", "R-Plot 2", "R-Plot 3", "R-Plot 4", "R-Plot 5", "R-Plot 6", "R-Plot 7", "R-Plot 8", "R-Plot 9": Mouse Move {
        # "Process mouse movement over plots in special modes (\"Cursor\", \"Erase\")"
        n736 = event-data() -> ("CtlRef"=w1125:refnum<vi>, "Coords"=w1126:T69)  [unwired: 1 in, 3 out]
        n737 = property on="Mode Buttons" class="RadioBtnsControl (strict)"() -> ("Value"=w1129:T7)  [unwired: 2 in, 2 out]
        n738 = local read "_LMBDown"() -> (w1130:bool)
        n739 = Equal?(x=w1129, y=Cursor_Controls."Erase range" ("Mode Buttons")) -> (x = y?=w1127:bool)
        n740 = And(x=w1130, y=w1127) -> (x .and. y?=w1128:bool)
        n741 = case shown="True" w1128 {
          tunnel: w1126 -> [_ w1132]
          tunnel: w1125 -> [_ w1131]
          frame False {
          }
          frame True {
            n742 = invoke class="XYGraph (strict)" method="Map Coords To XY"(reference=w1131, "Coords"=w1132) -> (reference out=w1135:refnum<vi>, "XY"=w1134:cluster{"X":dbl, "Y":dbl})  [unwired: 5 in, 5 out]
            n743 = property class="XYGraph (strict)"(reference=w1135, "Active Cursor"=u32 1, "Cursor.Cursor Position"=w1134) -> ()  [unwired: 1 in, 2 out]
          }
        }
      }
      event "R-Plot 0", "R-Plot 1", "R-Plot 2", "R-Plot 3", "R-Plot 4", "R-Plot 5", "R-Plot 6", "R-Plot 7", "R-Plot 8", "R-Plot 9": Mouse Up {
        n744 = event-data() -> ("CtlRef"=w1139:refnum<vi>, "Button"=w1137:u16)  [unwired: 1 in, 6 out]
        n745 = property on="Mode Buttons" class="RadioBtnsControl (strict)"() -> ("Value"=w1140:T7)  [unwired: 2 in, 2 out]
        n746 = property class="XYGraph (strict)"(reference=w1139) -> ("ActPaletteTool"=w1138:i32)  [unwired: 1 in, 2 out]
        n747 = case shown="1" w1137 {
          tunnel: w1140 -> [_ w1144]
          tunnel: w1139 -> [_ w1143]
          tunnel: w1138 -> [_ w1142]
          frame Default {
          }
          frame 1 {
            n748 = local read "_LMBDown"() -> (w1141:bool)
            n749 = case shown="0" w1142 {
              tunnel: w1144 -> [_ w1149]
              tunnel: w1143 -> [_ w1148]
              tunnel: w1141 -> [_ w1146]
              frame Default {
                n750 = property on="Mode Buttons" class="RadioBtnsControl (strict)"("Val(Sgnl)"=T54."No Selection" ("Value (Signaling)")) -> ()  [unwired: 2 in, 2 out]
              }
              frame 0 {
                n751 = Equal?(x=w1149, y=T54."Erase range") -> (x = y?=w1152:bool)
                n752 = And(x=w1146, y=w1152) -> (x .and. y?=w1151:bool)
                n753 = case shown="True" w1151 {
                  tunnel: w1148 -> [_ w1175]
                  frame False {
                  }
                  frame True {
                    n754 = local read "Channels Panel"() -> (w1174:T8)
                    n755 = property class="XYGraph (strict)"(reference=w1175, "Active Cursor"=u32 0, "Active Cursor"=u32 1) -> ("Cursor.Cursor X"=w1172:dbl, "Cursor.Cursor X"=w1153:dbl)  [unwired: 1 in, 2 out]
                    n756 = local read "Data Array"() -> (w1169:T28)
                    n757 = Max & Min(x=w1172, y=w1153) -> (max(x,y)=w1162:dbl, min(x,y)=w1155:dbl)
                    n758 = Index Array(array=w1169, index=w1174) -> (element=w1165:cluster{"R":dbl[], "T":dbl[], "Time":dbl[]})
                    n759 = Unbundle By Name(w1165) -> ("R"=w1163:dbl[], "T"=w1164:dbl[], "Time"=w1161:dbl[])
                    n760 = Threshold 1D Array(2:w1162, 3:w1161) -> (0:w1159:dbl)  [unwired: 1 in]
                    n761 = Threshold 1D Array(2:w1155, 3:w1161) -> (0:w1160:dbl)  [unwired: 1 in]
                    n762 = Subtract(x=w1159, y=w1160) -> (x-y=w1158:dbl)
                    n763 = Delete From Array(array=w1163, length=w1158, index=w1160) -> (array with subset deleted=w1168:dbl[])  [unwired: 1 out]
                    n764 = Delete From Array(array=w1164, length=w1158, index=w1160) -> (array with subset deleted=w1167:dbl[])  [unwired: 1 out]
                    n765 = Delete From Array(array=w1161, length=w1158, index=w1160) -> (array with subset deleted=w1166:dbl[])  [unwired: 1 out]
                    n766 = Bundle By Name(cluster=w1165, "R"=w1168, "T"=w1167, "Time"=w1166) -> (w1170:cluster{"R":dbl[], "T":dbl[], "Time":dbl[]})
                    n767 = Replace Array Subset(array=w1169, new element=w1170, index=w1174) -> (w1171:T28)
                    n768 = local write "Data Array"(w1171) -> ()
                    n769 = property class="XYGraph (strict)"(reference=w1175, "Active Cursor"=u32 0, "Cursor.Cursor X"=w1155, "Active Cursor"=u32 1, "Cursor.Cursor X"=w1155) -> ()  [unwired: 1 in, 2 out]
                  }
                }
                n770 = local write "_LMBDown"(FALSE ("Mouse down")) -> ()
              }
            }
          }
        }
      }
      event "R-Plot 0", "R-Plot 1", "R-Plot 2", "R-Plot 3", "R-Plot 4", "R-Plot 5", "R-Plot 6", "R-Plot 7", "R-Plot 8", "R-Plot 9": Mouse Leave {
        n771 = event-data() -> ()  [unwired: 1 in, 4 out]
        n772 = local write "_LMBDown"(FALSE ("Mouse down")) -> ()
      }
      event "R-Plot 0", "R-Plot 1", "R-Plot 2", "R-Plot 3", "R-Plot 4", "R-Plot 5", "R-Plot 6", "R-Plot 7", "R-Plot 8", "R-Plot 9": Scale Range Change {
        w1180 = u8 0 ("X Scale.Scale Fit")
        # "Disable plot autoscaling if the user has changed the scale of the plot manualy"
        n773 = event-data() -> ("CtlRef"=w1179:refnum<vi>)  [unwired: 1 in, 7 out]
        n774 = property class="XYGraph (strict)"(reference=w1179, "XScale.ScaleFit"=w1180, "YScale.ScaleFit"=w1180) -> ()  [unwired: 1 in, 2 out]
      }
      event "R-Plot 0", "R-Plot 1", "R-Plot 2", "R-Plot 3", "R-Plot 4", "R-Plot 5", "R-Plot 6", "R-Plot 7", "R-Plot 8", "R-Plot 9": Shortcut Menu Activation? {
        w1189 = string[] ["Log Y"] ("item names")
        w1191 = string[] ["Zoom In to Last Data", "Autoscale XY"] ("item names")
        # "Add extra options to the plots context menu"
        n775 = event-data() -> ("MenuRef"=w1193:refnum<k9>, "CtlRef"=w1185:refnum<vi>)  [unwired: 1 in]
        n776 = Insert Menu Items(4:10, 7:w1191, 8:w1191, 9:w1193) -> (3:w1187:refnum<k9>)  [unwired: 2 in, 2 out]
        n777 = property class="XYGraph (strict)"(reference=w1185) -> ("YScale.Mapping Mode"=w1184:u8)  [unwired: 1 in, 2 out]
        n778 = Insert Menu Items(4:14, 7:w1189, 8:w1189, 9:w1187) -> (3:w1186:refnum<k9>)  [unwired: 2 in, 2 out]
        n779 = Not Equal To 0?(x=w1184) -> (x != 0?=w1183:bool)
        n780 = Set Menu Item Info(6:w1183, 7:"Log Y", 11:w1186) -> ()  [unwired: 4 in, 2 out]
        n781 = local read "_LMBDown"() -> (w1190:bool)
        n782 = event-data("Discard?"=w1190) -> ()  [unwired: 1 in, 1 out]
      }
      event "R-Plot 0", "R-Plot 1", "R-Plot 2", "R-Plot 3", "R-Plot 4", "R-Plot 5", "R-Plot 6", "R-Plot 7", "R-Plot 8", "R-Plot 9": Shortcut Menu Selection (User) {
        # "Zoom in to last \"Miniplot points\". Zoom out a bit to have some space around the points"
        n783 = event-data() -> ("CtlRef"=w1199:refnum<vi>, "ItemTag"=w1197:string)  [unwired: 1 in]
        n784 = Type Cast(type=refnum<vi> refnum ("R-Plot 0"), x=w1199) -> (*(type *) &x=w1198:refnum<vi>)
        n785 = property on="Runtime Settings" class="Clust (strict)"() -> ("Value"=w1195:T27)  [unwired: 2 in, 2 out]
        n786 = case shown="\"Zoom In to Last Data\"" w1197 {
          tunnel: w1198 -> [_ w1201 w1230 w1236]
          tunnel: w1195 -> [_ _ w1202 _]
          frame Default {
          }
          frame "Autoscale XY" {
            w1200 = u8 2 ("X Scale.Scale Fit")
            n787 = property class="XYGraph (strict)"(reference=w1201, "XScale.ScaleFit"=w1200, "YScale.ScaleFit"=w1200) -> ()  [unwired: 1 in, 2 out]
          }
          frame "Zoom In to Last Data" {
            w1226 = u8 0 ("Y Scale.Scale Fit")
            n788 = property class="XYGraph (strict)"(reference=w1230) -> (reference out=w1227:refnum<vi>, "Value"=w1229:cluster{dbl[], dbl[]})  [unwired: 1 in, 1 out]
            n789 = Unbundle By Name(w1202) -> ("Miniplot Time"=w1225:dbl)
            n790 = Unbundle(w1229) -> (w1204:dbl[], w1228:dbl[])
            n791 = Multiply(x=w1225, y=60.0) -> (x*y=w1221:dbl)
            n792 = Reverse 1D Array(array=w1204) -> (reversed array=w1209:dbl[])
            n793 = Reverse 1D Array(array=w1228) -> (reversed array=w1217:dbl[])
            n794 = Index Array(array=w1209) -> (element=w1223:dbl)  [unwired: 1 in]
            n795 = Multiply(x=0.5, y=w1221) -> (x*y=w1222:dbl)
            n796 = Add(x=w1222, y=w1223) -> (x+y=w1220:dbl)
            n797 = Subtract(x=w1223, y=w1221) -> (x-y=w1218:dbl)
            n798 = call "Improved Threshold Detector.71.vi"("Threshold"=w1218, "Array"=w1204) -> ("Positive transition indices"=w1205:i32[])  [unwired: 8 in, 1 out]
            n799 = Index Array(array=w1205) -> (element=w1231:i32)  [unwired: 1 in]
            n800 = Array Size(array=w1204) -> (size(s)=w1207:i32)
            n801 = Index Array(array=w1204, index=w1231) -> (element=w1203:dbl)
            n802 = Subtract(x=w1207, y=w1231) -> (x-y=w1206:i32)
            n803 = Array Subset(array=w1217, length=w1206) -> (w1216:dbl[])  [unwired: 1 in]
            n804 = Array Max & Min(array=w1216) -> (max value=w1213:dbl, min value=w1212:dbl)  [unwired: 2 out]
            n805 = Subtract(x=w1213, y=w1212) -> (x-y=w1215:dbl)
            n806 = Divide(x=w1215, y=2.0) -> (x/y=w1211:dbl)
            n807 = Add(x=w1213, y=w1211) -> (x+y=w1208:dbl)
            n808 = Subtract(x=w1212, y=w1211) -> (x-y=w1210:dbl)
            n809 = property class="XYGraph (strict)"(reference=w1227, "XScale.ScaleFit"=w1226, "YScale.ScaleFit"=w1226, "XScale.Maximum"=w1220, "XScale.Minimum"=w1203, "YScale.Maximum"=w1208, "YScale.Minimum"=w1210) -> ()  [unwired: 1 in, 2 out]
          }
          frame "Log Y" {
            n810 = property class="XYGraph (strict)"(reference=w1236) -> (reference out=w1235:refnum<vi>, "YScale.Mapping Mode"=w1234:u8)  [unwired: 1 in, 1 out]
            n811 = Equal To 0?(x=w1234) -> (x = 0?=w1233:bool)
            n812 = Boolean To (0,1)(Boolean=w1233) -> (0, 1=w1232:i16)
            n813 = property class="XYGraph (strict)"(reference=w1235, "YScale.Mapping Mode"=w1232) -> ()  [unwired: 1 in, 2 out]
          }
        }
      }
      event "uPlots.uPlot 0", "uPlots.uPlot 1", "uPlots.uPlot 2", "uPlots.uPlot 3", "uPlots.uPlot 4", "uPlots.uPlot 5", "uPlots.uPlot 6", "uPlots.uPlot 7", "uPlots.uPlot 8", "uPlots.uPlot 9": Mouse Down {
        # "Switch to big plot on double click on small plot"
        n814 = event-data() -> ("Mods.Double Click"=w1239:bool, "CtlRef"=w1238:refnum<vi>)  [unwired: 1 in]
        n815 = case shown="True" w1239 {
          tunnel: w1238 -> [_ w1242]
          frame False {
          }
          frame True {
            n816 = property class="XYGraph (strict)"(reference=w1242) -> ("Label.Text"=w1243:string)  [unwired: 1 in, 2 out]
            n817 = Reverse String(1:w1243) -> (0:w1244:string)
            n818 = Decimal String To Number(string=w1244, default (0L)=8 ("default (0 I32)")) -> (number=w1241:i32)  [unwired: 1 in, 1 out]
            n819 = property on="Channels Panel" class="TabCtl (strict)"("Val(Sgnl)"=w1241) -> ()  [unwired: 2 in, 2 out]
          }
        }
      }
      event "Erase all": Value Change {
        # "Clear data array.\nReset PID."
        n820 = event-data() -> ()  [unwired: 1 in, 6 out]
        n821 = local read "Channels Panel"() -> (w1248:T8)
        n822 = local read "Data Array"() -> (w1249:T28)
        n823 = Replace Array Subset(array=w1249, new element=cluster{"R":dbl[], "T":dbl[], "Time":dbl[]} {"R"=[], "T"=[], "Time"=[]} ("new element/subarray"), index=w1248) -> (w1247:T28)
        n824 = local write "Data Array"(w1247) -> ()
        n825 = disable-structure shown="Disabled" {
          frame Disabled {
            n826 = Initialize Array(cluster{"R":dbl[], "T":dbl[], "Time":dbl[]} {"R"=[], "T"=[], "Time"=[]}, 10 ("dimension size")) -> ()  [unwired: 1 out]
          }
          frame Enabled {
          }
        }
      }
      event "Clear all plots": Value Change {
        n827 = event-data() -> ()  [unwired: 1 in, 6 out]
        n828 = Initialize Array(cluster{"R":dbl[], "T":dbl[], "Time":dbl[]} {"R"=[], "T"=[], "Time"=[]}, 10 ("dimension size")) -> (w1254:cluster{"R":dbl[], "T":dbl[], "Time":dbl[]}[])
        n829 = local write "Data Array"(w1254) -> ()
      }
      event "Bridge settings.Bridge Type": Value Change {
        # "Select bridge type (AVS/zBridge). Show/hide corresponding controls."
        n830 = event-data() -> ("NewVal"=w1258:T60)  [unwired: 1 in, 5 out]
        n831 = flat-sequence {
          tunnel: w1258 -> [w1267]
          frame #0 {
            w1263 = u8 0 ("Disabled")
            w1266 = u8 0 ("Disabled")
            w1265 = FALSE ("Visible")
            w1264 = u8 2 ("Disabled")
            n832 = property on="AVS RS232 Port" class="VISAName"("Visible"=w1265, "Disabled"=w1264) -> ()  [unwired: 2 in, 2 out]
            n833 = property on="zBridge settings" class="Bool"("Visible"=w1265, "Disabled"=w1264) -> ()  [unwired: 2 in, 2 out]
            n834 = property on="Lower Panel" class="TabCtl (strict)"("Disabled"=w1263) -> ()  [unwired: 2 in, 2 out]
            n835 = property on="AVS GPIB Address" class="VISAName"("Visible"=w1265, "Disabled"=w1264) -> ()  [unwired: 2 in, 2 out]
            n836 = property on="Main Panel" class="TabCtl (strict)"("Disabled"=w1263) -> ()  [unwired: 2 in, 2 out]
            n837 = property on="Read AVS channels from" class="DigNum (strict)"("Disabled"=w1266) -> ()  [unwired: 2 in, 2 out]
            n838 = property on="Last Channel" class="DigNum (strict)"("Disabled"=w1266) -> ()  [unwired: 2 in, 2 out]
            n839 = property on="Stabilisation Delay" class="DigNum (strict)"("Disabled"=w1266) -> ()  [unwired: 2 in, 2 out]
            n840 = property on="Averages" class="DigNum (strict)"("Disabled"=w1266) -> ()  [unwired: 2 in, 2 out]
            n841 = property on="Delay Between Scans" class="DigNum (strict)"("Disabled"=w1266) -> ()  [unwired: 2 in, 2 out]
            n842 = call "Build ranges list.vi"("Values"="-1\r\n0\r\n1\r\n2\r\n3\r\n4\r\n5\r\n6\r\n7", "Strings"="n.a.\r\nopen\r\n2 Ohm\r\n20 Ohm\r\n200 Ohm\r\n2k Ohm\r\n20k Ohm\r\n200k Ohm\r\n2M Ohm") -> ("Strings and Values"=w1262:cluster{"String":string, "Value":i32}[])  [unwired: 4 in]
            n843 = property on="Range 0" class="Ring (strict)"("StringsAndValues[]"=w1262) -> ()  [unwired: 2 in, 2 out]
            n844 = property on="Range 1" class="Ring (strict)"("StringsAndValues[]"=w1262) -> ()  [unwired: 2 in, 2 out]
            n845 = property on="Range 2" class="Ring (strict)"("StringsAndValues[]"=w1262) -> ()  [unwired: 2 in, 2 out]
            n846 = property on="Range 3" class="Ring (strict)"("StringsAndValues[]"=w1262) -> ()  [unwired: 2 in, 2 out]
            n847 = property on="Range 4" class="Ring (strict)"("StringsAndValues[]"=w1262) -> ()  [unwired: 2 in, 2 out]
            n848 = property on="Range 5" class="Ring (strict)"("StringsAndValues[]"=w1262) -> ()  [unwired: 2 in, 2 out]
            n849 = property on="Range 6" class="Ring (strict)"("StringsAndValues[]"=w1262) -> ()  [unwired: 2 in, 2 out]
            n850 = property on="Range 7" class="Ring (strict)"("StringsAndValues[]"=w1262) -> ()  [unwired: 2 in, 2 out]
          }
          frame #1 {
            n851 = case shown="\"AVS48SI (RS232 interface)\"" w1267 {
              frame "AVS47A (GPIB interface)" {
                n852 = local write "AVS Scan Parameters"(enum32{"Page 1", "Page 2"}."Page 1" ("Scan Parameters")) -> ()
                n853 = property on="AVS GPIB Address" class="VISAName"("Visible"=TRUE, "Disabled"=u8 0) -> ()  [unwired: 2 in, 2 out]
              }
              frame "AVS47B (RS232 interface)" {
                w1271 = u8 2 ("Disabled")
                n854 = local write "AVS Scan Parameters"(enum32{"Page 1", "Page 2"}."Page 1" ("Scan Parameters")) -> ()
                n855 = property on="AVS RS232 Port" class="VISAName"("Visible"=TRUE, "Disabled"=u8 0) -> ()  [unwired: 2 in, 2 out]
                n856 = property on="Read AVS channels from" class="DigNum (strict)"("Disabled"=w1271) -> ()  [unwired: 2 in, 2 out]
                n857 = property on="Last Channel" class="DigNum (strict)"("Disabled"=w1271) -> ()  [unwired: 2 in, 2 out]
              }
              frame "AVS48SI (RS232 interface)" {
                w1278 = u8 2 ("Disabled")
                n858 = property on="Read AVS channels from" class="DigNum (strict)"("Disabled"=w1278) -> ()  [unwired: 2 in, 2 out]
                n859 = property on="Last Channel" class="DigNum (strict)"("Disabled"=w1278) -> ()  [unwired: 2 in, 2 out]
                n860 = property on="AVS RS232 Port" class="VISAName"("Visible"=TRUE, "Disabled"=u8 0) -> ()  [unwired: 2 in, 2 out]
                n861 = local write "AVS Scan Parameters"(enum32{"Page 1", "Page 2"}."Page 1" ("Scan Parameters")) -> ()
                n862 = call "Build ranges list.vi"("Values"="-1\r\n0\r\n1\r\n2\r\n3\r\n4\r\n5\r\n6\r\n7", "Strings"="n.a.\r\n3 Ohm\r\n30 Ohm\r\n300 Ohm\r\n3k Ohm\r\n30k Ohm\r\n300k Ohm\r\n3M Ohm\r\n30m Ohm") -> ("Strings and Values"=w1276:cluster{"String":string, "Value":i32}[])  [unwired: 4 in]
                n863 = property on="Range 0" class="Ring (strict)"("StringsAndValues[]"=w1276) -> ()  [unwired: 2 in, 2 out]
                n864 = property on="Range 1" class="Ring (strict)"("StringsAndValues[]"=w1276) -> ()  [unwired: 2 in, 2 out]
                n865 = property on="Range 2" class="Ring (strict)"("StringsAndValues[]"=w1276) -> ()  [unwired: 2 in, 2 out]
                n866 = property on="Range 3" class="Ring (strict)"("StringsAndValues[]"=w1276) -> ()  [unwired: 2 in, 2 out]
                n867 = property on="Range 4" class="Ring (strict)"("StringsAndValues[]"=w1276) -> ()  [unwired: 2 in, 2 out]
                n868 = property on="Range 5" class="Ring (strict)"("StringsAndValues[]"=w1276) -> ()  [unwired: 2 in, 2 out]
                n869 = property on="Range 6" class="Ring (strict)"("StringsAndValues[]"=w1276) -> ()  [unwired: 2 in, 2 out]
                n870 = property on="Range 7" class="Ring (strict)"("StringsAndValues[]"=w1276) -> ()  [unwired: 2 in, 2 out]
              }
              frame "AVS Emulation" {
                n871 = local write "AVS Scan Parameters"(enum32{"Page 1", "Page 2"}."Page 1" ("Scan Parameters")) -> ()
              }
              frame "Impedance Bridge" {
                w1285 = u8 2 ("Disabled")
                n872 = local write "AVS Scan Parameters"(enum32{"Page 1", "Page 2"}."Page 2" ("Scan Parameters")) -> ()
                n873 = property on="zBridge settings" class="Bool"("Visible"=TRUE, "Disabled"=u8 0) -> ()  [unwired: 2 in, 2 out]
                n874 = property on="Read AVS channels from" class="DigNum (strict)"("Disabled"=w1285) -> ()  [unwired: 2 in, 2 out]
                n875 = property on="Last Channel" class="DigNum (strict)"("Disabled"=w1285) -> ()  [unwired: 2 in, 2 out]
                n876 = property on="Stabilisation Delay" class="DigNum (strict)"("Disabled"=w1285) -> ()  [unwired: 2 in, 2 out]
                n877 = property on="Averages" class="DigNum (strict)"("Disabled"=w1285) -> ()  [unwired: 2 in, 2 out]
                n878 = property on="Delay Between Scans" class="DigNum (strict)"("Disabled"=w1285) -> ()  [unwired: 2 in, 2 out]
              }
              frame "Disabled", Default {
                w1287 = u8 2 ("Disabled")
                n879 = property on="Lower Panel" class="TabCtl (strict)"("Disabled"=w1287) -> ()  [unwired: 2 in, 2 out]
                n880 = property on="Main Panel" class="TabCtl (strict)"("Disabled"=w1287) -> ()  [unwired: 2 in, 2 out]
              }
            }
          }
        }
      }
      event "Runtime Settings.Plot type": Value Change {
        # "Iterate through first 10 pages (plots only)"
        # "Switch between RxTime and TxTime plots"
        n881 = event-data() -> ("NewVal"=w1298:enum16{"R vs Time", "T vs Time"})  [unwired: 1 in, 5 out]
        n882 = Unbundle By Name(w1290) -> ("Reset PID loop"=w1289:refnum<user-event>)
        n883 = Equal To 0?(x=w1298) -> (x = 0?=w1297:bool)
        n884 = Select(t=u32 10532351, s=w1297, f=u32 16711680) -> (s? t:f=w1294:u32)
        n885 = property on="uPlots" class="Clust (strict)"() -> ("Controls[]"=w1292:refnum<vi>[])  [unwired: 2 in, 2 out]
        n886 = property on="Channels Panel" class="TabCtl (strict)"() -> ("Pages"=w1299:refnum<vi>[])  [unwired: 2 in, 2 out]
        n887 = for {
          N: 10 -> [_]
          tunnel: w1299 -> [w1309] mode=indexing
          tunnel: w1294 -> [w1302]
          tunnel: w1292 -> [w1300] mode=indexing
          # "!!NOTE:This routine assumes that graph is control #0 on page!!"
          n888 = property class="Page"(reference=w1309) -> ("ControlsOnPage"=w1307:refnum<vi>[])  [unwired: 1 in, 2 out]
          n889 = Type Cast(type=refnum<vi> refnum ("R-Plot 0"), x=w1300) -> (*(type *) &x=w1301:refnum<vi>)
          n890 = Index Array(array=w1307, index=0) -> (element=w1305:refnum<vi>)
          n891 = Type Cast(type=refnum<vi> refnum ("R-Plot 0"), x=w1305) -> (*(type *) &x=w1304:refnum<vi>)
          n892 = property class="XYGraph (strict)"(reference=w1304, "Plot.Plot Color"=w1302, "Plot.Fill/Pt. Color"=w1302) -> ()  [unwired: 1 in, 2 out]
          n893 = property class="XYGraph (strict)"(reference=w1301, "Plot.Plot Color"=w1302, "Plot.Fill/Pt. Color"=w1302) -> ()  [unwired: 1 in, 2 out]
        }
        n894 = Generate User Event(user event=w1289, event data cluster="" ("event data")) -> ()  [unwired: 2 in, 2 out]
      }
      event "Runtime Settings.Read AVS channels from", "Runtime Settings.Last Channel": Value Change {
        # "Change enabled channels for the AVS bridge"
        n895 = event-data() -> ()  [unwired: 1 in, 6 out]
        n896 = Unbundle By Name(w1312) -> ("UpdateChannelInfo"=w1311:refnum<user-event>)
        n897 = Generate User Event(user event=w1311, event data cluster=bool[] [] ("event data")) -> ()  [unwired: 2 in, 2 out]
      }
      event "Runtime Settings.Filter Graphs": Value Change {
        # "Graph filtering controls"
        n898 = event-data() -> ("NewVal"=w1315:bool)  [unwired: 1 in, 5 out]
        n899 = call "IsDisabled.vi"("Enabled?"=w1315) -> ("Numeric"=w1316:i16)
        n900 = property on="Y_min" class="DigNum (strict)"("Disabled"=w1316) -> ()  [unwired: 2 in, 2 out]
        n901 = property on="Y_max" class="DigNum (strict)"("Disabled"=w1316) -> ()  [unwired: 2 in, 2 out]
      }
      event "Channels Panel": Value Change {
        # "Show hide bottom Impedance/Temperature panel depending on the current tab page"
        n902 = event-data() -> ("NewVal"=w1319:T8)  [unwired: 1 in, 5 out]
        n903 = case shown="Default" w1319 {
          tunnel: [TRUE ("Visible") FALSE ("Visible")] -> w1318
          frame Default {
            n904 = property on="Mode Buttons" class="RadioBtnsControl (strict)"() -> ("Value"=w1321:T7)  [unwired: 2 in, 2 out]
            n905 = property on="Data History/RT Settings" class="TabCtl (strict)"("Value"=enum32{"History", "Settings"}."History" ("Data History")) -> ()  [unwired: 2 in, 2 out]
            n906 = property on="Mode Buttons" class="RadioBtnsControl (strict)"("Val(Sgnl)"=w1321) -> ()  [unwired: 2 in, 2 out]
          }
          frame "All", "PID loop" {
            n907 = property on="Data History/RT Settings" class="TabCtl (strict)"("Value"=enum32{"History", "Settings"}."Settings" ("Data History")) -> ()  [unwired: 2 in, 2 out]
          }
        }
        n908 = property on="Graph Controls Bar" class="TabCtl (strict)"("Visible"=w1318) -> ()  [unwired: 2 in, 2 out]
      }
      event Value Change {
        # "Calibration changed - update calibrations list"
        n909 = event-data() -> ()  [unwired: 1 in, 6 out]
        n910 = property on="Sensor Calibrations" class="Clust (strict)"() -> ("Controls[]"=w1328:refnum<vi>[])  [unwired: 2 in, 2 out]
        n911 = Array Size(array=w1328) -> (size(s)=w1329:i32)
        n912 = for {
          N: w1329 -> [_]
          tunnel: w1328 -> [w1333] mode=indexing
          tunnel: [w1330] -> w1327 mode=indexing
          w1332 = refnum<vi> refnum  # Ring
          n913 = Type Cast(type=w1332, x=w1333) -> (*(type *) &x=w1331:refnum<vi>)
          n914 = property class="Ring"(reference=w1331) -> ("RingText.Text"=w1330:string)  [unwired: 1 in, 2 out]
        }
        n915 = Array To Cluster(array=w1327) -> (cluster=→"_CurCalibrations":T33)
      }
      event "Data Logging Settings": Value Change {
        # "Log file settings changed. Generate new log file name"
        n916 = event-data() -> ()  [unwired: 1 in, 3 out]
        n917 = local read "Data Logging Settings"() -> (w1342:T37)
        n918 = Unbundle By Name(w1342) -> ("Run Description"=w1336:string, "Filenames Suffix"=w1337:string, "Log Files Folder"=w1343:path, "Log Files Name"=w1341:string, "Automode Files Name"=w1340:string)
        n919 = call <userlib>:"MGI Make String Filesafe.vi"("String In"=w1336) -> ("Filesafe String Out"=w1335:string)
        n920 = call "GeneratePaths.vi"("Filename Suffix"=w1337, "Run description"=w1335, "AVS_Path"=w1343, "AVS_FName"=w1341, "CAL_Path"=w1343, "CAL_FName"=w1340) -> ("Generated Log path"=w1339:path, "Generated Calib path"=w1338:path)  [unwired: 8 in]
        n921 = local write "_LogFilesPath"(w1339) -> ()
        n922 = local write "_CalibFilesPath"(w1338) -> ()
      }
      event "Convert R-T": Mouse Down; "QuickR": Value Change {
        # "Quick convert R->T"
        n923 = event-data() -> ()  [unwired: 1 in, 4 out]
        n924 = Unbundle By Name(w1344) -> ("Calibrations Folder"=w1345:path)
        n925 = property on="_QuickConvertCal" class="Ring (strict)"() -> ("Strings []"=w1348:string[], "Value"=w1349:u16)  [unwired: 2 in, 2 out]
        n926 = Index Array(array=w1348, index=w1349) -> (element=w1347:string)
        n927 = call "SelectSensor-txt no ext.vi"("Path"=w1345, "Resistance"="QuickR", "Select sensor"=w1347) -> ("error out"=w1346:errorcluster, "Temperature"=→"T7":dbl)
      }
      event "T Sweep.Current": Value Change {
        # "Current/ Setpoint value is changed"
        n928 = event-data() -> ("NewVal"=→"_I3SetPnt":dbl)  [unwired: 1 in, 5 out]
        n929 = Unbundle By Name(w1354) -> ("Reset PID loop"=w1353:refnum<user-event>)
        n930 = Generate User Event(user event=w1353, event data cluster="" ("event data")) -> ()  [unwired: 2 in, 2 out]
      }
      event Value Change {
        w1358 = FALSE ("Value (Signaling)")
        # "Changed Channel1 automatic mode"
        n931 = event-data() -> ("NewVal"=w1360:T39)  [unwired: 1 in, 5 out]
        n932 = Unbundle By Name(w1362) -> ("TempStabilized"=w1361:refnum<user-event>)
        n933 = property on="CS.Mode1.Start" class="Bool (strict)"("Val(Sgnl)"=w1358) -> ()  [unwired: 2 in, 2 out]
        n934 = property on="CS.Mode2.Start" class="Bool (strict)"("Val(Sgnl)"=w1358) -> ()  [unwired: 2 in, 2 out]
        n935 = case shown="\"Mode 1\"" w1360 {
          tunnel: [FALSE ("Automatic mode ON") TRUE ("Automatic mode ON") TRUE ("Automatic mode ON")] -> w1363
          tunnel: w1361 -> [_ w1373 _]
          tunnel: [0 1 2] -> w1359
          frame "Manual" {
            # "Set manual mode currents \nequal to last automode \nvalues."
            n936 = local read "CS.Automode Current"() -> (w1366:T23[])
            n937 = Index Array(array=w1366) -> (element #1=w1370:T23, element #2=w1369:T23, element #3=w1368:T23, element #4=w1367:T23)  [unwired: 4 in]
            n938 = property on="I" class="DigNum (strict)"("Val(Sgnl)"=w1370) -> ()  [unwired: 2 in, 2 out]
            n939 = property on="I" class="DigNum (strict)"("Val(Sgnl)"=w1369) -> ()  [unwired: 2 in, 2 out]
            n940 = property on="I" class="DigNum (strict)"("Val(Sgnl)"=w1368) -> ()  [unwired: 2 in, 2 out]
            n941 = property on="I" class="DigNum (strict)"("Val(Sgnl)"=w1367) -> ()  [unwired: 2 in, 2 out]
          }
          frame "Mode 1" {
            # "Set automatic mode currents equal to last manual values."
            n942 = local read "CS.Current Value"() -> (w1376:dbl[])
            n943 = Multiply(x=1000.0, y=w1376) -> (x*y=w1374:dbl[])
            n944 = local write "CS.Automode Current"(w1374) -> ()
            n945 = Generate User Event(user event=w1373, event data cluster=FALSE ("event data")) -> ()  [unwired: 2 in, 2 out]
          }
          frame "Mode2" {
            # "Set automatic mode currents equal to last manual values."
            n946 = local read "CS.Current Value"() -> (w1381:dbl[])
            n947 = Multiply(x=1000.0, y=w1381) -> (x*y=w1379:dbl[])
            n948 = local write "CS.Automode Current"(w1379) -> ()
          }
        }
        "CS.Automode 1" <- w1363
        "CS.Automode 2" <- w1363
        "CS.Automode 3" <- w1363
        "CS.Automode 0" <- w1363
        n949 = property on="CS Modes Panel" class="TabCtl (strict)"("Value"=w1359) -> ()  [unwired: 2 in, 2 out]
      }
      event "Data Logging Settings.External VI Path": Value Change {
        # "Set path for the external VI to call on TempStabilised event"
        n950 = event-data() -> ("NewVal"=w1386:path)  [unwired: 1 in, 5 out]
        n951 = vi-ref "OnTempStabilizedRef.vi"() -> (w1387:refnum<vi>)
        n952 = Open VI Reference(type specifier VI Refnum (for type only)=w1387, vi path=w1386) -> (vi reference=w1385:refnum<vi>)  [unwired: 4 in, 1 out]
        n953 = local write "_ExtVIReference"(w1385) -> ()
      }
      event "CS Settings.CS type": Value Change {
        # "Set CS type"
        n954 = event-data() -> ("NewVal"=w1389:T56)  [unwired: 1 in, 5 out]
        n955 = flat-sequence {
          tunnel: w1389 -> [w1416]
          frame #0 {
            w1401 = u8 2 ("Disabled")
            w1396 = u8 0 ("Disabled")
            w1411 = TRUE ("Visible")
            n956 = control-ref of="CS Indicators Panel"() -> (w1397:refnum<vi>)
            n957 = control-ref of="I0"() -> (w1408:refnum<vi>)
            n958 = control-ref of="I1"() -> (w1400:refnum<vi>)
            n959 = control-ref of="CS.I0"() -> (w1407:refnum<vi>)
            n960 = control-ref of="CS.I1"() -> (w1399:refnum<vi>)
            n961 = control-ref of="I2"() -> (w1395:refnum<vi>)
            n962 = control-ref of="I3"() -> (w1394:refnum<vi>)
            n963 = control-ref of="CS Mode"() -> (w1398:refnum<vi>)
            n964 = control-ref of="QCS. I0 Mapping"() -> (w1406:refnum<vi>)
            n965 = property class="TabCtl (strict)"(reference=w1397, "Disabled"=w1396) -> ()  [unwired: 1 in, 2 out]
            n966 = property class="Clust (strict)"(reference=w1408, "Disabled"=w1396) -> ()  [unwired: 1 in, 2 out]
            n967 = property class="Clust (strict)"(reference=w1400, "Disabled"=w1396) -> ()  [unwired: 1 in, 2 out]
            n968 = property class="Clust (strict)"(reference=w1395, "Disabled"=w1396) -> ()  [unwired: 1 in, 2 out]
            n969 = property class="Clust (strict)"(reference=w1394, "Disabled"=w1396) -> ()  [unwired: 1 in, 2 out]
            n970 = property class="Clust (strict)"(reference=w1407, "Disabled"=w1396) -> ()  [unwired: 1 in, 2 out]
            n971 = property class="Clust (strict)"(reference=w1399, "Disabled"=w1396) -> ()  [unwired: 1 in, 2 out]
            n972 = property class="Enum (strict)"(reference=w1406, "Disabled"=w1396) -> ()  [unwired: 1 in, 2 out]
            n973 = property class="Enum (strict)"(reference=w1398, "Disabled"=w1396) -> ()  [unwired: 1 in, 2 out]
            n974 = property on="Side Panel" class="TabCtl (strict)"() -> ("Pages"=w1390:refnum<vi>[])  [unwired: 2 in, 2 out]
            n975 = control-ref of="TCS RS232 Port"() -> (w1410:refnum<vi>)
            n976 = Index Array(array=w1390, index=1) -> (element=w1391:refnum<vi>)
            n977 = control-ref of="Toggle Gated"() -> (w1402:refnum<vi>)
            n978 = control-ref of="Toggle Gated"() -> (w1403:refnum<vi>)
            n979 = control-ref of="Toggle Gated"() -> (w1404:refnum<vi>)
            n980 = control-ref of="Toggle Gated"() -> (w1405:refnum<vi>)
            n981 = control-ref of="CS.QCS Device Nr"() -> (w1413:refnum<vi>)
            n982 = control-ref of="CS.QCS I0 Output"() -> (w1412:refnum<vi>)
            n983 = property class="Page"(reference=w1391, "PageVis"=TRUE ("Page Visible")) -> ()  [unwired: 1 in, 2 out]
            n984 = property class="Bool (strict)"(reference=w1402, "Disabled"=w1401) -> ()  [unwired: 1 in, 2 out]
            n985 = property class="Bool (strict)"(reference=w1403, "Disabled"=w1401) -> ()  [unwired: 1 in, 2 out]
            n986 = property class="Bool (strict)"(reference=w1404, "Disabled"=w1401) -> ()  [unwired: 1 in, 2 out]
            n987 = property class="Bool (strict)"(reference=w1405, "Disabled"=w1401) -> ()  [unwired: 1 in, 2 out]
            n988 = property class="DigNum (strict)"(reference=w1413, "Visible"=w1411) -> ()  [unwired: 1 in, 2 out]
            n989 = property class="Enum (strict)"(reference=w1412, "Visible"=w1411) -> ()  [unwired: 1 in, 2 out]
            n990 = property class="VISAName"(reference=w1410, "Visible"=FALSE) -> ()  [unwired: 1 in, 2 out]
          }
          frame #1 {
            n991 = case shown="\"PCS (n.a.)\"" w1416 {
              tunnel: [refnum<class "TCS.lvclass"> refnum ("TCS.lvclass") refnum<class "QCS.lvclass"> refnum ("QCS.lvclass") w1436 w1450 refnum<class "PCS.lvclass"> refnum ("PCS.lvclass")] -> w1415
              tunnel: [w1417 w1435 u16 255 ("Value") u16 255 ("Value") w1455] -> w1414
              frame "TCS" {
                w1420 = u8 2 ("Disabled")
                w1433 = u8 0 ("Disabled")
                n992 = control-ref of="TCS RS232 Port"() -> (w1423:refnum<vi>)
                n993 = control-ref of="Toggle Gated"() -> (w1432:refnum<vi>)
                n994 = control-ref of="Toggle Gated"() -> (w1431:refnum<vi>)
                n995 = control-ref of="Toggle Gated"() -> (w1430:refnum<vi>)
                n996 = control-ref of="Toggle Gated"() -> (w1429:refnum<vi>)
                n997 = control-ref of="CS.QCS Device Nr"() -> (w1425:refnum<vi>)
                n998 = control-ref of="I0"() -> (w1428:refnum<vi>)
                n999 = control-ref of="CS.I0"() -> (w1421:refnum<vi>)
                n1000 = control-ref of="QCS. I0 Mapping"() -> (w1422:refnum<vi>)
                n1001 = property class="Bool (strict)"(reference=w1432, "Disabled"=w1433) -> ()  [unwired: 1 in, 2 out]
                n1002 = property class="Bool (strict)"(reference=w1431, "Disabled"=w1433) -> ()  [unwired: 1 in, 2 out]
                n1003 = property class="Bool (strict)"(reference=w1430, "Disabled"=w1433) -> ()  [unwired: 1 in, 2 out]
                n1004 = property class="Bool (strict)"(reference=w1429, "Disabled"=w1433) -> ()  [unwired: 1 in, 2 out]
                n1005 = property class="Clust (strict)"(reference=w1421, "Disabled"=w1420) -> ()  [unwired: 1 in, 2 out]
                n1006 = property class="Clust (strict)"(reference=w1428, "Disabled"=u8 2) -> ()  [unwired: 1 in, 2 out]
                n1007 = property class="DigNum (strict)"(reference=w1425, "Visible"=FALSE) -> ()  [unwired: 1 in, 2 out]
                n1008 = property class="VISAName"(reference=w1423, "Visible"=TRUE) -> ()  [unwired: 1 in, 2 out]
                n1009 = property class="Enum (strict)"(reference=w1422, "Disabled"=w1420) -> ()  [unwired: 1 in, 2 out]
                n1010 = property on="TCS RS232 Port" class="VISAName"() -> ("Value"=w1418:refnum<visa-resource-name>)  [unwired: 2 in, 2 out]
                n1011 = call "VISA to RS232 Port Nr.vi"("VISA Resource Name"=w1418) -> ("Port Number"=w1417:u8)  [unwired: 1 in]
              }
              frame "QCS v1" {
                n1012 = property on="CS.QCS Device Nr" class="DigNum (strict)"() -> ("Value"=w1435:u16)  [unwired: 2 in, 2 out]
              }
              frame "CS Emulation" {
                w1436 = refnum<class "CS Emulation.lvclass"> refnum  # CS Emulation.lvclass
                n1013 = control-ref of="CS.QCS Device Nr"() -> (w1439:refnum<vi>)
                n1014 = property class="DigNum (strict)"(reference=w1439, "Visible"=FALSE) -> ()  [unwired: 1 in, 2 out]
              }
              frame "Disabled", Default {
                w1440 = u8 2 ("Disabled")
                w1450 = refnum<class "CS Emulation.lvclass"> refnum  # CS Emulation.lvclass
                n1015 = control-ref of="CS Indicators Panel"() -> (w1449:refnum<vi>)
                n1016 = control-ref of="I0"() -> (w1444:refnum<vi>)
                n1017 = control-ref of="I1"() -> (w1443:refnum<vi>)
                n1018 = control-ref of="I2"() -> (w1442:refnum<vi>)
                n1019 = control-ref of="I3"() -> (w1441:refnum<vi>)
                n1020 = control-ref of="CS.QCS Device Nr"() -> (w1453:refnum<vi>)
                n1021 = property class="DigNum (strict)"(reference=w1453, "Visible"=FALSE) -> ()  [unwired: 1 in, 2 out]
                n1022 = property class="Clust (strict)"(reference=w1444, "Disabled"=w1440) -> ()  [unwired: 1 in, 2 out]
                n1023 = property class="Clust (strict)"(reference=w1443, "Disabled"=w1440) -> ()  [unwired: 1 in, 2 out]
                n1024 = property class="Clust (strict)"(reference=w1442, "Disabled"=w1440) -> ()  [unwired: 1 in, 2 out]
                n1025 = property class="Clust (strict)"(reference=w1441, "Disabled"=w1440) -> ()  [unwired: 1 in, 2 out]
                n1026 = property class="TabCtl (strict)"(reference=w1449, "Disabled"=w1440) -> ()  [unwired: 1 in, 2 out]
                n1027 = property on="Side Panel" class="TabCtl (strict)"() -> ("Pages"=w1448:refnum<vi>[])  [unwired: 2 in, 2 out]
                n1028 = Index Array(array=w1448, index=1) -> (element=w1447:refnum<vi>)
                n1029 = property class="Page"(reference=w1447, "PageVis"=FALSE ("Page Visible")) -> ()  [unwired: 1 in, 2 out]
              }
              frame "PCS (n.a.)" {
                w1456 = u8 2 ("Disabled")
                n1030 = control-ref of="I0"() -> (w1462:refnum<vi>)
                n1031 = control-ref of="I1"() -> (w1461:refnum<vi>)
                n1032 = control-ref of="CS.I0"() -> (w1460:refnum<vi>)
                n1033 = control-ref of="CS.I1"() -> (w1459:refnum<vi>)
                n1034 = control-ref of="CS Mode"() -> (w1458:refnum<vi>)
                n1035 = control-ref of="QCS. I0 Mapping"() -> (w1457:refnum<vi>)
                n1036 = property class="Clust (strict)"(reference=w1460, "Disabled"=w1456) -> ()  [unwired: 1 in, 2 out]
                n1037 = property class="Clust (strict)"(reference=w1459, "Disabled"=w1456) -> ()  [unwired: 1 in, 2 out]
                n1038 = property class="Clust (strict)"(reference=w1462, "Disabled"=w1456) -> ()  [unwired: 1 in, 2 out]
                n1039 = property class="Clust (strict)"(reference=w1461, "Disabled"=w1456) -> ()  [unwired: 1 in, 2 out]
                n1040 = property class="Enum (strict)"(reference=w1458, "Disabled"=w1456) -> ()  [unwired: 1 in, 2 out]
                n1041 = property class="Enum (strict)"(reference=w1457, "Disabled"=w1456) -> ()  [unwired: 1 in, 2 out]
                n1042 = property on="CS.QCS Device Nr" class="DigNum (strict)"() -> ("Value"=w1455:u16)  [unwired: 2 in, 2 out]
              }
            }
            "_CSClassRef" <- w1415
            n1043 = property on="_CS_Address" class="DigNum (strict)"("Value"=w1414) -> ()  [unwired: 2 in, 2 out]
          }
        }
      }
      event "CS Settings.CS.QCS Device Nr": Value Change {
        # "Set CS port"
        n1044 = event-data() -> ("NewVal"=w1464:u16)  [unwired: 1 in, 5 out]
        n1045 = property on="CS type" class="Enum (strict)"() -> ("Value"=w1465:T56)  [unwired: 2 in, 2 out]
        n1046 = case shown="Default" w1465 {
          tunnel: w1464 -> [_ w1468 _]
          frame Default {
          }
          frame "QCS v1" {
            n1047 = Variant To Data(type=u32 255 ("HW Address"), Variant=w1468) -> (data=w1466:u32)  [unwired: 1 in, 1 out]
            n1048 = property on="_CS_Address" class="DigNum (strict)"("Value"=w1466) -> ()  [unwired: 2 in, 2 out]
          }
          frame "CS Emulation" {
            n1049 = property on="_CS_Address" class="DigNum (strict)"("Value"=u32 255 ("HW Address")) -> ()  [unwired: 2 in, 2 out]
          }
        }
      }
      event "CS Settings.TCS RS232 Port": Value Change {
        # "Set TCS port"
        n1050 = event-data() -> ("NewVal"=w1471:refnum<visa-resource-name>)  [unwired: 1 in, 5 out]
        n1051 = property on="CS type" class="Enum (strict)"() -> ("Value"=w1472:T56)  [unwired: 2 in, 2 out]
        n1052 = case shown="\"TCS\"" w1472 {
          tunnel: w1471 -> [w1475 _]
          frame "TCS" {
            n1053 = Type Cast(type=refnum<visa-resource-name> refnum ("Value"), x=w1475) -> (*(type *) &x=w1474:refnum<visa-resource-name>)
            n1054 = call "VISA to RS232 Port Nr.vi"("VISA Resource Name"=w1474) -> ("Port Number"=w1476:u8)  [unwired: 1 in]
            n1055 = property on="_CS_Address" class="DigNum (strict)"("Value"=w1476) -> ()  [unwired: 2 in, 2 out]
          }
          frame Default {
          }
        }
      }
      event "Load Data": Value Change {
        # "Load data from log files"
        n1056 = event-data() -> ()  [unwired: 1 in, 6 out]
        n1057 = property on="Log Files Folder" class="Path"() -> ("Value"=w1480:path)  [unwired: 2 in, 2 out]
        n1058 = call "File Dialog4"("start path"=w1480) -> ("selected paths"=w1479:path[], "cancelled"=w1478:bool)  [unwired: 11 in, 2 out]
        n1059 = case shown="False" w1478 {
          tunnel: w1479 -> [w1494 _]
          frame False {
            n1060 = property on="Bridge Type" class="Enum (strict)"() -> ("Value"=w1484:T60)  [unwired: 2 in, 2 out]
            n1061 = case shown="Default" w1484 {
              tunnel: [2 ("index")] -> w1483
              tunnel: [10 ("length")] -> w1481
              tunnel: [12 ("index")] -> w1482
              frame Default {
              }
            }
            n1062 = for {
              tunnel: w1494 -> [w1518] mode=indexing
              shift-right: [w1516] -> w1491
              shift-left: string[][] [] ("all rows") -> [w1517]
              # "skip header"
              n1063 = call <vilib>:"Read From Spreadsheet File (string).vi"("file path (dialog if empty)"=w1518) -> ("all rows"=w1514:string[][])  [unwired: 6 in, 4 out]
              n1064 = Array Subset(array=w1514, index (row)=5 ("index")) -> (w1513:string[][])  [unwired: 3 in]
              n1065 = Insert Into Array(array=w1517, new element=w1513) -> (w1516:string[][])  [unwired: 2 in]
            }
            n1066 = Index Array(array=w1491, index (col)=1 ("disabled index (col)")) -> (element=w1488:string[])  [unwired: 1 in]
            n1067 = Array Subset(array=w1491, index (col)=w1483, length (col)=w1481) -> (w1490:string[][])  [unwired: 2 in]
            n1068 = Array Subset(array=w1491, index (col)=w1482, length (col)=w1481) -> (w1489:string[][])  [unwired: 2 in]
            n1069 = Transpose 2D Array(2D array=w1490) -> (transposed array=w1486:string[][])
            n1070 = Transpose 2D Array(2D array=w1489) -> (transposed array=w1485:string[][])
            n1071 = for {
              tunnel: w1486 -> [w1510] mode=indexing
              tunnel: w1485 -> [w1509] mode=indexing
              tunnel: w1488 -> [w1511]
              tunnel: [w1508] -> w1487 mode=indexing
              # "Sort data by date and remove duplicate points"
              n1072 = Fract/Exp String To Number(string=w1510) -> (number=w1505:dbl[])  [unwired: 3 in, 1 out]
              n1073 = Fract/Exp String To Number(string=w1511) -> (number=w1507:dbl[])  [unwired: 3 in, 1 out]
              n1074 = Fract/Exp String To Number(string=w1509) -> (number=w1506:dbl[])  [unwired: 3 in, 1 out]
              n1075 = call <userlib>:"Sort 1D Array (DBL)__ogtk.vi"("Array in"=w1507) -> ("Sorted Pointers"=w1512:i32[], "Sorted Array out"=w1500:dbl[])  [unwired: 9 in]
              n1076 = call <userlib>:"Reorder 1D Array2 (DBL)__ogtk.vi"("indices"=w1512, "array"=w1505) -> ("reordered array"=w1504:dbl[])  [unwired: 9 in]
              n1077 = call <userlib>:"Reorder 1D Array2 (DBL)__ogtk.vi"("indices"=w1512, "array"=w1506) -> ("reordered array"=w1502:dbl[])  [unwired: 9 in]
              n1078 = call <userlib>:"Remove Duplicates from 1D Array (DBL)__ogtk.vi"("Input Array"=w1504) -> ("Output Array"=w1503:dbl[], "indices of removed elements"=w1498:i32[])
              n1079 = call <userlib>:"Delete Elements from 1D Array (DBL)__ogtk.vi"("indices"=w1498, "array"=w1502) -> ("array w/ subset deleted"=w1501:dbl[])  [unwired: 8 in, 1 out]
              n1080 = call <userlib>:"Delete Elements from 1D Array (DBL)__ogtk.vi"("indices"=w1498, "array"=w1500) -> ("array w/ subset deleted"=w1499:dbl[])  [unwired: 8 in, 1 out]
              n1081 = Bundle("Output Array"=w1503, "array w/ subset deleted"=w1501, "array w/ subset deleted"=w1499) -> (w1508:T71)  [unwired: 1 in]
            }
            n1082 = local write "Data Array"(w1487) -> ()
          }
          frame True {
          }
        }
      }
      event "Save Data 2": Value Change {
        # "Load data from log files"
        n1083 = event-data() -> ()  [unwired: 1 in, 6 out]
        n1084 = property on="Log Files Folder" class="Path"() -> ("Value"=w1524:path)  [unwired: 2 in, 2 out]
        n1085 = call "File Dialog"("start path"=w1524, "pattern (all files)"="*.dat", "pattern label"="Log files") -> ("selected path"=w1522:path, "cancelled"=w1523:bool)  [unwired: 9 in, 2 out]
        n1086 = case shown="False" w1523 {
          tunnel: w1522 -> [w1529 _]
          frame False {
            (unwired) 30 ("dimension size")
            n1087 = local read "Data Array"() -> (w1530:T28)
            n1088 = for {
              tunnel: w1530 -> [w1543] mode=indexing
              tunnel: [w1534] -> w1528 mode=indexing
              shift-right: [w1532] -> w1526
              shift-left: string[][] [] -> [w1533]
              n1089 = Unbundle By Name(w1543) -> ("Time"=w1540:dbl[], "R"=w1539:dbl[], "T"=w1535:dbl[])
              n1090 = property on="Data Logging Settings" class="Clust (strict)"() -> ("Value"=w1542:T37)  [unwired: 2 in, 2 out]
              n1091 = Unbundle By Name(w1542) -> ("Date Format"=w1541:string)
              n1092 = Array Size(array=w1535) -> (size(s)=w1534:i32)
              n1093 = for {
                tunnel: w1541 -> [w1546]
                tunnel: [w1545] -> w1538 mode=indexing
                tunnel: w1540 -> [w1544] mode=indexing
                n1094 = Format Date/Time String(time format string (%c)=w1546, seconds (now)=w1544) -> (date/time string=w1545:string)  [unwired: 1 in]
              }
              n1095 = Number To Fractional String(number=w1539) -> (F-format string=w1537:string[])  [unwired: 3 in]
              n1096 = Number To Fractional String(number=w1535) -> (F-format string=w1536:string[])  [unwired: 3 in]
              n1097 = Build Array(w1538, w1537, w1536) -> (w1531:string[][])
              n1098 = Build Array (concatenate)(w1533, w1531) -> (w1532:string[][])
            }
            n1099 = Array Max & Min(array=w1528) -> ()  [unwired: 4 out]
            n1100 = call "Write To Spreadsheet File (string) w Error.vi"("transpose? (no:F)"=TRUE, "2D data"=w1526, "file path (dialog if empty)"=w1529) -> ()  [unwired: 7 in, 2 out]
          }
          frame True {
          }
        }
      }
      event "Plot-save-screen": Value Change {
        n1101 = event-data() -> ()  [unwired: 1 in, 6 out]
        n1102 = property on="Log Files Folder" class="Path"() -> ("Value"=w1552:path)  [unwired: 2 in, 2 out]
        n1103 = call "File Dialog7"("start path"=w1552, "pattern (all files)"="*.dat", "pattern label"="Log files") -> ("selected path"=w1550:path, "cancelled"=w1551:bool)  [unwired: 9 in, 2 out]
        n1104 = case shown="False" w1551 {
          tunnel: w1550 -> [w1577 _]
          frame False {
            # "!!NOTE:This routine assumes that XY graph is \ncontrol #0 on tab page!!"
            n1105 = property on="Channels Panel" class="TabCtl (strict)"() -> ("Pages"=w1575:refnum<vi>[], "Value"=w1574:T8)  [unwired: 2 in, 2 out]
            n1106 = Index Array(array=w1575, index=w1574) -> (element=w1573:refnum<vi>)
            n1107 = property class="Page"(reference=w1573) -> ("ControlsOnPage"=w1570:refnum<vi>[])  [unwired: 1 in, 2 out]
            n1108 = Index Array(array=w1570, index=0) -> (element=w1572:refnum<vi>)
            n1109 = control-ref of="R-Plot 0"() -> (w1568:refnum<vi>)
            n1110 = Type Cast(type=w1568, x=w1572) -> (*(type *) &x=w1569:refnum<vi>)
            n1111 = property class="XYGraph (strict)"(reference=w1569) -> ("Value"=w1567:cluster{dbl[], dbl[]}, "XScale.Maximum"=w1566:dbl, "XScale.Minimum"=w1565:dbl)  [unwired: 1 in, 2 out]
            n1112 = Unbundle(w1567) -> (w1564:dbl[], w1563:dbl[])
            n1113 = call <userlib>:"MGI Threshold 1D Array Extended.vi"("Threshold Y"=w1566, "Y Value[]"=w1564) -> ("Extended Fractional Index"=w1554:dbl)  [unwired: 1 in]
            n1114 = call <userlib>:"MGI Threshold 1D Array Extended.vi"("Threshold Y"=w1565, "Y Value[]"=w1564) -> ("Extended Fractional Index"=w1553:dbl)  [unwired: 1 in]
            n1115 = Subtract(x=w1554, y=w1553) -> (x-y=w1576:dbl)
            n1116 = Array Subset(array=w1564, index=w1553, length=w1576) -> (w1558:dbl[])
            n1117 = Array Subset(array=w1563, index=w1553, length=w1576) -> (w1556:dbl[])
            n1118 = property on="Data Logging Settings" class="Clust (strict)"() -> ("Value"=w1560:T37)  [unwired: 2 in, 2 out]
            n1119 = Unbundle By Name(w1560) -> ("Date Format"=w1559:string)
            n1120 = Number To Fractional String(number=w1556) -> (F-format string=w1555:string[])  [unwired: 3 in]
            n1121 = for {
              tunnel: w1559 -> [w1580]
              tunnel: [w1579] -> w1557 mode=indexing
              tunnel: w1558 -> [w1578] mode=indexing
              n1122 = Format Date/Time String(time format string (%c)=w1580, seconds (now)=w1578) -> (date/time string=w1579:string)  [unwired: 1 in]
            }
            n1123 = Build Array(w1557, w1555) -> (w1562:string[][])
            n1124 = call <vilib>:"Write To Spreadsheet File (string).vi"("transpose? (no:F)"=TRUE, "2D data"=w1562, "file path (dialog if empty)"=w1577) -> ()  [unwired: 5 in, 1 out]
          }
          frame True {
          }
        }
      }
      event "Plot-Save All": Value Change {
        n1125 = event-data() -> ()  [unwired: 1 in, 6 out]
        n1126 = property on="Log Files Folder" class="Path"() -> ("Value"=w1586:path)  [unwired: 2 in, 2 out]
        n1127 = call "File Dialog8"("start path"=w1586, "pattern (all files)"="*.dat", "pattern label"="Log files") -> ("selected path"=w1584:path, "cancelled"=w1585:bool)  [unwired: 9 in, 2 out]
        n1128 = case shown="False" w1585 {
          tunnel: w1584 -> [w1604 _]
          frame False {
            # "!!NOTE:This routine assumes that XY graph is \ncontrol #0 on tab page!!"
            n1129 = property on="Channels Panel" class="TabCtl (strict)"() -> ("Pages"=w1603:refnum<vi>[], "Value"=w1602:T8)  [unwired: 2 in, 2 out]
            n1130 = Index Array(array=w1603, index=w1602) -> (element=w1601:refnum<vi>)
            n1131 = property class="Page"(reference=w1601) -> ("ControlsOnPage"=w1598:refnum<vi>[])  [unwired: 1 in, 2 out]
            n1132 = Index Array(array=w1598, index=0) -> (element=w1600:refnum<vi>)
            n1133 = control-ref of="R-Plot 0"() -> (w1596:refnum<vi>)
            n1134 = Type Cast(type=w1596, x=w1600) -> (*(type *) &x=w1597:refnum<vi>)
            n1135 = property class="XYGraph (strict)"(reference=w1597) -> ("Value"=w1595:cluster{dbl[], dbl[]})  [unwired: 1 in, 2 out]
            n1136 = Unbundle(w1595) -> (w1588:dbl[], w1587:dbl[])
            n1137 = property on="Data Logging Settings" class="Clust (strict)"() -> ("Value"=w1592:T37)  [unwired: 2 in, 2 out]
            n1138 = Unbundle By Name(w1592) -> ("Date Format"=w1591:string)
            n1139 = Number To Fractional String(number=w1587) -> (F-format string=w1589:string[])  [unwired: 3 in]
            n1140 = for {
              tunnel: w1591 -> [w1607]
              tunnel: [w1606] -> w1590 mode=indexing
              tunnel: w1588 -> [w1605] mode=indexing
              n1141 = Format Date/Time String(time format string (%c)=w1607, seconds (now)=w1605) -> (date/time string=w1606:string)  [unwired: 1 in]
            }
            n1142 = Build Array(w1590, w1589) -> (w1594:string[][])
            n1143 = call <vilib>:"Write To Spreadsheet File (string).vi"("transpose? (no:F)"=TRUE, "2D data"=w1594, "file path (dialog if empty)"=w1604) -> ()  [unwired: 5 in, 1 out]
          }
          frame True {
          }
        }
      }
      event "_CurrentsChanged": Value Change {
        # "New values for currents were entered by user/automode-> write new data to CS"
        n1144 = event-data() -> ()  [unwired: 1 in, 6 out]
        n1145 = local read "_CSClassRef"() -> (w1613:refnum<class "CS.lvclass">)
        n1146 = property on="CS status" class="Clust (strict)"() -> ("Value"=w1610:errorcluster)  [unwired: 2 in, 2 out]
        n1147 = call-dynamic "Read.vi"("CS in"=w1613, "error in (no error)"=w1610, "Optional"=TRUE ("Unused")) -> ("CS out"=w1612:refnum<class "CS.lvclass">, "error out"=w1609:errorcluster)  [unwired: 11 in, 4 out]
        n1148 = local write "_CSClassRef"(w1612) -> ()
        n1149 = property on="CS status" class="Clust (strict)"("Value"=w1609) -> ()  [unwired: 2 in, 2 out]
      }
      event "CS.QCS I0 Output": Value Change {
        # "Switch QCS channel 0 to aux output"
        n1150 = event-data() -> ("OldVal"=w1621:T38, "NewVal"=w1616:T38)  [unwired: 1 in, 4 out]
        n1151 = To Long Integer(number=w1616) -> (32bit integer=→"QCS. I0 Mapping":i32)
        n1152 = local read "_CSClassRef"() -> (w1619:refnum<class "CS.lvclass">)
        n1153 = property on="CS status" class="Clust (strict)"() -> ("Value"=w1620:errorcluster)  [unwired: 2 in, 2 out]
        n1154 = call-dynamic "Switch Output Channel.vi"("error in (no error)"=w1620, "New Channel"=w1616, "Old Channel"=w1621, "CS in"=w1619) -> ("error out"=w1617:errorcluster, "CS out"=w1618:refnum<class "CS.lvclass">)  [unwired: 6 in]
        n1155 = local write "_CSClassRef"(w1618) -> ()
        n1156 = property on="CS status" class="Clust (strict)"("Value"=w1617) -> ()  [unwired: 2 in, 2 out]
      }
      event "T Sweep.Start": Value Change {
        # "Setup and Start Current/Temperature sweep for CS channel 3"
        n1157 = event-data() -> ("CtlRef"=w1623:refnum<vi>, "NewVal"=w1624:bool)  [unwired: 1 in, 4 out]
        n1158 = case shown="False" w1624 {
          tunnel: w1623 -> [w1625 w1628]
          frame False {
            n1159 = property class="Bool (strict)"(reference=w1625, "Caption.Text"="Start") -> ()  [unwired: 1 in, 2 out]
          }
          frame True {
            n1160 = property on="Start value" class="DigNum (strict)"() -> ("Value"=w1629:dbl)  [unwired: 2 in, 2 out]
            n1161 = property class="Bool (strict)"(reference=w1628, "Caption.Text"="Stop") -> ()  [unwired: 1 in, 2 out]
            n1162 = property on="Current" class="DigNum (strict)"("Val(Sgnl)"=w1629) -> ()  [unwired: 2 in, 2 out]
          }
        }
      }
      event "T Sweep.I_next": Value Change {
        # "Go to next step in Current/Temperature sweep for CS channel 3"
        n1163 = event-data() -> ()  [unwired: 1 in, 6 out]
        n1164 = property on="I_next" class="Bool (strict)"("Value"=FALSE) -> ()  [unwired: 2 in, 2 out]
        n1165 = call "Current Time(double).vi"() -> ("Current Time (double)"=w1631:dbl)  [unwired: 6 in, 1 out]
        n1166 = local write "_TimeOld"(w1631) -> ()
        n1167 = property on="Current" class="DigNum (strict)"() -> ("Value"=w1632:dbl)  [unwired: 2 in, 2 out]
        n1168 = property on="Step" class="DigNum (strict)"() -> ("Value"=w1637:dbl)  [unwired: 2 in, 2 out]
        n1169 = Add(x=w1632, y=w1637) -> (x+y=w1636:dbl)
        n1170 = property on="End value" class="DigNum (strict)"() -> ("Value"=w1635:dbl)  [unwired: 2 in, 2 out]
        n1171 = property on="Start value" class="DigNum (strict)"() -> ("Value"=w1634:dbl)  [unwired: 2 in, 2 out]
        n1172 = In Range and Coerce(upper limit=w1635, x=w1636, lower limit=w1634) -> (coerced(x)=w1633:dbl)  [unwired: 1 out]
        n1173 = property on="Current" class="DigNum (strict)"("Val(Sgnl)"=w1633) -> ()  [unwired: 2 in, 2 out]
      }
      event "T Sweep.I_prev": Value Change {
        # "Go to previous step in Current/Temperature sweep for CS channel 3"
        n1174 = event-data() -> ()  [unwired: 1 in, 6 out]
        n1175 = call "Current Time(double).vi"() -> ("Current Time (double)"=w1640:dbl)  [unwired: 6 in, 1 out]
        n1176 = property on="I_prev" class="Bool (strict)"("Value"=FALSE) -> ()  [unwired: 2 in, 2 out]
        n1177 = local write "_TimeOld"(w1640) -> ()
        n1178 = property on="Current" class="DigNum (strict)"() -> ("Value"=w1642:dbl)  [unwired: 2 in, 2 out]
        n1179 = property on="Step" class="DigNum (strict)"() -> ("Value"=w1647:dbl)  [unwired: 2 in, 2 out]
        n1180 = Subtract(x=w1642, y=w1647) -> (x-y=w1646:dbl)
        n1181 = property on="End value" class="DigNum (strict)"() -> ("Value"=w1645:dbl)  [unwired: 2 in, 2 out]
        n1182 = property on="Start value" class="DigNum (strict)"() -> ("Value"=w1644:dbl)  [unwired: 2 in, 2 out]
        n1183 = In Range and Coerce(upper limit=w1645, x=w1646, lower limit=w1644) -> (coerced(x)=w1643:dbl)  [unwired: 1 out]
        n1184 = property on="Current" class="DigNum (strict)"("Val(Sgnl)"=w1643) -> ()  [unwired: 2 in, 2 out]
      }
      event User Event {
        # "Reset the PID loop"
        n1185 = event-data() -> ()  [unwired: 1 in, 5 out]
        n1186 = local write "CS.Mode1.PID Error"(0.0 ("T_error")) -> ()
      }
      event "Minimize UI 1", "Minimize UI 2": Value Change {
        (unwired) 29 ("Splitter Position")
        (unwired) 534 ("Numeric 2")
        # "Shrink/restore the program window"
        # "726"
        # "222"
        # "1243"
        # "816"
        n1187 = event-data() -> ()  [unwired: 1 in, 6 out]
        n1188 = case shown="True" "Minimize UI 1" {
          tunnel: "Minimize UI 2" -> [_ w1678]
          frame True {
            (unwired) T55."Disabled" ("Value")
            n1189 = property on="CS type" class="Enum (strict)"() -> ("Value"=w1664:T56)  [unwired: 2 in, 2 out]
            n1190 = property on="Bridge Type" class="Enum (strict)"() -> ("Value"=w1659:T60)  [unwired: 2 in, 2 out]
            n1191 = Equal?(x=w1659, y=T55."Disabled" ("Value")) -> (x = y?=w1657:bool)
            n1192 = Equal?(x=w1664, y=T56."Disabled" ("Value")) -> (x = y?=w1663:bool)
            n1193 = property on="Data History/RT Settings" class="TabCtl (strict)"("Value"=enum32{"History", "Settings"}."History" ("Data History")) -> ()  [unwired: 2 in, 2 out]
            n1194 = Exclusive Or(1:w1657, 2:w1663) -> (0:w1656:bool)
            n1195 = property on="Mode Buttons" class="RadioBtnsControl (strict)"("Disabled"=u8 2, "Val(Sgnl)"=T54."No Selection" ("Value (Signaling)")) -> ()  [unwired: 2 in, 2 out]
            n1196 = property class="VI"() -> ("Front Panel.PanelBounds"=w1666:T72)  [unwired: 2 in, 2 out]
            n1197 = Select(t=i16 105 ("y"), s=w1656, f=i16 169 ("y")) -> (s? t:f=w1660:i16)
            n1198 = Unbundle By Name(w1666) -> ("Left"=w1672:i16, "Top"=w1669:i16)
            n1199 = property on="Splitter 3" class="Splitter"("Position"=29 ("Splitter Position")) -> (error out=w1658:errorcluster)  [unwired: 2 in, 1 out]
            n1200 = Add(x=i16 806 ("right"), y=w1672) -> (x+y=w1671:i16)
            n1201 = Add(x=w1669, y=w1660) -> (x+y=w1668:i16)
            n1202 = Bundle By Name(cluster=w1666, "Right"=w1671, "Bottom"=w1668) -> (w1673:T72)
            n1203 = case shown="True" w1657 {
              tunnel: w1658 -> [_ w1676]
              frame False {
              }
              frame True {
                n1204 = property on="Splitter 4" class="Splitter"(error in=w1676, "Position"=32 ("Splitter Position")) -> ()  [unwired: 1 in, 2 out]
              }
            }
            n1205 = property class="VI"("Front Panel.PanelBounds"=w1673) -> ()  [unwired: 2 in, 2 out]
          }
          frame False {
            n1206 = property class="VI"() -> ("Front Panel.PanelBounds"=w1685:T72)  [unwired: 2 in, 2 out]
            n1207 = property on="Channels Panel" class="TabCtl (strict)"() -> ("Value"=w1693:T8)  [unwired: 2 in, 2 out]
            n1208 = Unbundle By Name(w1685) -> ("Left"=w1691:i16, "Top"=w1689:i16)
            n1209 = property on="Channels Panel" class="TabCtl (strict)"("Val(Sgnl)"=w1693) -> ()  [unwired: 2 in, 2 out]
            n1210 = Select(t=i16 806 ("right"), s=w1678, f=i16 1206 ("right")) -> (s? t:f=w1682:i16)
            n1211 = Add(x=w1682, y=w1691) -> (x+y=w1690:i16)
            n1212 = Add(x=w1689, y=i16 702) -> (x+y=w1687:i16)
            n1213 = Bundle By Name(cluster=w1685, "Right"=w1690, "Bottom"=w1687) -> (w1692:T72)
            n1214 = property on="Mode Buttons" class="RadioBtnsControl (strict)"("Disabled"=u8 0) -> ()  [unwired: 2 in, 2 out]
            n1215 = property class="VI"("Front Panel.PanelBounds"=w1692) -> (error out=w1679:errorcluster)  [unwired: 2 in, 1 out]
            n1216 = property on="Splitter 3" class="Splitter"(error in=w1679, "Position"=559 ("Splitter Position")) -> (error out=w1683:errorcluster)  [unwired: 1 in, 1 out]
            n1217 = property on="Splitter 4" class="Splitter"(error in=w1683, "Position"=635 ("Splitter Position")) -> ()  [unwired: 1 in, 2 out]
          }
        }
        n1218 = property on="Splitter 2" class="Splitter"("Position"=805 ("Splitter Position")) -> ()  [unwired: 2 in, 2 out]
      }
      event "Copy to Clipboard": Value Change {
        # "Copy current values to the clipboard"
        n1219 = event-data() -> ()  [unwired: 1 in, 6 out]
        n1220 = property on="_ScanData" class="Arr (strict)"() -> ("Value"=w1699:dbl[])  [unwired: 2 in, 2 out]
        n1221 = property on="T Array" class="Arr (strict)"() -> ("Value"=w1698:dbl[])  [unwired: 2 in, 2 out]
        n1222 = Build Array(w1699, w1698) -> (w1697:dbl[][])
        n1223 = Transpose 2D Array(2D array=w1697) -> (transposed array=w1696:dbl[][])
        n1224 = Array To Spreadsheet String(delimiter (Tab)="\t", array=w1696, 3:"%.4g" ("format string")) -> (spreadsheet string=w1702:string)
        n1225 = invoke class="App" method="Clipboard.Write"("Param 0"=w1702) -> ()  [unwired: 3 in, 4 out]
      }
      event "Show PID graph?": Value Change {
        # "Display plots with the PID parameters vs time for debugging"
        n1226 = event-data() -> ("NewVal"=w1704:bool)  [unwired: 1 in, 5 out]
        n1227 = property on="Channels Panel" class="TabCtl (strict)"() -> ("Pages"=w1707:refnum<vi>[])  [unwired: 2 in, 2 out]
        n1228 = Reverse 1D Array(array=w1707) -> (reversed array=w1706:refnum<vi>[])
        n1229 = Index Array(array=w1706) -> (element=w1705:refnum<vi>)  [unwired: 1 in]
        n1230 = property class="Page"(reference=w1705, "PageVis"=w1704) -> ()  [unwired: 1 in, 2 out]
      }
      event "I0.uA", "I1.uA", "I2.uA", "I3.uA": Mouse Up {
        # "Show curent edit filed on double clicking the current indicator. Set the field to the actual current value."
        n1231 = event-data() -> ("Mods.Double Click"=w1710:bool, "CtlRef"=w1709:refnum<vi>)  [unwired: 1 in, 5 out]
        n1232 = case shown="True" w1710 {
          tunnel: w1709 -> [_ w1721]
          frame False {
          }
          frame True {
            w1717 = TRUE ("Visible")
            n1233 = property class="Str"(reference=w1721) -> ("Owner"=w1720:refnum<vi>)  [unwired: 1 in, 2 out]
            n1234 = control-ref of="uA 0"() -> (w1727:refnum<vi>)
            n1235 = control-ref of="uA 1"() -> (w1730:refnum<vi>)
            n1236 = control-ref of="uA 2"() -> (w1729:refnum<vi>)
            n1237 = control-ref of="uA 3"() -> (w1728:refnum<vi>)
            n1238 = control-ref of="I0"() -> (w1718:refnum<vi>)
            n1239 = control-ref of="I1"() -> (w1724:refnum<vi>)
            n1240 = control-ref of="I2"() -> (w1723:refnum<vi>)
            n1241 = control-ref of="I3"() -> (w1716:refnum<vi>)
            n1242 = property on="CS.Current Value" class="Arr (strict)"() -> ("Value"=w1715:dbl[])  [unwired: 2 in, 2 out]
            n1243 = Type Cast(type=w1716, x=w1720) -> (*(type *) &x=w1719:refnum<vi>)
            n1244 = Build Array(w1727, w1730, w1729, w1728) -> (w1726:refnum<vi>[])
            n1245 = Build Array(w1718, w1724, w1723, w1716) -> (w1722:refnum<vi>[])
            n1246 = Search 1D Array(1D array=w1722, element=w1719) -> (index of element=w1714:i32)  [unwired: 1 in]
            n1247 = Index Array(array=w1715, index=w1714) -> (element=w1713:dbl)
            n1248 = Index Array(array=w1726, index=w1714) -> (element=w1725:refnum<vi>)
            n1249 = Multiply(x=1000.0, y=w1713) -> (x*y=w1712:dbl)
            n1250 = property on="Property Node" class="DigNum (strict)"(reference=w1725, "Value"=w1712, "Visible"=w1717, "Key Focus"=w1717) -> ()  [unwired: 1 in, 2 out]
          }
        }
      }
      event "I0.current flows", "I1.current flows", "I2.current flows", "I3.current flows": Mouse Up {
        # "Toggle the current channel by double clickin on the \"On\" led in the current indicator."
        n1251 = event-data() -> ("CtlRef"=w1732:refnum<vi>, "Mods.Double Click"=w1733:bool)  [unwired: 1 in, 5 out]
        n1252 = case shown="True" w1733 {
          tunnel: w1732 -> [_ w1742]
          frame False {
          }
          frame True {
            n1253 = control-ref of="current flows"() -> (w1747:refnum<vi>)
            n1254 = control-ref of="current flows"() -> (w1746:refnum<vi>)
            n1255 = control-ref of="current flows"() -> (w1745:refnum<vi>)
            n1256 = control-ref of="current flows"() -> (w1744:refnum<vi>)
            n1257 = control-ref of="Toggle ON/OFF"() -> (w1741:refnum<vi>)
            n1258 = control-ref of="Toggle ON/OFF"() -> (w1739:refnum<vi>)
            n1259 = control-ref of="Toggle ON/OFF"() -> (w1738:refnum<vi>)
            n1260 = control-ref of="Toggle ON/OFF"() -> (w1740:refnum<vi>)
            n1261 = Build Array(w1747, w1746, w1745, w1744) -> (w1743:refnum<vi>[])
            n1262 = Build Array(w1741, w1739, w1738, w1740) -> (w1737:refnum<vi>[])
            n1263 = Search 1D Array(1D array=w1743, element=w1742) -> (index of element=w1736:i32)  [unwired: 1 in]
            n1264 = Index Array(array=w1737, index=w1736) -> (element=w1735:refnum<vi>)
            n1265 = property class="Bool (strict)"(reference=w1735, "Val(Sgnl)"=TRUE ("Value (Signaling)")) -> ()  [unwired: 1 in, 2 out]
          }
        }
      }
      event "uA 0", "uA 1", "uA 2", "uA 3": Value Change {
        w1750 = refnum<vi> refnum  # Numeric
        w1754 = refnum<vi> refnum  # Enum
        # "User has entered the current by double clicking on the current indicators at the bottom. \nSet range to \"Auto\" and interpret the entered value as [uA]"
        # "!!NOTE:This routine assumes that Current and Range are controls #2 & #3 in current control cluster"
        n1266 = event-data() -> ("CtlRef"=w1762:refnum<vi>, "NewVal"=w1749:u32)  [unwired: 1 in, 4 out]
        n1267 = control-ref of="CS.I0"() -> (w1771:refnum<vi>)
        n1268 = control-ref of="CS.I1"() -> (w1769:refnum<vi>)
        n1269 = control-ref of="CS.I2"() -> (w1770:refnum<vi>)
        n1270 = control-ref of="CS.I3"() -> (w1772:refnum<vi>)
        n1271 = control-ref of="uA 0"() -> (w1764:refnum<vi>)
        n1272 = control-ref of="uA 1"() -> (w1767:refnum<vi>)
        n1273 = control-ref of="uA 2"() -> (w1766:refnum<vi>)
        n1274 = control-ref of="uA 3"() -> (w1765:refnum<vi>)
        n1275 = Build Array(w1771, w1769, w1770, w1772) -> (w1768:refnum<vi>[])
        n1276 = Build Array(w1764, w1767, w1766, w1765) -> (w1763:refnum<vi>[])
        n1277 = Search 1D Array(1D array=w1763, element=w1762) -> (index of element=w1761:i32)  [unwired: 1 in]
        n1278 = Index Array(array=w1768, index=w1761) -> (element=w1760:refnum<vi>)
        n1279 = property class="Clust (strict)"(reference=w1760) -> ("Controls[]"=w1759:refnum<vi>[])  [unwired: 1 in, 2 out]
        n1280 = Index Array(array=w1759, index #1=3 ("index"), index #2=2 ("index")) -> (element #1=w1756:refnum<vi>, element #2=w1752:refnum<vi>)
        n1281 = Type Cast(type=w1750, x=w1752) -> (*(type *) &x=w1751:refnum<vi>)
        n1282 = Type Cast(type=w1754, x=w1756) -> (*(type *) &x=w1755:refnum<vi>)
        n1283 = property on="Property Node" class="Num"(reference=w1751, "Value"=w1749) -> ()  [unwired: 1 in, 2 out]
        n1284 = property on="Property Node" class="Enum"(reference=w1755, "Value"=T57."Auto") -> ()  [unwired: 1 in, 2 out]
      }
      event "_AVSRanges": Value Change {
        # "If user has changed the exitation, update the AVS bridge settings."
        n1285 = event-data() -> ("NewVal"=w1775:T29)  [unwired: 1 in, 5 out]
        n1286 = property on="AVS Exc&Ranges" class="Clust (strict)"() -> ("Value"=w1774:T15)  [unwired: 2 in, 2 out]
        n1287 = call "Combine Excitation&Range.vi"("Ranges"=w1775, "Exc&Ranges In"=w1774) -> ("Exc&Ranges Out"=w1776:T73)
        n1288 = property on="AVS Exc&Ranges" class="Clust (strict)"("Value"=w1776) -> ()  [unwired: 2 in, 2 out]
      }
      event Panel Close? {
        # "Ask for confirmation is user is trying to close the program"
        n1289 = event-data() -> ()  [unwired: 1 in, 4 out]
        n1290 = Two Button Dialog(message="Are you sure you want to quit the program?") -> (T button?=w1779:bool)  [unwired: 2 in]
        n1291 = Not(x=w1779) -> (.not. x?=w1780:bool)
        n1292 = event-data("Discard?"=w1780) -> ()  [unwired: 1 in, 1 out]
      }
      event "Save config": Mouse Up {
        # "Save parameters to the configuration file"
        n1293 = event-data() -> ()  [unwired: 1 in, 8 out]
        n1294 = control-ref of="CS Cannel Names"() -> (w1792:refnum<vi>)
        n1295 = control-ref of="AVS names"() -> (w1791:refnum<vi>)
        n1296 = control-ref of="_CurCalibrations"() -> (w1786:refnum<vi>)
        n1297 = control-ref of="CS.Mode1.PID"() -> (w1784:refnum<vi>)
        n1298 = control-ref of="CS.Mode1.Settings"() -> (w1783:refnum<vi>)
        n1299 = control-ref of="zBridge.Active Channels"() -> (w1785:refnum<vi>)
        n1300 = control-ref of="Bridge settings"() -> (w1797:refnum<vi>)
        n1301 = control-ref of="Runtime Settings"() -> (w1798:refnum<vi>)
        n1302 = control-ref of="CS Settings"() -> (w1796:refnum<vi>)
        n1303 = control-ref of="Sensor Calibrations"() -> (w1799:refnum<vi>)
        n1304 = control-ref of="PID setup"() -> (w1800:refnum<vi>)
        n1305 = control-ref of="Data Logging Settings"() -> (w1795:refnum<vi>)
        n1306 = call "File Dialog3"("start path"=path "C:/LC Data/Configuration" ("Relative path (.)"), "pattern (all files)"="*.ini") -> ("selected path"=w1787:path)  [unwired: 10 in, 3 out]
        n1307 = Build Array(w1785, w1797, w1798, w1796, w1795, w1799, w1800, w1792, w1791, w1786, w1784, w1783) -> (w1793:refnum<vi>[])
        n1308 = call "Save Load Settings to File by Ref with path.vi"("Array of Cluster References"=w1793, "Action"=enum8{"Load", "Save"}."Save", "error in (no error)"=w1790, "Configuration file"=w1787) -> ("error out"=w1789:errorcluster)  [unwired: 5 in]
      }
      event "Load config": Mouse Up {
        # "Load parameters from the configuration file"
        n1309 = event-data() -> ()  [unwired: 1 in, 8 out]
        n1310 = Unbundle By Name(w1804) -> ("UpdateCalibrations"=w1803:refnum<user-event>)
        n1311 = flat-sequence {
          tunnel: [w1829] -> w1814
          tunnel: w1810 -> [w1824]
          tunnel: [w1815] -> w1805
          tunnel: w1801 -> [w1817]
          tunnel: w1814 -> [w1844]
          tunnel: [w1844] -> w1813
          tunnel: [w1842] -> w1806
          tunnel: w1805 -> [w1842]
          tunnel: [w1849] -> w1812
          tunnel: w1813 -> [w1848]
          tunnel: [w1846] -> w1807
          tunnel: w1806 -> [w1846]
          tunnel: w1812 -> [w1855]
          tunnel: [w1855] -> w1811
          tunnel: [w1853] -> w1808
          tunnel: w1807 -> [w1853]
          tunnel: w1811 -> [w1859]
          tunnel: [w1858] -> w1809
          tunnel: w1808 -> [w1857]
          tunnel: w1803 -> [w1856]
          frame #0 {
            n1312 = control-ref of="zBridge.Active Channels"() -> (w1820:refnum<vi>)
            n1313 = control-ref of="Bridge settings"() -> (w1830:refnum<vi>)
            n1314 = control-ref of="Runtime Settings"() -> (w1826:refnum<vi>)
            n1315 = control-ref of="CS Settings"() -> (w1827:refnum<vi>)
            n1316 = control-ref of="Data Logging Settings"() -> (w1828:refnum<vi>)
            n1317 = control-ref of="PID setup"() -> (w1825:refnum<vi>)
            n1318 = control-ref of="CS Cannel Names"() -> (w1823:refnum<vi>)
            n1319 = control-ref of="AVS names"() -> (w1822:refnum<vi>)
            n1320 = control-ref of="_CurCalibrations"() -> (w1821:refnum<vi>)
            n1321 = control-ref of="CS.Mode1.PID"() -> (w1819:refnum<vi>)
            n1322 = control-ref of="CS.Mode1.Settings"() -> (w1818:refnum<vi>)
            n1323 = Build Array(w1820, w1830, w1826, w1827, w1828, w1825, w1823, w1822, w1821, w1819, w1818) -> (w1832:refnum<vi>[])
            n1324 = call "File Dialog2"("start path"=w1817, "pattern (all files)"="*.ini") -> ("selected path"=w1815:path)  [unwired: 10 in, 3 out]
            n1325 = call "Save Load Settings to File by Ref with path.vi"("Array of Cluster References"=w1832, "Action"=enum8{"Load", "Save"}."Load", "error in (no error)"=w1824, "Configuration file"=w1815) -> ("error out"=w1833:errorcluster)  [unwired: 5 in]
            n1326 = disable-structure shown="Disabled" {
              disable-tunnel: w1833 -> [w1836 w1841]
              disable-tunnel: [w1834 w1841] -> w1829
              frame Disabled {
                n1327 = property on="Bridge Type" class="Enum (strict)"(error in=w1836) -> (error out=w1837:errorcluster, "Value"=w1839:T60)  [unwired: 1 in, 1 out]
                n1328 = Equal To 0?(x=w1839) -> (x = 0?=w1840:bool)
                n1329 = property on="AVS GPIB Address" class="VISAName"(error in=w1837, "Visible"=w1840) -> (error out=w1838:errorcluster)  [unwired: 1 in, 1 out]
                n1330 = Not(x=w1840) -> (.not. x?=w1835:bool)
                n1331 = property on="AVS RS232 Port" class="VISAName"(error in=w1838, "Visible"=w1835) -> (error out=w1834:errorcluster)  [unwired: 1 in, 1 out]
              }
              frame Enabled {
              }
            }
          }
          frame #1 {
            n1332 = Wait (ms)(milliseconds to wait=250) -> ()  [unwired: 1 out]
          }
          frame #2 {
            n1333 = control-ref of="Sensor Calibrations"() -> (w1847:refnum<vi>)
            n1334 = control-ref of="_CurCalibrations"() -> (w1845:refnum<vi>)
            n1335 = control-ref of="Calibrations Folder"() -> (w1851:refnum<vi>)
            n1336 = control-ref of="Sensor 1"() -> (w1852:refnum<vi>)
            n1337 = control-ref of="_QuickConvertCal"() -> (w1850:refnum<vi>)
            n1338 = call "ReloadCalibrations.vi"("error in (no error)"=w1848, "Quick convert sensors"=w1850, "CurCalibrations"=w1845, "Calibration files path"=w1851, "Channel1 sensors"=w1852, "Channels list"=w1847) -> ("error out"=w1849:errorcluster)  [unwired: 1 in]
          }
          frame #3 {
            n1339 = Wait (ms)(milliseconds to wait=250) -> ()  [unwired: 1 out]
          }
          frame #4 {
            n1340 = disable-structure shown="Enabled" {
              disable-tunnel: w1859 -> [w1862 w1868]
              disable-tunnel: [w1861 w1870] -> w1858
              disable-tunnel: w1857 -> [w1860 _]
              disable-tunnel: w1856 -> [_ w1867]
              frame Enabled {
                (unwired) T74."HKEY_CURRENT_USER" ("root key (HKEY_LOCAL_MACHINE) 2")
                n1341 = control-ref of="Sensor Calibrations"() -> (w1865:refnum<vi>)
                n1342 = Build Array(w1865) -> (w1864:refnum<vi>[])
                n1343 = call "Save Load Settings to File by Ref with path.vi"("Array of Cluster References"=w1864, "subkey"="SOFTWARE\\Leiden Cryogenics\\TC" ("subkey 2"), "Action"=enum8{"Load", "Save"}."Load", "error in (no error)"=w1862, "Configuration file"=w1860) -> ("error out"=w1861:errorcluster)  [unwired: 4 in]
              }
              frame Disabled {
                n1344 = Generate User Event(user event=w1867, event data cluster="" ("event data"), error in=w1868) -> (error out=w1870:errorcluster)  [unwired: 1 in, 1 out]
              }
            }
          }
        }
        n1345 = Unbundle By Name(w1802) -> ("Config folder"=w1801:path)
      }
      event "zBridge settings": Value Change {
        # "Show parameters menu. (only for zBridge)"
        n1346 = event-data() -> ()  [unwired: 1 in, 6 out]
        n1347 = Unbundle By Name(w1873) -> ("zBridge dll"=w1871:path, "Config folder"=w1872:path)
        n1348 = disable-structure shown="Disabled" {
          disable-tunnel: w1872 -> [w1875 w1880]
          disable-tunnel: w1871 -> [w1874 w1879]
          frame Enabled {
            w1878 = 0 ("Page")
            n1349 = call "SetParFilePath.vi"("path"=w1875, "zDll"=w1874) -> ("error out"=w1876:errorcluster, "zDll out"=w1877:path)  [unwired: 8 in]
            n1350 = call "ParamMenu.vi"("error in (no error)"=w1876, "Subpage"=w1878, "Page"=w1878, "path in"=w1877) -> ()  [unwired: 6 in, 2 out]
          }
          frame Disabled {
            n1351 = call "SetParFilePath.vi"("path"=w1880, "zDll"=w1879) -> ("zDll out"=w1881:path)  [unwired: 8 in, 1 out]
            n1352 = call "zBridgeSettings_1page.vi"("zDll"=w1881) -> ()  [unwired: 10 in, 1 out]
          }
        }
      }
      event "Edit Calibrations": Value Change {
        # "Show calibration files editor. Works with .cal and .cal2 files only"
        n1353 = event-data() -> ("NewVal"=w1893:T11)  [unwired: 1 in, 5 out]
        n1354 = Unbundle By Name(w1885) -> ("UpdateCalibrations"=w1884:refnum<user-event>)
        n1355 = Cluster To Array(cluster=w1893) -> (array=w1892:bool[])
        n1356 = Unbundle By Name(w1883) -> ("Calibrations Folder"=w1882:path)
        n1357 = local read "_CurCalibrations"() -> (w1888:T33)
        n1358 = Search 1D Array(1D array=w1892, element=TRUE) -> (index of element=w1890:i32)  [unwired: 1 in]
        n1359 = Cluster To Array(cluster=w1888) -> (array=w1887:string[])
        n1360 = Index Array(array=w1887, index=w1890) -> (element=w1889:string)
        n1361 = call "Edit Calibration Coefficients.vi"("Calibration Name"=w1889, "Calibration folder"=w1882) -> ("Cancelled?"=w1886:bool)  [unwired: 1 out]
        n1362 = case shown="False" w1886 {
          tunnel: w1884 -> [w1894 _]
          frame False {
            n1363 = Generate User Event(user event=w1894, event data cluster="" ("event data")) -> ()  [unwired: 2 in, 2 out]
          }
          frame True {
          }
        }
      }
      event "Edit calibration": Value Change {
        # "Show calibration files editor for quick convert R->T. Works with .cal and .cal2 files only"
        n1364 = event-data() -> ()  [unwired: 1 in, 6 out]
        n1365 = Unbundle By Name(w1899) -> ("UpdateCalibrations"=w1898:refnum<user-event>)
        n1366 = Unbundle By Name(w1897) -> ("Calibrations Folder"=w1896:path)
        n1367 = property on="_QuickConvertCal" class="Ring (strict)"() -> ("Strings []"=w1902:string[], "Value"=w1903:u16)  [unwired: 2 in, 2 out]
        n1368 = Index Array(array=w1902, index=w1903) -> (element=w1901:string)
        n1369 = call "Edit Calibration Coefficients.vi"("Calibration Name"=w1901, "Calibration folder"=w1896) -> ("Cancelled?"=w1900:bool)  [unwired: 1 out]
        n1370 = case shown="False" w1900 {
          tunnel: w1898 -> [w1904 _]
          frame False {
            n1371 = Generate User Event(user event=w1904, event data cluster="" ("event data")) -> ()  [unwired: 2 in, 2 out]
          }
          frame True {
          }
        }
      }
      event "zBridge params.AVS Name 0", "zBridge params.AVS Name 1", "zBridge params.AVS Name 2", "zBridge params.AVS Name 3", "zBridge params.AVS Name 4", "zBridge params.AVS Name 5", "zBridge params.AVS Name 6", "zBridge params.AVS Name 7", "zBridge params.AVS Name 8", "zBridge params.AVS Name 9": Mouse Down {
        # "Show parameters menu for the channel by double clicking on \"Channel parameters\". (only for zBridge)"
        n1372 = event-data() -> ("CtlRef"=w1910:refnum<vi>, "Mods.Double Click"=w1909:bool, "PlatMods.Alt"=w1908:bool)  [unwired: 1 in, 5 out]
        n1373 = Unbundle By Name(w1907) -> ("zBridge dll"=w1906:path)
        n1374 = case shown="False" w1909 {
          tunnel: w1910 -> [w1914 w1919]
          tunnel: w1908 -> [_ w1918]
          tunnel: w1906 -> [w1911 w1917]
          frame True {
            n1375 = control-ref of="zBridge params"() -> (w1916:refnum<vi>)
            n1376 = property class="Clust (strict)"(reference=w1916) -> ("Controls[]"=w1915:refnum<vi>[])  [unwired: 1 in, 2 out]
            n1377 = Search 1D Array(1D array=w1915, element=w1914) -> (index of element=w1912:i32)  [unwired: 1 in]
            n1378 = call "ParamMenu.vi"("Subpage"=w1912, "Page"=0, "path in"=w1911) -> ()  [unwired: 7 in, 2 out]
          }
          frame False {
            n1379 = case shown="True" w1918 {
              tunnel: w1919 -> [_ w1921]
              tunnel: w1917 -> [_ w1920]
              frame False {
              }
              frame True {
                n1380 = disable-structure shown="Disabled" {
                  disable-tunnel: w1921 -> [w1924 w1928]
                  disable-tunnel: w1920 -> [w1922 _]
                  frame Disabled {
                    # "Show information window.\nTends to crash the acquisition!"
                    n1381 = control-ref of="zBridge params"() -> (w1926:refnum<vi>)
                    n1382 = property class="Clust (strict)"(reference=w1926) -> ("Controls[]"=w1925:refnum<vi>[])  [unwired: 1 in, 2 out]
                    n1383 = Search 1D Array(1D array=w1925, element=w1924) -> (index of element=w1923:i32)  [unwired: 1 in]
                    n1384 = call "Show Info Window.vi"("Data set number"=w1923, "zDll"=w1922) -> ()  [unwired: 8 in, 2 out]
                  }
                  frame Enabled {
                    # "Show information window."
                    n1385 = control-ref of="zBridge params"() -> (w1930:refnum<vi>)
                    n1386 = property class="Clust (strict)"(reference=w1930) -> ("Controls[]"=w1929:refnum<vi>[])  [unwired: 1 in, 2 out]
                    n1387 = Search 1D Array(1D array=w1929, element=w1928) -> (index of element=w1927:i32)  [unwired: 1 in]
                    n1388 = call "Scan Parameters Window.vi"("index"=w1927) -> ()  [unwired: 11 in]
                  }
                }
              }
            }
          }
        }
      }
      event "zBridge.Active Channels.active Channel 0", "zBridge.Active Channels.active Channel 1", "zBridge.Active Channels.active Channel 2", "zBridge.Active Channels.active Channel 3", "zBridge.Active Channels.active Channel 4", "zBridge.Active Channels.active Channel 5", "zBridge.Active Channels.active Channel 6", "zBridge.Active Channels.active Channel 7", "zBridge.Active Channels.active Channel 8", "zBridge.Active Channels.active Channel 9": Mouse Down {
        # "Switch channels On/Off by double clicking on \"Active\" LED. (only for zBridge and AVS47B)"
        n1389 = event-data() -> ("CtlRef"=w1935:refnum<vi>, "Mods.Double Click"=w1933:bool)  [unwired: 1 in, 6 out]
        n1390 = Unbundle By Name(w1932) -> ("zBridge dll"=w1931:path)
        n1391 = property on="Bridge Type" class="Enum (strict)"() -> ("Value"=w1934:T60)  [unwired: 2 in, 2 out]
        n1392 = case shown="True" w1933 {
          tunnel: w1935 -> [_ w1938]
          tunnel: w1934 -> [_ w1942]
          tunnel: w1931 -> [_ w1936]
          frame False {
          }
          frame True {
            n1393 = control-ref of="zBridge.Active Channels"() -> (w1941:refnum<vi>)
            n1394 = property class="Clust (strict)"(reference=w1941) -> ("Controls[]"=w1939:refnum<vi>[])  [unwired: 1 in, 2 out]
            n1395 = property class="Bool (strict)"(reference=w1938) -> ("Value"=w1937:bool)  [unwired: 1 in, 2 out]
            n1396 = Search 1D Array(1D array=w1939, element=w1938) -> (index of element=w1940:i32)  [unwired: 1 in]
            n1397 = case shown="\"Impedance Bridge\"" w1942 {
              tunnel: w1940 -> [_ w1947 w1949]
              tunnel: w1939 -> [_ w1946 _]
              tunnel: w1937 -> [_ w1943 _]
              tunnel: w1936 -> [_ _ w1948]
              frame Default {
              }
              frame "AVS47B (RS232 interface)" {
                n1398 = Index Array(array=w1946, index=w1947) -> (element=w1945:refnum<vi>)
                n1399 = Not(x=w1943) -> (.not. x?=w1944:bool)
                n1400 = property class="Ctl"(reference=w1945, "Value"=w1944) -> ()  [unwired: 1 in, 2 out]
              }
              frame "Impedance Bridge" {
                w1951 = Byte_Params."Active" ("Enum")
                # "Invert Active flag"
                n1401 = call "GetByteParam.vi"("ParNo"=w1951, "SetNo"=w1949, "zDll"=w1948) -> ("return type"=w1953:u8)  [unwired: 6 in, 2 out]
                n1402 = Decrement(x=w1953) -> (x-1=w1952:i8)
                n1403 = Absolute Value(x=w1952) -> (abs(x)=w1950:i8)
                n1404 = call "SetByteParam.vi"("SetNo"=w1949, "ParNo"=w1951, "Data"=w1950, "zDll"=w1948) -> ()  [unwired: 6 in, 2 out]
              }
            }
          }
        }
      }
      event "Small R Cluster.R0", "Small R Cluster.R1", "Small R Cluster.R2", "Small R Cluster.R3", "Small R Cluster.R4", "Small R Cluster.R5", "Small R Cluster.R6", "Small R Cluster.R7", "Small R Cluster.R8", "Small R Cluster.R9", "Small T Cluster.T0", "Small T Cluster.T1", "Small T Cluster.T2", "Small T Cluster.T3", "Small T Cluster.T4", "Small T Cluster.T5", "Small T Cluster.T6", "Small T Cluster.T7", "Small T Cluster.T8", "Small T Cluster.T9": Mouse Down {
        n1405 = event-data() -> ()  [unwired: 1 in, 8 out]
      }
      event Mouse Down {
        n1406 = event-data() -> ()  [unwired: 1 in, 8 out]
      }
      event Value Change {
        # "Update channel names on the small bottom panel when the names are changed."
        n1407 = event-data() -> ("NewVal"=→"AVS names small":T10)  [unwired: 1 in, 5 out]
      }
      event "CS.Mode1.Next": Value Change {
        # "Go to next step in CS auto mode."
        n1408 = event-data() -> ()  [unwired: 1 in, 6 out]
        n1409 = Unbundle By Name(w1961) -> ("TempStabilized"=w1960:refnum<user-event>)
        n1410 = flat-sequence {
          tunnel: w1960 -> [w1963]
          frame #0 {
            n1411 = call "Current Time(double).vi"() -> ("Current Time (double)"=w1962:dbl)  [unwired: 6 in, 1 out]
            n1412 = local write "_TimeOld"(w1962) -> ()
          }
          frame #1 {
            n1413 = Generate User Event(user event=w1963, event data cluster=TRUE ("event data")) -> ()  [unwired: 2 in, 2 out]
          }
        }
      }
      event "CS.Mode1.Auto Advance": Value Change {
        n1414 = event-data() -> ("NewVal"=w1966:bool)  [unwired: 1 in, 5 out]
        n1415 = case shown="True" w1966 {
          frame False {
          }
          frame True {
            # "Set timer to zero (01-01-1904) so the first point is set immediately, w/o wainting for time delay."
            # "If automatic mode is enabled- fire TempStabilized event to record current R,T,I values and start sweeping through TCS channels arrays"
            n1416 = disable-structure shown="Disabled" {
              frame Disabled {
                n1417 = Generate User Event(event data cluster="" ("event data")) -> ()  [unwired: 3 in, 2 out]
                "_TimeOld" <- 0.0 ("Timer")
              }
              frame Enabled {
              }
            }
          }
        }
      }
      event "CS.Mode1.Start", "CS.Mode2.Start": Value Change {
        n1418 = event-data() -> ("NewVal"=w1970:bool)  [unwired: 1 in, 5 out]
        n1419 = case shown="True" w1970 {
          frame False {
          }
          frame True {
            w1971 = TRUE
            # "Switch on the current sources."
            n1420 = property on="ON" class="Bool (strict)"() -> ("Value"=w1975:bool)  [unwired: 2 in, 2 out]
            n1421 = property on="ON" class="Bool (strict)"() -> ("Value"=w1974:bool)  [unwired: 2 in, 2 out]
            n1422 = property on="ON" class="Bool (strict)"() -> ("Value"=w1973:bool)  [unwired: 2 in, 2 out]
            n1423 = property on="ON" class="Bool (strict)"() -> ("Value"=w1972:bool)  [unwired: 2 in, 2 out]
            n1424 = Exclusive Or(1:w1975, 2:w1971) -> (0:w1979:bool)
            n1425 = Exclusive Or(1:w1974, 2:w1971) -> (0:w1977:bool)
            n1426 = Exclusive Or(1:w1973, 2:w1971) -> (0:w1976:bool)
            n1427 = Exclusive Or(1:w1972, 2:w1971) -> (0:w1978:bool)
            n1428 = property on="Toggle ON/OFF" class="Bool (strict)"("Value"=w1979) -> ()  [unwired: 2 in, 2 out]
            n1429 = property on="Toggle ON/OFF" class="Bool (strict)"("Value"=w1977) -> ()  [unwired: 2 in, 2 out]
            n1430 = property on="Toggle ON/OFF" class="Bool (strict)"("Value"=w1976) -> ()  [unwired: 2 in, 2 out]
            n1431 = property on="Toggle ON/OFF" class="Bool (strict)"("Value"=w1978) -> ()  [unwired: 2 in, 2 out]
          }
        }
      }
      event "CS.Mode1.PID.Enabled": Value Change {
        # "Enable/disable the PID loop"
        n1432 = event-data() -> ("NewVal"=w1994:bool)  [unwired: 1 in, 5 out]
        n1433 = Unbundle By Name(w1983) -> ("Reset PID loop"=w1982:refnum<user-event>)
        n1434 = call "IsDisabled.vi"("Enabled?"=w1994) -> ("Numeric"=w1997:i16)
        n1435 = Generate User Event(user event=w1982, event data cluster="" ("event data")) -> ()  [unwired: 2 in, 2 out]
        n1436 = property on="PID setup" class="Clust (strict)"("Disabled"=w1997) -> ()  [unwired: 2 in, 2 out]
        n1437 = property on="FB on" class="Enum (strict)"() -> ("Value"=w1991:enum16{"Resistance", "Temperature"})  [unwired: 2 in, 2 out]
        n1438 = property on="CS.Mode1.PID Channel" class="Enum (strict)"() -> ("Value"=w1981:enum16{"0", "1", "2", "3"})  [unwired: 2 in, 2 out]
        n1439 = property on="Enabled" class="Bool (strict)"() -> ("Value"=w1985:bool)  [unwired: 2 in, 2 out]
        n1440 = Initialize Array(FALSE, 4 ("dimension size")) -> (w1987:bool[])
        n1441 = And(x=TRUE ("new element/subarray"), y=w1985) -> (x .and. y?=w1984:bool)
        n1442 = Index Array(array=string[] ["%#_g uA", "%#_g mK"], index=w1991) -> (element=w1993:string)
        n1443 = Replace Array Subset(array=w1987, new element=w1984, index=w1981) -> (w1990:bool[])
        n1444 = local write "CS.Mode1.PID Column"(w1990) -> ()
        n1445 = Select(t=w1993, s=w1994, f="%#_g uA") -> ()  [unwired: 1 out]
      }
      event "CS.Mode1.Reset PID": Value Change {
        # "Reset the PID loop"
        n1446 = event-data() -> ()  [unwired: 1 in, 6 out]
        n1447 = Unbundle By Name(w2000) -> ("Reset PID loop"=w1999:refnum<user-event>)
        n1448 = Generate User Event(user event=w1999, event data cluster="" ("event data")) -> ()  [unwired: 2 in, 2 out]
      }
      event Value Change {
        n1449 = event-data() -> ("NewVal"=w2006:dbl)  [unwired: 1 in, 5 out]
        n1450 = Unbundle By Name(w2004) -> ("Reset PID loop"=w2003:refnum<user-event>)
        n1451 = Generate User Event(user event=w2003, event data cluster="" ("event data")) -> ()  [unwired: 2 in, 2 out]
        n1452 = property on="Enabled" class="Bool (strict)"() -> ("Value"=w2008:bool)  [unwired: 2 in, 2 out]
        n1453 = Initialize Array(FALSE, 4 ("dimension size")) -> (w2010:bool[])
        n1454 = And(x=TRUE ("new element/subarray"), y=w2008) -> (x .and. y?=w2007:bool)
        n1455 = Replace Array Subset(array=w2010, new element=w2007, index=w2006) -> (→"CS.Mode1.PID Column":bool[])
        n1456 = Index Array(array=string[] ["%#_g uA", "%#_g mK"], index=w2006) -> ()  [unwired: 1 out]
      }
      event "CS.Mode1.List": Value Change {
        n1457 = event-data() -> ("NewVal"=w2019:T23[][])  [unwired: 1 in, 5 out]
        n1458 = local read "CS.Mode1.List:Index"() -> (w2018:i32)
        n1459 = Decrement(x=w2018) -> (x-1=w2017:i32)
        n1460 = Array Size(array=w2019) -> (size(s)=w2021:i32[])
        n1461 = Index Array(array=w2021) -> (element=→"CS.Mode1.List:Count":i32)  [unwired: 1 in]
        n1462 = Index Array(array=w2019, index (row)=w2017) -> (element=→"_CSMode1List[i]":T23[])  [unwired: 1 in]
      }
      event "CS.Mode1.List": Shortcut Menu Activation? {
        n1463 = event-data() -> ()  [unwired: 1 in, 7 out]
        n1464 = event-data() -> ()  [unwired: 2 in, 1 out]
      }
      event "CS.Mode1.List": Shortcut Menu Selection (App) {
        n1465 = event-data() -> ("ItemTag"=w2024:string)  [unwired: 1 in, 7 out]
        n1466 = case shown="\"APP_SC_COPY_DATA\"" w2024 {
          frame Default {
          }
          frame "APP_SC_PASTE_DATA" {
            n1467 = invoke class="App" method="Clipboard.Read"() -> ("Read Clipbrd"=w2027:string)  [unwired: 3 in, 2 out]
            n1468 = Spreadsheet String To Array(format string="%d", spreadsheet string=w2027) -> (array=w2025:dbl[][])  [unwired: 2 in]
            n1469 = local write "CS.Mode1.List"(w2025) -> ()
          }
          frame "APP_SC_COPY_DATA" {
            n1470 = local read "CS.Mode1.List"() -> (w2030:T23[][])
            n1471 = Array To Spreadsheet String(array=w2030, 3:"%d" ("format string")) -> (spreadsheet string=w2028:string)  [unwired: 1 in]
            n1472 = invoke class="App" method="Clipboard.Write"("Param 0"=w2028) -> ()  [unwired: 3 in, 4 out]
          }
        }
      }
      event "CS.Mode1.List:To First": Value Change {
        n1473 = event-data() -> ("OldVal"=w2032:bool)  [unwired: 1 in, 5 out]
        n1474 = local write "CS.Mode1.List:To First"(w2032) -> ()
        n1475 = property on="CS.Mode1.List:Index" class="DigNum (strict)"("Val(Sgnl)"=1 ("Value (Signaling)")) -> ()  [unwired: 2 in, 2 out]
      }
      event "CS.Mode1.List:Next": Value Change {
        n1476 = event-data() -> ("OldVal"=w2035:bool)  [unwired: 1 in, 5 out]
        n1477 = local write "CS.Mode1.List:Next"(w2035) -> ()
        n1478 = local read "CS.Mode1.List:Index"() -> (w2037:i32)
        n1479 = Increment(x=w2037) -> (x+1=w2036:i32)
        n1480 = property on="CS.Mode1.List:Index" class="DigNum (strict)"("Val(Sgnl)"=w2036) -> ()  [unwired: 2 in, 2 out]
      }
      event "CS.Mode1.List:Prev": Value Change {
        n1481 = event-data() -> ("OldVal"=w2039:bool)  [unwired: 1 in, 5 out]
        n1482 = local write "CS.Mode1.List:Prev"(w2039) -> ()
        n1483 = local read "CS.Mode1.List:Index"() -> (w2041:i32)
        n1484 = Decrement(x=w2041) -> (x-1=w2040:i32)
        n1485 = property on="CS.Mode1.List:Index" class="DigNum (strict)"("Val(Sgnl)"=w2040) -> ()  [unwired: 2 in, 2 out]
      }
      event "CS.Mode1.List:Clear": Value Change {
        n1486 = event-data() -> ()  [unwired: 1 in, 6 out]
        n1487 = flat-sequence {
          frame #0 {
            n1488 = local write "CS.Mode1.List"(T23[][] [] ("I_list")) -> ()
          }
          frame #1 {
            n1489 = property on="CS.Mode1.List:To First" class="Bool (strict)"("Val(Sgnl)"=TRUE ("Value (Signaling)")) -> ()  [unwired: 2 in, 2 out]
          }
        }
      }
      event "CS.Mode1.List:Index": Value Change {
        w2066 = 10  # Lines to scroll
        n1490 = event-data() -> ("NewVal"=w2049:i32)  [unwired: 1 in, 5 out]
        n1491 = Array Size(array="CS.Mode1.List") -> (size(s)=w2052:i32[])
        n1492 = Index Array(array=w2052) -> (element=w2050:i32)  [unwired: 1 in]
        n1493 = call "Current Time(double).vi"() -> ("Current Time (double)"=w2046:dbl)  [unwired: 6 in, 1 out]
        n1494 = local write "CS.Mode1.List:Count"(w2050) -> ()
        n1495 = local write "_TimeOld"(w2046) -> ()
        n1496 = In Range and Coerce(upper limit=w2050, x=w2049, lower limit=1) -> (coerced(x)=w2047:i32)  [unwired: 1 out]
        "CS.Mode1.List:Index" <- w2047
        n1497 = Decrement(x=w2047) -> (x-1=w2048:i32)
        n1498 = Initialize Array(FALSE, w2066) -> (w2067:bool[])
        n1499 = Index Array(array="CS.Mode1.List", index (row)=w2048) -> (element=w2069:T23[])  [unwired: 1 in]
        n1500 = local write "_CSMode1List[i]"(w2069) -> ()
        n1501 = Subtract(x=w2048, y=w2066) -> (x-y=w2056:i32)
        n1502 = Increment(x=w2056) -> (x+1=w2055:i32)
        n1503 = Decrement(x=w2066) -> (x-1=w2064:i32)
        n1504 = In Range and Coerce(upper limit=inf, x=w2055, lower limit=0) -> (coerced(x)=w2054:dbl)  [unwired: 1 out]
        n1505 = In Range and Coerce(upper limit=w2064, x=w2048, lower limit=0) -> (coerced(x)=w2061:i32)  [unwired: 1 out]
        n1506 = control-ref of="CS.Mode1.List"() -> (w2059:refnum<vi>)
        n1507 = Build Array(w2054, 0 ("element")) -> (w2060:dbl[])
        n1508 = Replace Array Subset(array=w2067, new element=TRUE ("new element/subarray"), index=w2061) -> (→"CS.Mode1.Row":bool[])
        n1509 = property class="Arr (strict)"(reference=w2059, "Index Values"=w2060) -> ()  [unwired: 1 in, 2 out]
      }
      event "CS.Mode1.List:Save": Value Change {
        n1510 = event-data() -> ()  [unwired: 1 in, 6 out]
        n1511 = call "File Dialog6"() -> ("selected path"=w2073:path, "cancelled"=w2072:bool)  [unwired: 12 in, 2 out]
        n1512 = case shown="False" w2072 {
          tunnel: w2073 -> [w2074 _]
          frame False {
            n1513 = local read "CS.Mode1.List"() -> (w2076:T23[][])
            n1514 = call <vilib>:"Write To Spreadsheet File (DBL).vi"("format (%.3f)"="%.1f", "2D data"=w2076, "file path (dialog if empty)"=w2074) -> ()  [unwired: 5 in, 1 out]
          }
          frame True {
          }
        }
      }
      event "CS.Mode1.List:Load": Value Change {
        n1515 = event-data() -> ()  [unwired: 1 in, 6 out]
        n1516 = call "File Dialog5"() -> ("selected path"=w2078:path, "cancelled"=w2079:bool)  [unwired: 12 in, 2 out]
        n1517 = case shown="False" w2079 {
          tunnel: w2078 -> [w2080 _]
          frame False {
            n1518 = call <vilib>:"Read From Spreadsheet File (DBL).vi"("file path (dialog if empty)"=w2080) -> ("all rows"=w2081:dbl[][])  [unwired: 6 in, 4 out]
            n1519 = local write "CS.Mode1.List"(w2081) -> ()
          }
          frame True {
          }
        }
      }
      event "CS.Mode1.Write To Log": Value Change {
        n1520 = event-data() -> ()  [unwired: 1 in, 6 out]
        n1521 = Unbundle By Name(w2084) -> ("TempStabilized"=w2083:refnum<user-event>)
        n1522 = Generate User Event(user event=w2083, event data cluster=FALSE ("event data")) -> ()  [unwired: 2 in, 2 out]
      }
      event "CS.Mode2.Add Row": Value Change {
        n1523 = event-data() -> ()  [unwired: 1 in, 6 out]
        n1524 = call "Currents-Temp list  - add new range.vi"("List in"="CS.Mode2.List", "Array"="CS.Mode2.New Row") -> ("Sorted list out"=w2088:dbl[][])  [unwired: 3 in, 1 out]
        n1525 = local write "CS.Mode2.List"(w2088) -> ()
      }
      event "CS.Mode2.List": Shortcut Menu Selection (User) {
        n1526 = event-data() -> ("CtlRef"=w2093:refnum<vi>, "Coords"=w2092:T69, "ItemPath"=w2091:string)  [unwired: 1 in]
        n1527 = case shown="\"Erase Range\"" w2091 {
          tunnel: w2093 -> [_ w2099 _ w2105 w2106]
          tunnel: w2092 -> [_ w2098 _ _ _]
          frame Default {
          }
          frame "Erase Range" {
            (unwired) TRUE
            n1528 = call "Get Clicked Array Index.vi"("Coords"=w2098, "Array 2"=w2099) -> ("Clicked Index"=w2095:i32[])  [unwired: 9 in]
            n1529 = local read "CS.Mode2.List"() -> (w2097:dbl[][])
            n1530 = Index Array(array=w2095) -> (element=w2094:i32)  [unwired: 1 in]
            n1531 = call "Currents-Temp list - delete range.vi"("Numeric"=w2094, "I_list 2"=w2097) -> ("I_list"=w2096:dbl[][])  [unwired: 2 in]
            n1532 = local write "CS.Mode2.List"(w2096) -> ()
          }
          frame "Clear List" {
            n1533 = call "Currents-Temp list - check ranges.vi"() -> ("I_list out"=w2100:dbl[][])  [unwired: 5 in]
            n1534 = local write "CS.Mode2.List"(w2100) -> ()
          }
          frame "Copy Data" {
            n1535 = property class="Arr (strict)"(reference=w2105) -> ("Value"=w2101:dbl[][])  [unwired: 1 in, 2 out]
            n1536 = Array To Spreadsheet String(delimiter (Tab)="\t", array=w2101, 3:"%.4g" ("format string")) -> (spreadsheet string=w2104:string)
            n1537 = invoke class="App" method="Clipboard.Write"("Param 0"=w2104) -> ()  [unwired: 3 in, 4 out]
          }
          frame "Paste Data" {
            n1538 = invoke class="App" method="Clipboard.Read"() -> ("Read Clipbrd"=w2107:string)  [unwired: 3 in, 2 out]
            n1539 = Spreadsheet String To Array(delimiter (Tab)="\t", format string="%.4g", spreadsheet string=w2107) -> (array=w2110:dbl[][])  [unwired: 1 in]
            n1540 = property class="Arr (strict)"(reference=w2106, "Value"=w2110) -> ()  [unwired: 1 in, 2 out]
          }
        }
      }
      event "Graph-open popup": Value Change {
        w2122 = 128  # call and forget
        n1541 = event-data() -> ()  [unwired: 1 in, 6 out]
        n1542 = vi-ref "Graph popup.vi"() -> (w2118:refnum<vi>)
        n1543 = property class="VI"(reference=w2118) -> (error out=w2120:errorcluster, "Name"=w2121:string)  [unwired: 1 in, 1 out]
        n1544 = Open VI Reference(type specifier VI Refnum (for type only)=refnum<vi> refnum, vi path=w2121, options=w2122, error in (no error)=w2120) -> (vi reference=w2119:refnum<vi>, error out=w2113:errorcluster)  [unwired: 2 in]
        n1545 = control-ref of="Data"() -> (w2116:refnum<vi>)
        n1546 = local read "Sensor Names"() -> (w2115:T10)
        n1547 = call-by-ref "Start Asynchronous Call"(reference=w2119, error in=w2113, "Data"=w2116, "AVS names"=w2115) -> (reference out=w2114:refnum<vi>, error out=w2112:errorcluster)  [unwired: 18 in]
        n1548 = Close Reference(reference=w2114, error in (no error)=w2112) -> ()  [unwired: 1 out]
      }
      event "ColorBox": Mouse Move {
        n1549 = event-data() -> ("Coords"=w2126:T69)  [unwired: 1 in]
        n1550 = call <vilib>:"Picture to Pixmap.vi"("picture"="Colors") -> ("image data"=w2132:T68)  [unwired: 9 in, 1 out]
        n1551 = property on="Colors" class="Pict"() -> ("Position"=w2125:T76)  [unwired: 2 in, 2 out]
        n1552 = call <vilib>:"Unflatten Pixmap.vi"("image data"=w2132) -> ("24-bit pixmap"=w2127:u32[][])  [unwired: 4 in, 6 out]
        n1553 = Subtract(x=w2126, y=w2125) -> (x-y=w2130:T69)
        n1554 = Unbundle(w2130) -> ("Horizontal"=w2129:i32, "Vertical"=w2128:i32)
        n1555 = Index Array(array=w2127, index (row)=w2128, index (col)=w2129) -> (element=→"Color":u32)
      }
      event "ColorBox": Mouse Down {
        n1556 = event-data() -> ()  [unwired: 1 in, 8 out]
        n1557 = property on="ColorBox" class="TabCtl (strict)"("Visible"=FALSE) -> ()  [unwired: 2 in, 2 out]
      }
      event "Set Color": Value Change {
        n1558 = event-data() -> ()  [unwired: 1 in, 6 out]
        n1559 = property on="ColorBox" class="TabCtl (strict)"("Visible"=TRUE) -> ()  [unwired: 2 in, 2 out]
      }
    }
    "General Error" <- w70
  }
  n1560 = flat-sequence {
    tunnel: w36 -> [w2137]
    frame #0 {
      n1561 = Wait on Occurrence(2:w2137) -> ()  [unwired: 2 in, 1 out]
    }
    frame #1 {
      n1562 = while {
        i -> [w2148]
        stop <- "Stop" stop-if-true
        # "AVS/zBridge read-out"
        n1563 = case shown="False" "Pause" {
          tunnel: w2148 -> [w2151 _]
          frame False {
            # "For the first measurement set Stab.Time=12 s to do autoranging"
            n1564 = property on="Runtime Settings" class="Clust (strict)"() -> ("Value"=w2173:T27)  [unwired: 2 in, 2 out]
            n1565 = local read "zBridge.Active Channels"() -> (w2156:T21)
            n1566 = Unbundle By Name(w2173) -> ("Stabilisation Delay"=w2165:dbl, "Averages"=w2158:u16, "Last Channel"=w2172:i8, "Read AVS channels from"=w2171:i8)
            n1567 = property on="Bridge Type" class="Enum (strict)"() -> ("Value"=w2169:T60)  [unwired: 2 in, 2 out]
            n1568 = call "Split Exc&Range.vi"("Excitations 2"="AVS Exc&Ranges") -> ("Excitations"=w2162:T29, "Ranges"=w2157:T77)  [unwired: 4 in]
            n1569 = property on="_AVS_VISA" class="VISAName"() -> ("Value"=w2170:refnum<visa-resource-name>)  [unwired: 2 in, 2 out]
            n1570 = Cluster To Array(cluster=w2156) -> (array=w2155:bool[])
            n1571 = call "If First Iteration.vi"("Iteration"=w2151, "Value In"=w2165, "Default"=12.0) -> ("Value Out"=w2164:dbl)
            n1572 = case shown="\"Impedance Bridge\"" w2169 {
              tunnel: w2170 -> [w2183 w2194 _ _ _]
              tunnel: w2164 -> [w2179 w2197 w2204 _ _]
              tunnel: w2158 -> [w2180 w2196 _ _ _]
              tunnel: w2172 -> [w2181 w2192 _ _ _]
              tunnel: w2171 -> [w2182 w2193 _ _ _]
              tunnel: w2162 -> [w2184 w2188 _ _ _]
              tunnel: [w2176 w2187 errorcluster {"status"=FALSE, "code"=0, "source"=""} ("error out") w2220 errorcluster {"status"=FALSE, "code"=0, "source"=""} ("error out")] -> w2161
              tunnel: w2157 -> [w2178 w2190 w2205 w2221 w2225]
              tunnel: TRUE ("Autorange") -> [w2174 w2191 _ _ _]
              tunnel: [w2177 w2189 w2205 w2221 w2225] -> w2154
              tunnel: [w2175 w2186 w2203 w2214 dbl[] [] ("Data array")] -> w2159
              tunnel: w2155 -> [_ w2185 _ _ _]
              tunnel: "_ScanData" -> [_ _ _ w2210 _]
              frame "AVS47A (GPIB interface)" {
                # "AVS 47 (GPIB)"
                n1573 = call "AVS47IB_do_single_scan.vi"("AVS Port"=w2183, "Stabilization Delay"=w2179, "Autorange"=w2174, "Number of Averages"=w2180, "Last Channel"=w2181, "First Channel"=w2182, "Excitations"=w2184, "Ranges"=w2178) -> ("error out"=w2176:errorcluster, "R"=w2175:dbl[], "Ranges"=w2177:T78)  [unwired: 3 in, 2 out]
              }
              frame "AVS47B (RS232 interface)" {
                # "AVS 47B (RS232)"
                n1574 = Type Cast(type=refnum<visa-resource-name> refnum ("dup VISA session"), x=w2194) -> (*(type *) &x=w2198:refnum<visa-resource-name>)
                n1575 = call "Scanner.vi"("STABILIZATION  DELAY"=w2197, "FIRST CH TO SCAN"=w2193, "LAST CH TO SCAN"=w2192, "Autorange"=w2191, "AVERAGE COUNT"=w2196, "Excitation"=w2188, "Range"=w2190, "VISA resource"=w2198, "array"=w2185) -> ("RI"=w2186:dbl[], "Range out"=w2189:T79, "error out 2"=w2187:errorcluster)  [unwired: 1 in, 3 out]
              }
              frame "AVS Emulation" {
                (unwired) dbl[] [0.0, 0.0, 0.0, 0.0] ("I")
                n1576 = local read "CS.Automode Current"() -> (w2201:T23[])
                n1577 = Multiply(x=w2204, y=u32 1000 ("milliseconds to wait")) -> (x*y=w2208:dbl)
                n1578 = Wait (ms)(milliseconds to wait=w2208) -> ()  [unwired: 1 out]
                n1579 = Index Array(array=w2201, index=3) -> ()  [unwired: 1 out]
                n1580 = property on="CS.Current Value" class="Arr (strict)"() -> ("Value"=w2207:dbl[])  [unwired: 2 in, 2 out]
                n1581 = Multiply(x=1000.0, y=w2207) -> (x*y=w2199:dbl[])
                n1582 = call "AVS Emulate.vi"("Currents"=w2199, "Sampling time"=w2204) -> ("R"=w2203:dbl[])  [unwired: 1 in, 1 out]
              }
              frame "Impedance Bridge" {
                n1583 = local read "Bridge status"() -> (w2215:errorcluster)
                n1584 = local read "_zBridgeDll"() -> (w2222:path)
                n1585 = call "Read Data from Single Channel.vi"("error in (no error)"=w2215, "zDll"=w2222) -> ("error out"=w2220:errorcluster, "Value"=w2219:dbl, "Scan parameters/Error string"=→"_zBridgeParText":string, "Set number"=w2212:u8, "Error code"=→"Error code":u8, "Unit"=→"_ZBridgeUnit":string, "ScanParameters out"=w2213:T80)  [unwired: 3 in]
                "_zBridgeSetNr" <- w2212
                n1586 = call "ScanParameters FGV.vi"("Action"=Action."Write", "index"=w2212, "ScanParameters in"=w2213) -> ()  [unwired: 8 in, 1 out]
                n1587 = Replace Array Subset(array=w2210, new element=w2219, index=w2212) -> (w2214:dbl[])
              }
              frame "Disabled", Default {
              }
            }
            "Bridge status" <- w2161
            n1588 = property on="_AVSRanges" class="Clust (strict)"("Val(Sgnl)"=w2154) -> ()  [unwired: 2 in, 2 out]
            n1589 = property on="_ScanData" class="Arr (strict)"("Val(Sgnl)"=w2159) -> ()  [unwired: 2 in, 2 out]
            n1590 = property on="Delay" class="DigNum (strict)"() -> ("Value"=w2153:u32)  [unwired: 2 in, 2 out]
            n1591 = Multiply(x=u32 1000, y=w2153) -> (x*y=w2168:u32)
            n1592 = Wait (ms)(milliseconds to wait=w2168) -> ()  [unwired: 1 out]
          }
          frame True {
          }
        }
      }
      n1593 = while {
        stop <- w2227 stop-if-true
        (unwired) errorcluster {"status"=FALSE, "code"=0, "source"=""} ("Value")
        # "Current source control"
        n1594 = property on="CS status" class="Clust (strict)"() -> ("Value"=w2226:errorcluster)  [unwired: 2 in, 2 out]
        n1595 = stacked-sequence {
          seq-local: [w2255 _ _ _] -> [_ w2264 _ _]
          seq-local: [w2254 _ _ _] -> [_ w2263 _ _]
          seq-local: [_ w2264 _ _] -> [_ _ w2274 _]
          seq-local: [_ w2262 _ _] -> [_ _ w2273 _]
          tunnel: w2226 -> [w2253 _ _ _]
          frame #0 {
            # "Write 0 instead of the actual \ncurrent value to log if there \nis no current flowing."
            # "Read current CS status"
            n1596 = local read "_CSClassRef"() -> (w2243:refnum<class "CS.lvclass">)
            n1597 = call-dynamic "Read.vi"("CS in"=w2243, "error in (no error)"=w2253, "Optional"=FALSE) -> ("CS out"=w2255:refnum<class "CS.lvclass">, "I0"=w2246:T81, "I1"=w2247:T81, "I2"=w2248:T81, "I3"=w2249:T81, "error out"=w2254:errorcluster)  [unwired: 11 in]
            n1598 = Unbundle By Name(w2246) -> ("Current (string)"=w2241:string, "I?"=w2240:bool)
            n1599 = Unbundle By Name(w2247) -> ("Current (string)"=w2256:string, "I?"=w2239:bool)
            n1600 = Unbundle By Name(w2248) -> ("Current (string)"=w2244:string, "I?"=w2238:bool)
            n1601 = Unbundle By Name(w2249) -> ("Current (string)"=w2257:string, "I?"=w2237:bool)
            n1602 = call "CS Data Converter.vi"("CS Data"=w2246) -> ("CS Indicator"=→"I0":T82)
            n1603 = call "CS Data Converter.vi"("CS Data"=w2247) -> ("CS Indicator"=→"I1":T82)
            n1604 = call "CS Data Converter.vi"("CS Data"=w2248) -> ("CS Indicator"=→"I2":T82)
            n1605 = call "CS Data Converter.vi"("CS Data"=w2249) -> ("CS Indicator"=→"I3":T82)
            n1606 = Fract/Exp String To Number(string=w2241) -> (number=w2245:dbl)  [unwired: 3 in, 1 out]
            n1607 = Fract/Exp String To Number(string=w2256) -> (number=w2252:dbl)  [unwired: 3 in, 1 out]
            n1608 = Fract/Exp String To Number(string=w2244) -> (number=w2251:dbl)  [unwired: 3 in, 1 out]
            n1609 = Fract/Exp String To Number(string=w2257) -> (number=w2250:dbl)  [unwired: 3 in, 1 out]
            n1610 = Build Array(w2240, w2239, w2238, w2237) -> (w2236:bool[])
            n1611 = Not(x=w2236) -> (.not. x?=w2232:bool[])
            n1612 = Build Array(w2245, w2252, w2251, w2250) -> (w2235:dbl[])
            "CS.Current Value" <- w2235
            n1613 = for {
              tunnel: w2232 -> [w2261] mode=indexing
              tunnel: w2235 -> [w2260] mode=indexing
              tunnel: dbl[] [0.0, 0.0, 0.0, 0.0] ("t") -> [w2259] mode=indexing
              tunnel: [w2258] -> w2233 mode=indexing
              n1614 = Select(t=w2259, s=w2261, f=w2260) -> (s? t:f=w2258:dbl)
            }
            "CS.Actual Current" <- w2233
          }
          frame #1 {
            n1615 = Wait (ms)(milliseconds to wait=100) -> ()  [unwired: 1 out]
            n1616 = call <vilib>:"Clear Errors.vi"("error in (no error)"=w2263) -> ("error out"=w2262:errorcluster)  [unwired: 5 in, 1 out]
          }
          frame #2 {
            # "Only send data to CS if\nnew value was entered"
            # "Set CS status"
            n1617 = call "CS OnOff & Gated and Current & Range.vi"("I in"="CS.I0") -> ("OnOff & Gated"=w2285:T83, "Current & Range"=w2270:T84, "I out"=w2278:T85)  [unwired: 2 in]
            n1618 = call "CS OnOff & Gated and Current & Range.vi"("I in"="CS.I1") -> ("OnOff & Gated"=w2284:T83, "Current & Range"=w2269:T84, "I out"=w2275:T85)  [unwired: 2 in]
            n1619 = call "CS OnOff & Gated and Current & Range.vi"("I in"="CS.I2") -> ("OnOff & Gated"=w2281:T83, "Current & Range"=w2268:T84, "I out"=w2276:T85)  [unwired: 2 in]
            n1620 = call "CS OnOff & Gated and Current & Range.vi"("I in"="CS.I3") -> ("OnOff & Gated"=w2280:T83, "Current & Range"=w2267:T84, "I out"=w2277:T85)  [unwired: 2 in]
            n1621 = local write "CS.I0"(w2278) -> ()
            n1622 = local write "CS.I1"(w2275) -> ()
            n1623 = local write "CS.I2"(w2276) -> ()
            n1624 = local write "CS.I3"(w2277) -> ()
            n1625 = local read "CS.Automode Current"() -> (w2266:T23[])
            n1626 = Equal To 0?(x="CS.Mode") -> (x = 0?=w2271:bool)
            n1627 = call "CS_set_channels.vi"("CS in"=w2274, "Current & Range0"=w2270, "Current & Range1"=w2269, "Current & Range 2"=w2268, "Current & Range3"=w2267, "error out"=w2273, "I_automode"=w2266, "Auto?"=w2271) -> ("CS.lvclass out"=w2290:refnum<class "CS.lvclass">, "Current Changed?"=w2287:bool, "error out 2"=w2291:errorcluster)  [unwired: 9 in]
            n1628 = call-dynamic "Set Mode.vi"("CS.lvclass in"=w2290, "On&G 0"=w2285, "On&G 1"=w2284, "On&G 2"=w2281, "On&G 3"=w2280, "error in (no error)"=w2291) -> ("CS.lvclass out"=w2288:refnum<class "CS.lvclass">, "error out"=w2289:errorcluster)  [unwired: 12 in]
            n1629 = case shown="True" w2287 {
              selector: w2287 -> [_ w2292]
              frame False {
              }
              frame True {
                n1630 = property on="_CurrentsChanged" class="Bool (strict)"("Val(Sgnl)"=w2292) -> ()  [unwired: 2 in, 2 out]
              }
            }
            n1631 = local write "_CSClassRef"(w2288) -> ()
            n1632 = property on="CS status" class="Clust (strict)"("Value"=w2289) -> ()  [unwired: 2 in, 2 out]
          }
          frame #3 {
            n1633 = Wait (ms)(milliseconds to wait=100) -> ()  [unwired: 1 out]
          }
        }
        n1634 = local read "Stop"() -> (w2227:bool)
      }
      n1635 = while {
        stop <- w2140 stop-if-true
        # "zBridge status read-out"
        n1636 = property on="Bridge Type" class="Enum (strict)"() -> ("Value"=w2138:T60)  [unwired: 2 in, 2 out]
        n1637 = case shown="\"Impedance Bridge\"" w2138 {
          frame Default {
          }
          frame "Impedance Bridge" {
            n1638 = local read "_zBridgeDll"() -> (w2146:path)
            n1639 = local read "Bridge status"() -> (w2145:errorcluster)
            n1640 = call "ScanStatus.vi"("error in (no error)"=w2145, "zDll"=w2146) -> ("error out"=w2144:errorcluster, "Status"=w2142:i32, "Channel"=w2143:i32)  [unwired: 7 in]
            n1641 = local write "Bridge status"(w2144) -> ()
            n1642 = call "zBridge Format Status.vi"("Status"=w2142, "Channel"=w2143) -> ("Status"=→"zBridge.Scan Phase":T86, "Active channel"=→"zBridge.Active channel":T87)  [unwired: 2 in]
          }
        }
        n1643 = Wait (ms)(milliseconds to wait=u32 200) -> ()  [unwired: 1 out]
        n1644 = local read "Stop"() -> (w2140:bool)
      }
    }
  }
  n1645 = disable-structure shown="Disabled" {
    frame Disabled {
      w2307 = string[] ["Paste Data from Clipboard"] ("item names")
      (unwired) enum32{"Page 1"}."Page 1" ("Tab Control 4")
      n1646 = local read "CS.Automode Current"() -> (w2302:T23[])
      n1647 = local read "zBridge.Active Channels"() -> ()  [unwired: 1 in]
      n1648 = property on="Bridge Channel" class="DigNum (strict)"() -> ("Value"=w2295:i32)  [unwired: 2 in, 2 out]
      n1649 = local read item#-1() -> ()  [unwired: 1 out]
      n1650 = Index Array(array=w2302) -> (element #1=w2298:T23, element #2=w2299:T23, element #3=w2300:T23, element #4=w2301:T23)  [unwired: 4 in]
      n1651 = property class="XYGraph (strict)" props=["YScale", "Mapping Mode"]() -> ()  [unwired: 2 in, 3 out]
      n1652 = property on="I" class="DigNum (strict)"("Val(Sgnl)"=w2298) -> ()  [unwired: 2 in, 2 out]
      n1653 = property on="I" class="DigNum (strict)"("Val(Sgnl)"=w2299) -> ()  [unwired: 2 in, 2 out]
      n1654 = property on="I" class="DigNum (strict)"("Val(Sgnl)"=w2300) -> ()  [unwired: 2 in, 2 out]
      n1655 = property on="I" class="DigNum (strict)"("Val(Sgnl)"=w2301) -> ()  [unwired: 2 in, 2 out]
      n1656 = Insert Menu Items(4:4, 7:w2307, 8:w2307) -> ()  [unwired: 3 in, 3 out]
      n1657 = Equal?(y=w2295) -> (x = y?=w2294:bool)  [unwired: 1 in]
      n1658 = Equal?(x=w2295, y=-1) -> (x = y?=w2297:bool)
      n1659 = Or(x=w2294, y=w2297) -> ()  [unwired: 1 out]
      n1660 = property on="ON" class="Boolean (strict)"() -> ("Value"=w2314:bool)  [unwired: 2 in, 2 out]
      n1661 = control-ref of="zBridge.Active Channels"() -> ()  [unwired: 1 out]
      n1662 = Exclusive Or(1:w2314, 2:TRUE ("x")) -> (0:w2313:bool)
      n1663 = property on="Toggle ON/OFF" class="Bool (strict)"("Value"=w2313) -> ()  [unwired: 2 in, 2 out]
      n1664 = control-ref of="CS.Mode1.List"() -> (w2309:refnum<vi>)
      n1665 = property class="Arr (strict)"(reference=w2309) -> ("Index Values"=w2310:u32[])  [unwired: 1 in, 2 out]
      n1666 = Index Array(array=w2310) -> (element=w2311:u32)  [unwired: 1 in]
      n1667 = property on="Side Panel" class="TabCtl (strict)"() -> ("Pages"=w2315:refnum<vi>[])  [unwired: 2 in, 2 out]
      n1668 = property on="CS.Mode1.List:Index" class="DigNum (strict)"("Val(Sgnl)"=w2311) -> ()  [unwired: 2 in, 2 out]
      n1669 = Index Array(array=w2315, index=1) -> (element=w2316:refnum<vi>)
      n1670 = Generate User Event(event data cluster="" ("event data")) -> ()  [unwired: 3 in, 2 out]
      n1671 = property class="Page"(reference=w2316, "PageVis"=TRUE ("Page Visible")) -> ()  [unwired: 1 in, 2 out]
      n1672 = property on="FB on" class="Enum (strict)" props=["Value"]() -> ()  [unwired: 2 in, 3 out]
      n1673 = Initialize Array(0.0 ("element"), 4 ("dimension size")) -> (w2303:dbl[])
      n1674 = local write "CS.Automode Current"(w2303) -> ()
    }
    frame Enabled {
    }
  }
